vi "Omniax_mDrive_XYZR_MM_BR_RES_2_NC_GR.vi"() -> ()   [LabVIEW 2009]
uses:
  <vilib>/Instr/_visa.llb/VISA Configure Serial Port (Instr).vi
panel:
  out "XY Graph 2":cluster{"Y":dbl[], "Y":dbl[]}[](graph)
  out "XY Graph":cluster{"Y":dbl[], "Y":dbl[]}[](graph)
  out "X Scan Duration":dbl
  out "Y Scan Duration":dbl
  out "Z Scan Duration":dbl
  out "R Scan Duration":dbl
  out "R Backlash steps/sec":i32
  out "R Backlash":i32
  out "R Holding Current %":i32
  out "R Run Current %":i32
  out "R offset deg":dbl
  out "R deg/rev":dbl
  out "R steps/rev":u32
  out "R velocity PV step/sec":i32
  out "R MINPOS":i32=-94296
  out "R MAXPOS":i32=-34296
  out "R COM PORT":refnum<visa-resource-name>="COM5"
  in  "R Scan set":bool
  in  "R Scan Velocity SP deg/sec":dbl
  in  "R Scan Length SP deg":dbl
  in  "R Move Set":bool
  out "Reset R Motor Steps":i32
  in  "Reset R Position deg":dbl
  out "R Velocity MVdeg/sec":dbl
  in  "R Velocity SP deg/sec":dbl
  in  "R Position SP deg":dbl
  out "R Position MV deg":dbl
  out "R Scan velocity MV deg/sec":dbl format="%#_6f"
  out "R Scan length MV deg":dbl
  in  "R Scan Length SP steps":i32 min=0 max=6144000 step=100
  in  "R Scan OK":bool
  in  "R Velocity SP step/sec":i32 min=1 max=102400
  in  "R Scan Velocity SP steps/sec":i32=1 min=1 max=102400 step=1
  in  "R Go":bool
  in  "R Step SP":i32=-20000 min=0 max=6144000 step=500
  out "R Position deg PV":dbl
  out "R Step PV":i32 max=2000
  out "R Backlash corr":bool
  out "R in Motion":bool
  out "R Scan":bool
  out "R in Range":bool
  out "Z COM PORT":refnum<visa-resource-name>="COM5"
  out "Z Backlash steps/sec":i32
  out "Z Backlash":i32
  out "Z Holding Current %":i32
  out "Z Run Current %":i32
  out "Z offset mm":dbl
  out "Z mm/rev":dbl
  out "Z steps/rev":u32
  out "Z  velocity PV step/sec":i32
  out "Z MINPOS":i32=-94296
  out "Z MAXPOS":i32=-34296
  in  "Z Scan set":bool
  in  "Z Scan Velocity SP mm/sec":dbl
  in  "Z Scan Length SP mm":dbl
  in  "Z Move Set":bool
  out "Reset Z Motor Steps":i32
  in  "Reset Z Position mm":dbl
  out "Z Velocity MV mm/sec":dbl
  in  "Z Velocity SP mm/sec":dbl
  in  "Z Position SP mm":dbl
  out "Z Position MV mm":dbl
  out "Z Scan velocity MV mm/sec":dbl format="%#_6f"
  out "Z Scan length MV mm":dbl
  in  "Z Scan Length SP steps":i32 min=0 max=2048000 step=100
  in  "Z Scan OK":bool
  in  "Z Velocity SP step/sec":i32 min=1 max=102400
  in  "Z Scan Velocity SP steps/sec":i32=1 min=1 max=102400 step=1
  in  "Z Go":bool
  in  "Z Step SP":i32=-20000 min=0 max=2048000 step=500
  out "Z Position mm PV":dbl
  out "Z Step PV":i32 max=2000
  out "Z Backlash corr":bool
  out "Z in Motion":bool
  out "Z Scan":bool
  out "Z in Range":bool
  out "Reset X Motor Steps":i32
  in  "Reset X Position mm":dbl
  out "X Backlash corr":bool
  out "X  in Motion":bool
  out "X Scan":bool
  out "X  in Range":bool
  out "X Step PV":i32 max=2000
  out "X Position mm PV":dbl
  out "X velocity PV step/sec":i32
  in  "X Scan set":bool
  in  "X Scan Velocity SP mm/sec":dbl
  in  "X Scan Length SP mm":dbl
  in  "X Move Set":bool
  out "X Velocity MV mm/sec":dbl
  in  "X Velocity SP mm/sec":dbl
  in  "X Position SP mm":dbl
  out "X Position MV mm":dbl
  out "X Scan velocity MV mm/sec":dbl format="%#_6f"
  out "X Scan length MV mm":dbl
  in  "X Scan Length SP steps":i32 min=-460800 max=460800 step=100
  in  "X Scan OK":bool
  in  "X Velocity SP step/sec":i32 min=1 max=102400
  in  "X Scan Velocity SP steps/sec":i32=1 min=1 max=102400 step=1
  in  "X Go":bool
  in  "X Step SP":i32=-20000 min=-460800 max=460800 step=500
  out "X Backlash steps/sec":i32
  out "X Backlash":i32
  out "X Holding Current %":i32
  out "X Run Current %":i32
  out "X offset mm":dbl
  out "X mm/rev":dbl
  out "X steps/rev":u32
  out "X MAXPOS":i32=-34296
  out "X MINPOS":i32=-94296
  out "X COM PORT":refnum<visa-resource-name>="COM5"
  out "Y Backlash corr":bool
  in  "Y Scan set":bool
  in  "Y Scan Velocity SP mm/sec":dbl
  in  "Y Scan Length SP mm":dbl
  in  "Y Move Set":bool
  out "Y Backlash steps/sec":i32
  out "Y Backlash":i32
  out "Y in Motion":bool
  in  "Reset":bool
  out "Reset Y Motor Steps":i32
  in  "Reset Y Position mm":dbl
  out "Y Velocity MV mm/sec":dbl
  in  "Y Velocity SP mm/sec":dbl
  in  "Y Position SP mm":dbl
  out "Y Position MV mm":dbl
  out "Y Holding Current %":i32
  out "Y Run Current %":i32
  out "Y Scan velocity MV mm/sec":dbl format="%#_6f"
  out "Y Scan length MV mm":dbl
  in  "Scan Cancel":bool
  out "Y Position mm PV":dbl
  out "Y offset mm":dbl
  out "Y mm/rev":dbl
  out "Y steps/rev":u32
  out "Y velocity PV step/sec":i32
  in  "Y Scan Length SP steps":i32 min=-460800 max=460800 step=100
  out "Y Scan":bool
  in  "Y Scan OK":bool
  in  "Scan Go":bool
  in  "Y Velocity SP step/sec":i32 min=1 max=102400
  in  "Y Scan Velocity SP steps/sec":i32=1 min=1 max=102400 step=1
  in  "Stop":bool
  out "Y in Range":bool
  out "Y Step PV":i32 max=2000
  in  "Y Go":bool
  in  "Y Step SP":i32=-20000 min=-460800 max=460800 step=500
  out "Y MINPOS":i32=-94296
  out "Y MAXPOS":i32=-34296
  out "Y COM PORT":refnum<visa-resource-name>="COM5"
  # "L"
  # "M"
  # "B"
  # "S"
  # "MX"
  # "MY"
  # "MZ"
  # "MR"
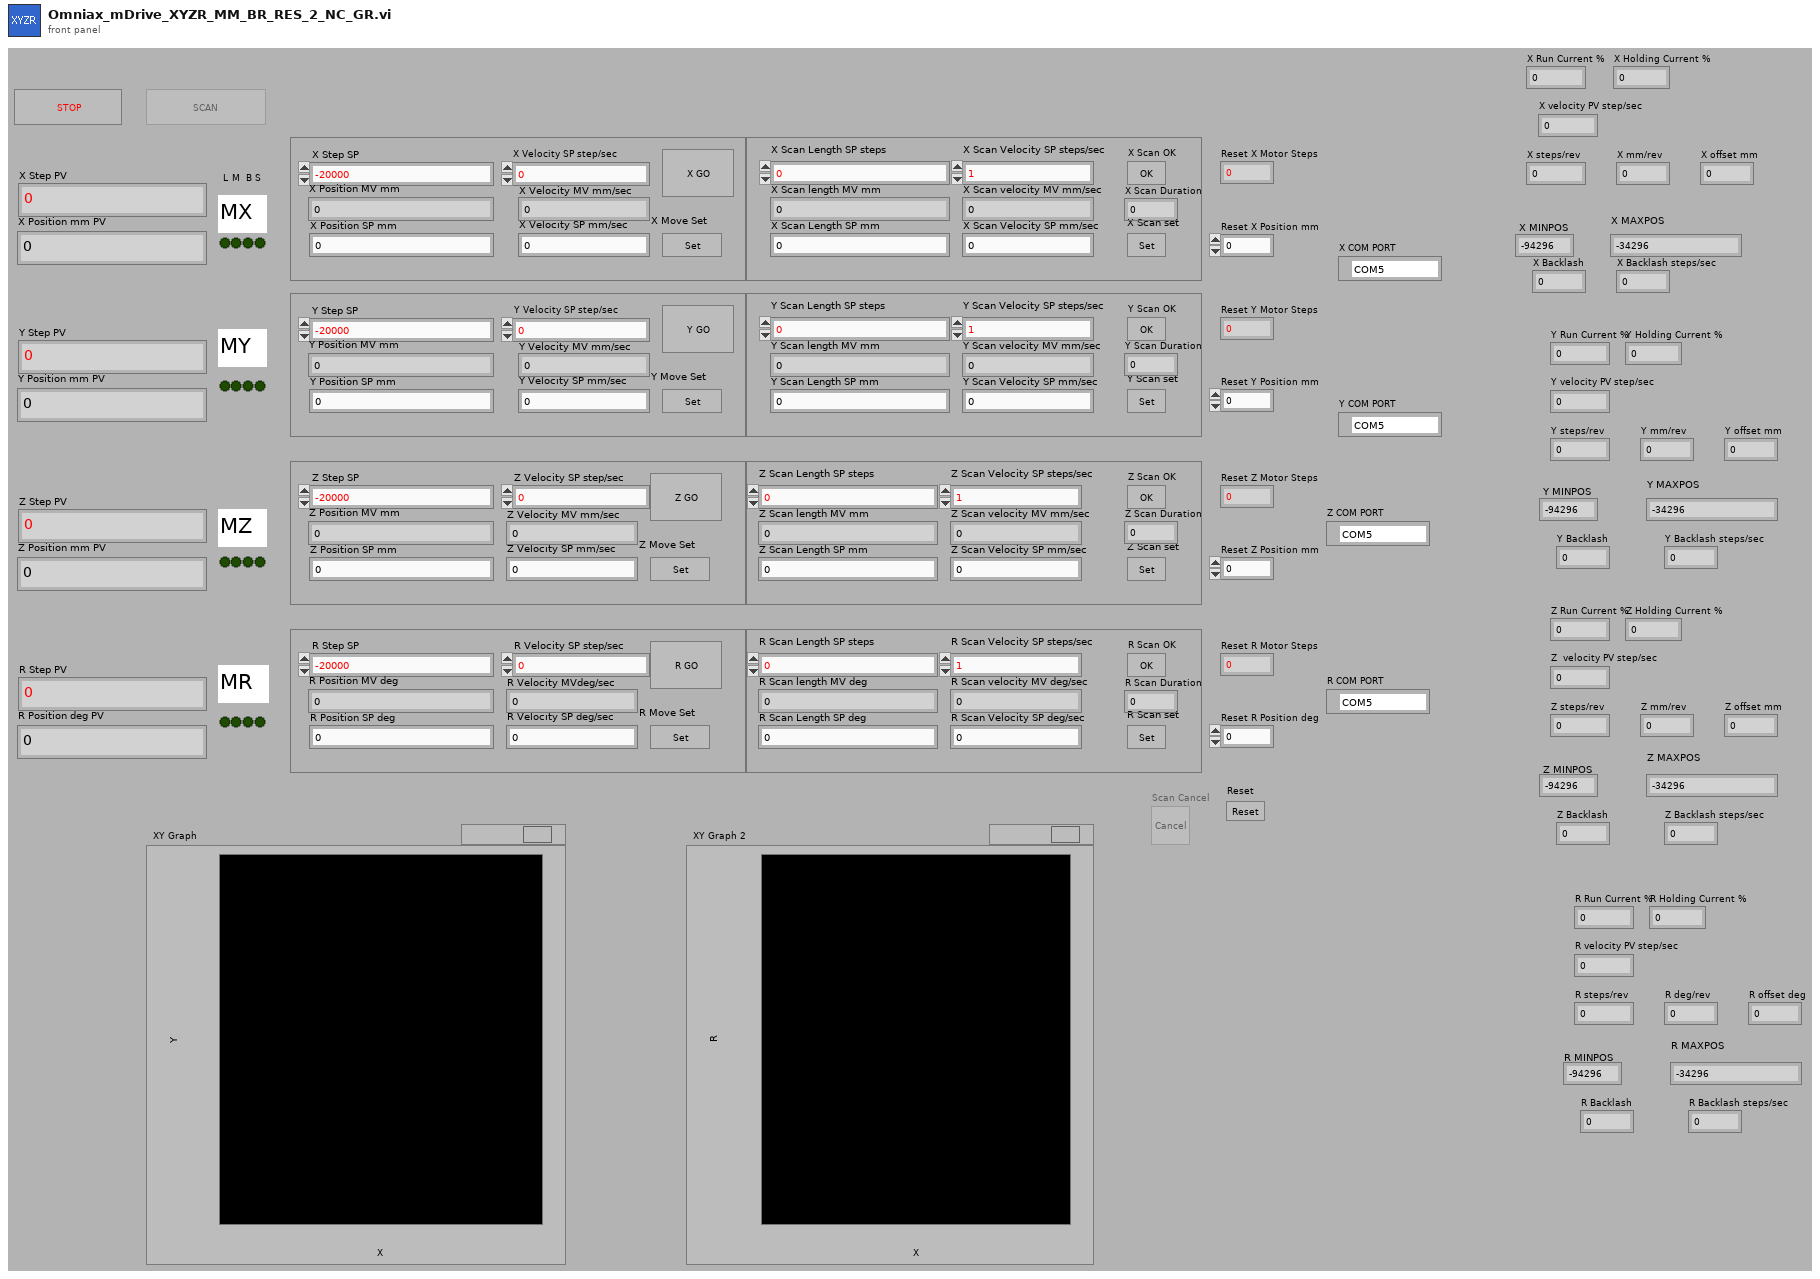
[diagram p1: front panel]
types:
  T1 = enum8{"Enabled", "Disabled", "Disabled and Grayed Out"}
  T2 = enum16{"Stop", "Reset", "Run Current", "Holding Current", "Accel Rate", "Decel Rate", "Move to Relative Position", "Move to Absolute Position", "Echo Mode", "Print Parameter", "Send String", "Microstep Resolution", "Set Current Position", "Max Velocity"}
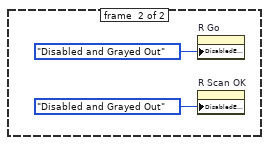
[diagram p2: hidden frame]
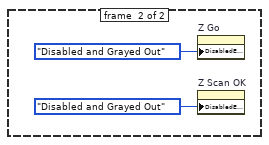
[diagram p5: hidden frame]
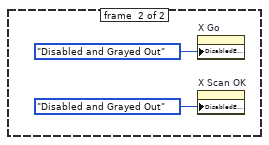
[diagram p8: hidden frame]
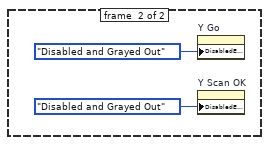
[diagram p11: hidden frame]
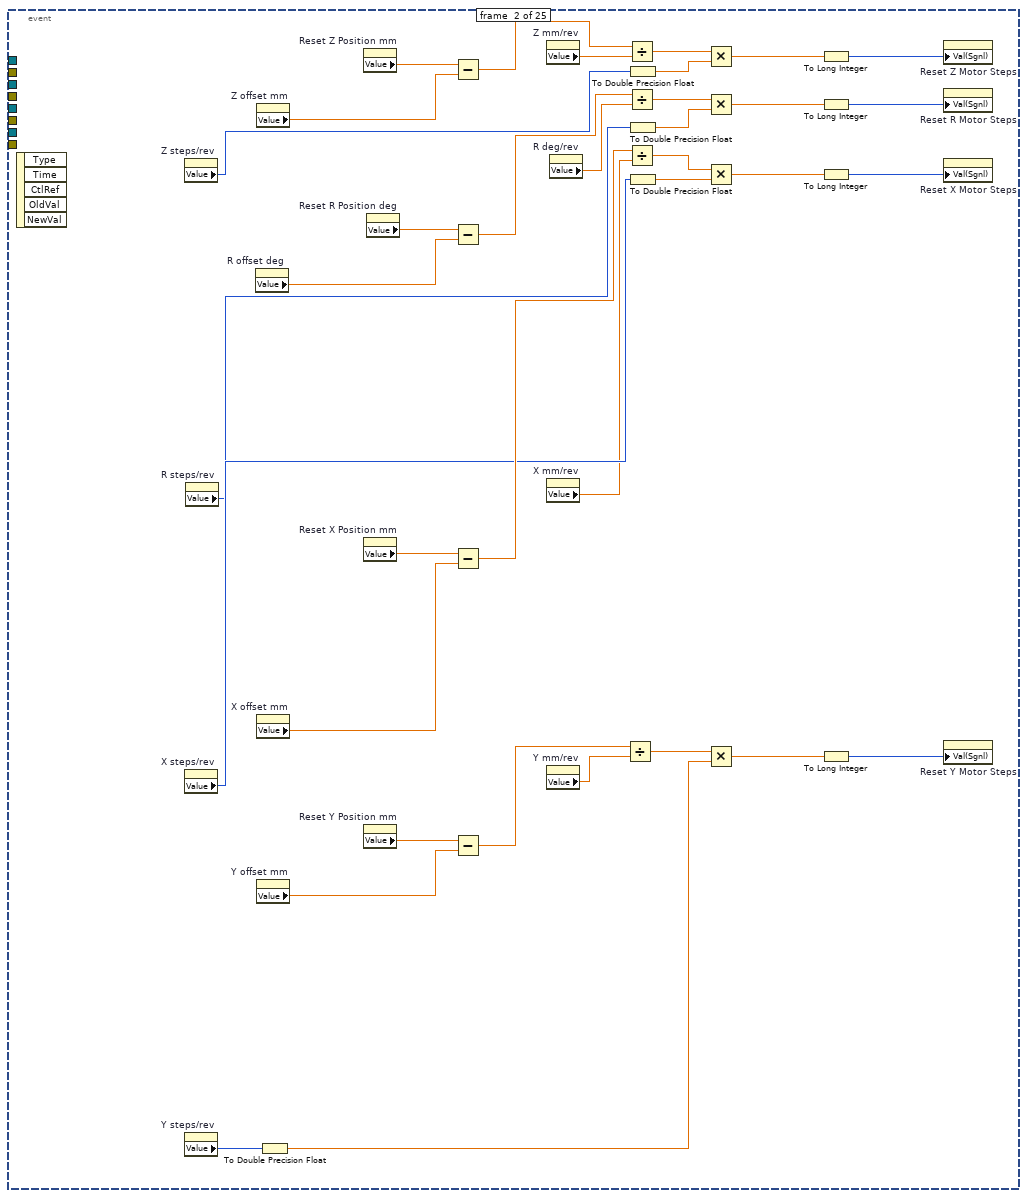
[diagram p14: hidden frame]
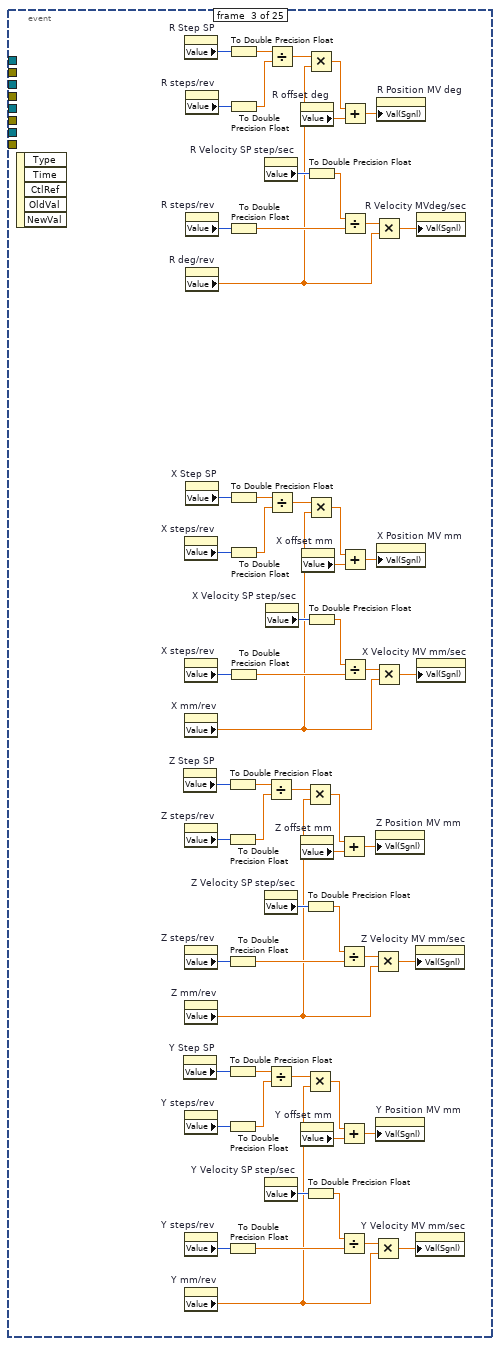
[diagram p15: hidden frame]
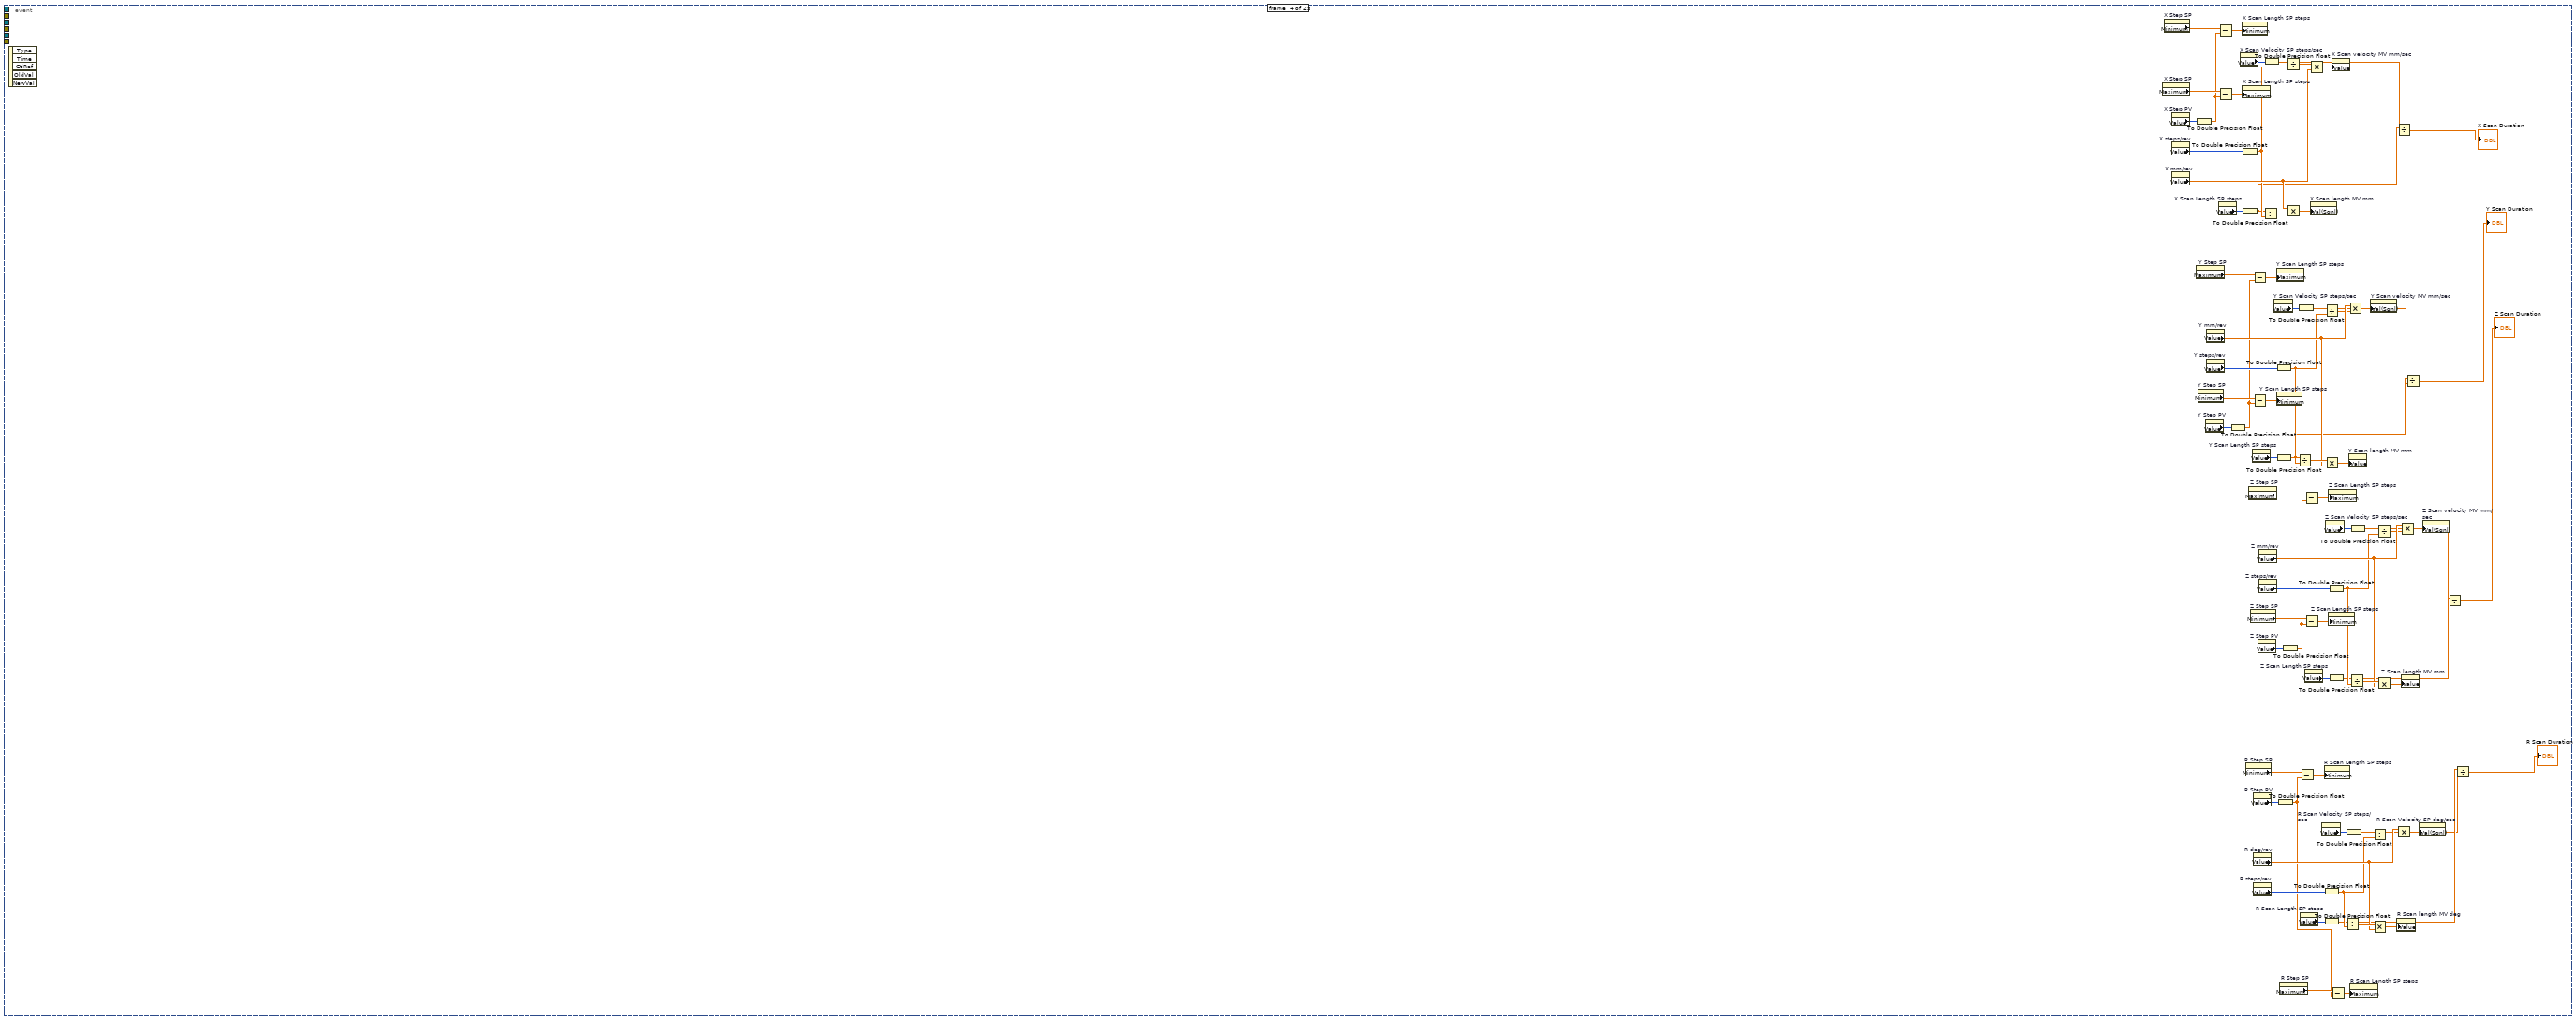
[diagram p16: hidden frame]
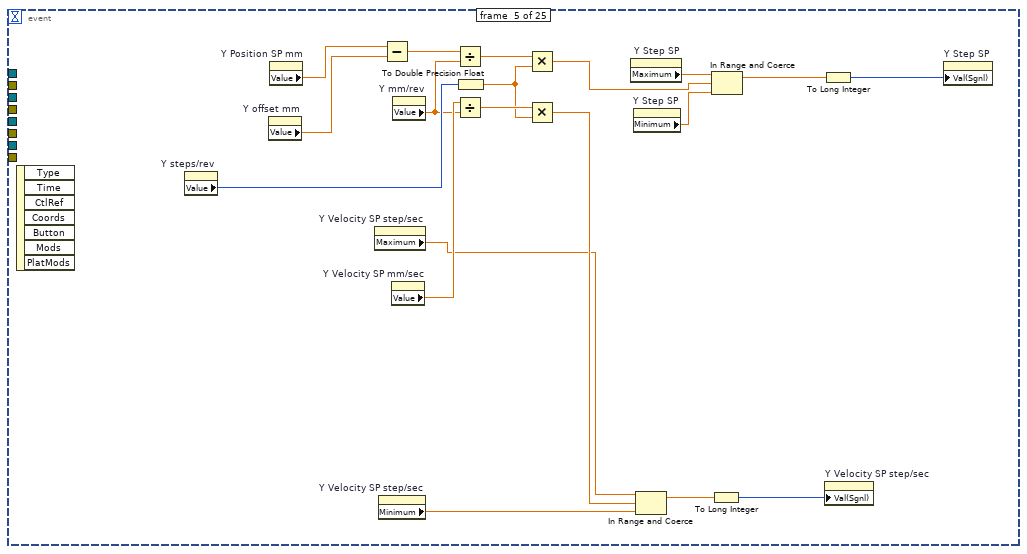
[diagram p17: hidden frame]
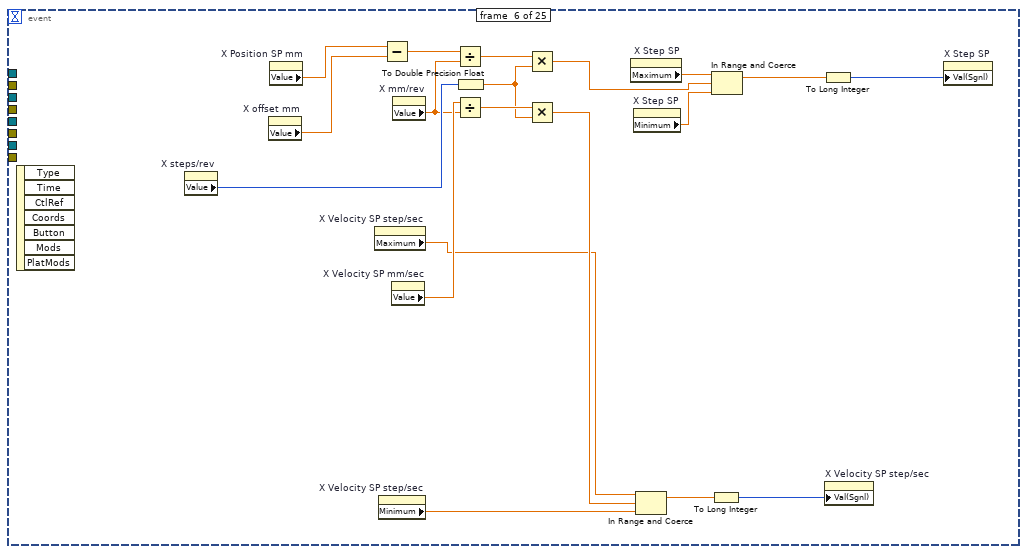
[diagram p18: hidden frame]
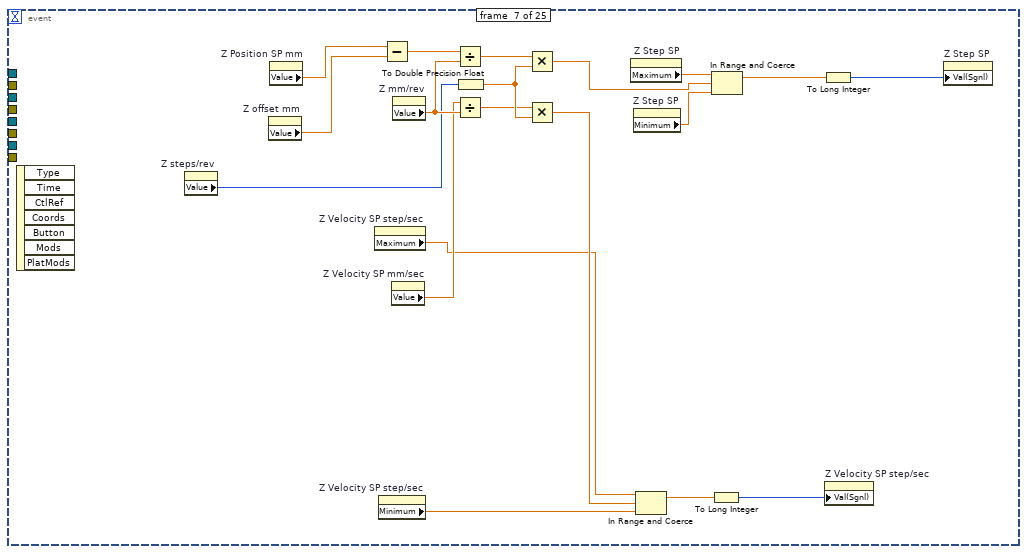
[diagram p19: hidden frame]
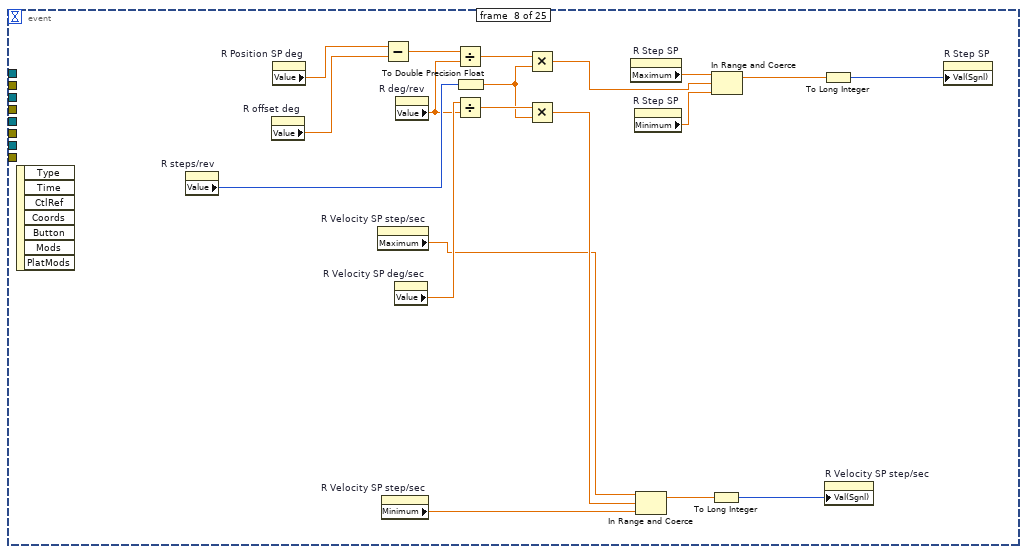
[diagram p20: hidden frame]
diagram:
  w19 = refnum<visa-resource-name> "COM11" ("COM PORT")
  w21 = u16 0 items=["None", "XON/XOFF", "RTS/CTS", "XON/XOFF & RTS/CTS", "DTR/DSR", "XON/XOFF & DTR/DSR"] ("flow control (0:none)")
  w22 = u16 10 items=["1.0"=10, "1.5"=15, "2.0"=20] ("stop bits (10: 1 bit)")
  w52 = refnum<visa-resource-name> "COM10" ("COM PORT")
  w54 = u16 0 items=["None", "XON/XOFF", "RTS/CTS", "XON/XOFF & RTS/CTS", "DTR/DSR", "XON/XOFF & DTR/DSR"] ("flow control (0:none)")
  w55 = u16 10 items=["1.0"=10, "1.5"=15, "2.0"=20] ("stop bits (10: 1 bit)")
  w65 = refnum<visa-resource-name> "COM8" ("COM PORT")
  w67 = u16 0 items=["None", "XON/XOFF", "RTS/CTS", "XON/XOFF & RTS/CTS", "DTR/DSR", "XON/XOFF & DTR/DSR"] ("flow control (0:none)")
  w68 = u16 10 items=["1.0"=10, "1.5"=15, "2.0"=20] ("stop bits (10: 1 bit)")
  w90 = refnum<visa-resource-name> "COM9" ("COM PORT")
  w92 = u16 0 items=["None", "XON/XOFF", "RTS/CTS", "XON/XOFF & RTS/CTS", "DTR/DSR", "XON/XOFF & DTR/DSR"] ("flow control (0:none)")
  w93 = u16 10 items=["1.0"=10, "1.5"=15, "2.0"=20] ("stop bits (10: 1 bit)")
  # "Stop bits"
  # "Stop bits"
  # "Stop bits"
  # "Stop bits"
  n1 = flat-sequence {
    frame #0 {
      w101 = 3.0 ("R deg/rev")
      w99 = u32 51200 ("step/rev")
      w103 = 102400 ("Value (Signaling)")
      n2 = property on="R Velocity SP step/sec" class="DigNum (strict)"("Val(Sgnl)"=w103) -> ()  [unwired: 2 in, 2 out]
      n3 = property on="R Velocity SP step/sec" class="DigNum (strict)"("Minimum"=1.0 ("Data Entry Limits:Minimum")) -> ()  [unwired: 2 in, 2 out]
      n4 = To Double Precision Float(number=w99) -> (double precision float=w100:dbl)
      n5 = To Double Precision Float(number=w103) -> (double precision float=w105:dbl)
      n6 = Divide(x=w105, y=w100) -> (x/y=w104:dbl)
      n7 = property on="R Velocity SP step/sec" class="DigNum (strict)"("Maximum"=w105) -> ()  [unwired: 2 in, 2 out]
      n8 = Multiply(x=w104, y=w101) -> (x*y=w102:dbl)
      n9 = property on="R Velocity SP deg/sec" class="DigNum (strict)"("Val(Sgnl)"=w102) -> ()  [unwired: 2 in, 2 out]
      "R offset deg" <- 0.0 ("R offset deg")
      "R deg/rev" <- w101
      "R steps/rev" <- w99
    }
  }
  n10 = flat-sequence {
    frame #0 {
      w108 = 1.0 ("MM/rev")
      w111 = u32 51200 ("step/rev")
      w106 = 102400 ("Value (Signaling)")
      n11 = property on="X Velocity SP step/sec" class="DigNum (strict)"("Minimum"=1.0 ("Data Entry Limits:Minimum")) -> ()  [unwired: 2 in, 2 out]
      n12 = property on="X Velocity SP step/sec" class="DigNum (strict)"("Val(Sgnl)"=w106) -> ()  [unwired: 2 in, 2 out]
      n13 = To Double Precision Float(number=w111) -> (double precision float=w110:dbl)
      n14 = To Double Precision Float(number=w106) -> (double precision float=w112:dbl)
      n15 = Divide(x=w112, y=w110) -> (x/y=w107:dbl)
      n16 = property on="X Velocity SP step/sec" class="DigNum (strict)"("Maximum"=w112) -> ()  [unwired: 2 in, 2 out]
      n17 = Multiply(x=w107, y=w108) -> (x*y=w109:dbl)
      n18 = property on="X Velocity SP mm/sec" class="DigNum (strict)"("Val(Sgnl)"=w109) -> ()  [unwired: 2 in, 2 out]
      "X offset mm" <- 0.0 ("offset")
      "X steps/rev" <- w111
      "X mm/rev" <- w108
    }
  }
  n19 = flat-sequence {
    frame #0 {
      w116 = 1.0 ("Z mm/rev")
      w115 = u32 51200 ("step/rev")
      w117 = 102400 ("Value (Signaling)")
      n20 = property on="Z Velocity SP step/sec" class="DigNum (strict)"("Val(Sgnl)"=w117) -> ()  [unwired: 2 in, 2 out]
      n21 = property on="Z Velocity SP step/sec" class="DigNum (strict)"("Minimum"=1.0 ("Data Entry Limits:Minimum")) -> ()  [unwired: 2 in, 2 out]
      n22 = To Double Precision Float(number=w115) -> (double precision float=w120:dbl)
      n23 = To Double Precision Float(number=w117) -> (double precision float=w121:dbl)
      n24 = Divide(x=w121, y=w120) -> (x/y=w118:dbl)
      n25 = property on="Z Velocity SP step/sec" class="DigNum (strict)"("Maximum"=w121) -> ()  [unwired: 2 in, 2 out]
      n26 = Multiply(x=w118, y=w116) -> (x*y=w119:dbl)
      n27 = property on="Z Velocity SP mm/sec" class="DigNum (strict)"("Val(Sgnl)"=w119) -> ()  [unwired: 2 in, 2 out]
      "Z offset mm" <- 0.0 ("Z offset mm")
      "Z mm/rev" <- w116
      "Z steps/rev" <- w115
    }
  }
  n28 = flat-sequence {
    frame #0 {
      n29 = property on="X Backlash corr" class="Bool (strict)"("Val(Sgnl)"=FALSE ("Value (Signaling)")) -> ()  [unwired: 2 in, 2 out]
      n30 = property on="Z Backlash corr" class="Bool (strict)"("Val(Sgnl)"=FALSE ("Value (Signaling)")) -> ()  [unwired: 2 in, 2 out]
      n31 = property on="Y Backlash corr" class="Bool (strict)"("Val(Sgnl)"=FALSE ("Value (Signaling)")) -> ()  [unwired: 2 in, 2 out]
      n32 = property on="R Backlash corr" class="Bool (strict)"("Val(Sgnl)"=FALSE ("Value (Signaling)")) -> ()  [unwired: 2 in, 2 out]
      "Z Backlash steps/sec" <- 25600 ("Z Backlash steps/sec")
      "Z Backlash" <- -12800 ("Z Backlash")
      "X Backlash steps/sec" <- 25600 ("Value (Signaling)")
      "X Backlash" <- -5120 ("Backlash2")
      "Y Backlash" <- -5120 ("Backlash2")
      "Y Backlash steps/sec" <- 25600 ("Value (Signaling)")
      "R Backlash steps/sec" <- 25600 ("R Backlash steps/sec")
      "R Backlash" <- -12800 ("R Backlash")
    }
  }
  n33 = flat-sequence {
    frame #0 {
      "Z Holding Current %" <- 20 ("Z Holding Current %")
      "Z Run Current %" <- 40 ("Z Run Current %")
      "X Run Current %" <- 40 ("Run Current %")
      "X Holding Current %" <- 20 ("Holding Current %")
      "Y Run Current %" <- 40 ("Run Current %")
      "Y Holding Current %" <- 20 ("Holding Current %")
      "R Holding Current %" <- 20 ("R Holding Current %")
      "R Run Current %" <- 40 ("R Run Current %")
    }
  }
  n34 = flat-sequence {
    frame #0 {
      n35 = property on="Y Scan" class="Bool (strict)"("Val(Sgnl)"=FALSE ("Value (Signaling)")) -> ()  [unwired: 2 in, 2 out]
      n36 = property on="Y Scan Velocity SP mm/sec" class="DigNum (strict)"("Val(Sgnl)"=0.1 ("Value (Signaling)")) -> ()  [unwired: 2 in, 2 out]
      n37 = property on="Z Scan Velocity SP mm/sec" class="DigNum (strict)"("Val(Sgnl)"=0.1 ("Value (Signaling)")) -> ()  [unwired: 2 in, 2 out]
      n38 = property on="R Scan" class="Bool (strict)"("Val(Sgnl)"=FALSE ("Value (Signaling)")) -> ()  [unwired: 2 in, 2 out]
      n39 = property on="Z Scan" class="Bool (strict)"("Val(Sgnl)"=FALSE ("Value (Signaling)")) -> ()  [unwired: 2 in, 2 out]
      n40 = property on="R Velocity SP deg/sec" class="DigNum (strict)"("Val(Sgnl)"=0.1 ("Value (Signaling)")) -> ()  [unwired: 2 in, 2 out]
      n41 = property on="X Scan" class="Bool (strict)"("Val(Sgnl)"=FALSE ("Value (Signaling)")) -> ()  [unwired: 2 in, 2 out]
      n42 = property on="X Scan Velocity SP mm/sec" class="DigNum (strict)"("Val(Sgnl)"=0.1 ("Value (Signaling)")) -> ()  [unwired: 2 in, 2 out]
      n43 = property on="Scan Go" class="Bool"("DisabledEnum"=T1."Disabled and Grayed Out" ("Disabled")) -> ()  [unwired: 2 in, 2 out]
      n44 = property on="Scan Cancel" class="Bool"("DisabledEnum"=T1."Disabled and Grayed Out" ("Disabled")) -> ()  [unwired: 2 in, 2 out]
    }
  }
  n45 = flat-sequence {
    frame #0 {
      w156 = 1.0 ("MM/rev")
      w159 = u32 51200 ("step/rev")
      w154 = 102400 ("Value (Signaling)")
      n46 = property on="Y Velocity SP step/sec" class="DigNum (strict)"("Minimum"=1.0 ("Data Entry Limits:Minimum")) -> ()  [unwired: 2 in, 2 out]
      n47 = property on="Y Velocity SP step/sec" class="DigNum (strict)"("Val(Sgnl)"=w154) -> ()  [unwired: 2 in, 2 out]
      n48 = To Double Precision Float(number=w159) -> (double precision float=w158:dbl)
      n49 = To Double Precision Float(number=w154) -> (double precision float=w160:dbl)
      n50 = Divide(x=w160, y=w158) -> (x/y=w155:dbl)
      n51 = property on="Y Velocity SP step/sec" class="DigNum (strict)"("Maximum"=w160) -> ()  [unwired: 2 in, 2 out]
      n52 = Multiply(x=w155, y=w156) -> (x*y=w157:dbl)
      n53 = property on="Y Velocity SP mm/sec" class="DigNum (strict)"("Val(Sgnl)"=w157) -> ()  [unwired: 2 in, 2 out]
      "Y offset mm" <- 0.0 ("offset")
      "Y steps/rev" <- w159
      "Y mm/rev" <- w156
    }
  }
  n54 = call-poly "VISA Configure Serial Port"("VISA resource name"=w90, "timeout (10sec)"=u32 10000, "baud rate (9600)"=u32 9600, "data bits (8)"=u16 8, "parity (0:none)"=enum16{"None", "Odd", "Even", "Mark", "Space"}."None", "stop bits (10: 1 bit)"=w93, "flow control (0:none)"=w92) -> ("VISA resource name out"=w83:refnum<visa-resource-name>, "error out"=w82:errorcluster)  [unwired: 7 in]
  n55 = flat-sequence {
    tunnel: w82 -> [w164]
    tunnel: w83 -> [w166]
    tunnel: [w165] -> w4
    tunnel: [w163] -> w3
    tunnel: [w172] -> w81
    tunnel: [w174] -> w79
    tunnel: w4 -> [w173]
    tunnel: w3 -> [w175]
    tunnel: w81 -> [w182]
    tunnel: [w181] -> w80
    tunnel: w79 -> [w179]
    tunnel: [w180] -> w78
    tunnel: [w192] -> w85
    tunnel: [w193] -> w84
    tunnel: w80 -> [w191]
    tunnel: w78 -> [w190]
    tunnel: w85 -> [w203]
    tunnel: w84 -> [w202]
    tunnel: [w205] -> w51
    tunnel: [w204] -> w50
    tunnel: [w199] -> w49
    tunnel: [w210] -> w88
    tunnel: [w211] -> w89
    tunnel: w51 -> [w211]
    tunnel: w50 -> [w210]
    tunnel: w49 -> [w206]
    frame #0 {
      n56 = call "mDrive Send Command.vi"("error in (no error)"=w164, "Extra"="EM=2", "Command"=T2."Send String", "VISA resource name"=w166) -> ("error out"=w163:errorcluster, "VISA resource name out"=w165:refnum<visa-resource-name>)  [unwired: 3 in, 1 out]
    }
    frame #1 {
      # "Run Current %"
      n57 = property on="Y Run Current %" class="DigNum (strict)"() -> ("Value"=w170:i32)  [unwired: 2 in, 2 out]
      n58 = Number To Decimal String(number=w170) -> (decimal integer string=w171:string)  [unwired: 1 in]
      n59 = call "mDrive Send Command.vi"("error in (no error)"=w175, "Extra"=w171, "Command"=T2."Run Current", "VISA resource name"=w173) -> ("error out"=w174:errorcluster, "VISA resource name out"=w172:refnum<visa-resource-name>)  [unwired: 3 in, 1 out]
    }
    frame #2 {
      # "Holding Current %"
      n60 = property on="Y Holding Current %" class="DigNum (strict)"() -> ("Value"=w177:i32)  [unwired: 2 in, 2 out]
      n61 = Number To Decimal String(number=w177) -> (decimal integer string=w178:string)  [unwired: 1 in]
      n62 = call "mDrive Send Command.vi"("error in (no error)"=w179, "Extra"=w178, "Command"=T2."Holding Current", "VISA resource name"=w182) -> ("error out"=w180:errorcluster, "VISA resource name out"=w181:refnum<visa-resource-name>)  [unwired: 3 in, 1 out]
    }
    frame #3 {
      # "Print Velocity Ma"
      # "Velocity Max"
      n63 = property on="Y Velocity SP step/sec" class="DigNum (strict)"() -> ("Value"=w189:i32)  [unwired: 2 in, 2 out]
      n64 = Number To Decimal String(number=w189) -> (decimal integer string=w188:string)  [unwired: 1 in]
      n65 = call "mDrive Send Command.vi"("error in (no error)"=w190, "Extra"=w188, "Command"=T2."Max Velocity", "VISA resource name"=w191) -> ("error out"=w186:errorcluster, "VISA resource name out"=w196:refnum<visa-resource-name>)  [unwired: 3 in, 1 out]
      n66 = call "mDrive Send Command.vi"("error in (no error)"=w186, "Extra"="VM", "Command"=T2."Print Parameter", "VISA resource name"=w196) -> ("error out"=w193:errorcluster, "read buffer"=w194:string, "VISA resource name out"=w192:refnum<visa-resource-name>)  [unwired: 3 in]
      n67 = Decimal String To Number(string=w194, offset=0) -> (number=w187:i32)  [unwired: 1 in, 1 out]
      n68 = property on="Y scan velocity MV step/sec" class="DigNum (strict)"("Val(Sgnl)"=w187) -> ()  [unwired: 2 in, 2 out]
    }
    frame #4 {
      # "PRINT POSITION"
      n69 = call "mDrive Send Command.vi"("error in (no error)"=w202, "Extra"="P", "Command"=T2."Print Parameter", "VISA resource name"=w203) -> ("error out"=w204:errorcluster, "read buffer"=w201:string, "VISA resource name out"=w205:refnum<visa-resource-name>)  [unwired: 3 in]
      n70 = Decimal String To Number(string=w201, offset=0) -> (number=w199:i32)  [unwired: 1 in, 1 out]
    }
    frame #5 {
      w208 = -460800 ("lower limit")
      w209 = 460800 ("upper limit")
      n71 = property on="Y Step SP" class="DigNum (strict)"("Val(Sgnl)"=w206) -> ()  [unwired: 2 in, 2 out]
      n72 = property on="Y Step SP" class="DigNum (strict)"("Maximum"=w209) -> ()  [unwired: 2 in, 2 out]
      n73 = property on="Y Step SP" class="DigNum (strict)"("Minimum"=w208) -> ()  [unwired: 2 in, 2 out]
      n74 = In Range and Coerce(upper limit=w209, x=w206, lower limit=w208) -> (In Range?=w207:bool)  [unwired: 1 out]
      n75 = property on="Y in Range" class="Bool (strict)"("Val(Sgnl)"=w207) -> ()  [unwired: 2 in, 2 out]
      "Y MINPOS" <- w208
      "Y MAXPOS" <- w209
    }
  }
  n76 = call-poly "VISA Configure Serial Port"("VISA resource name"=w65, "timeout (10sec)"=u32 10000, "baud rate (9600)"=u32 9600, "data bits (8)"=u16 8, "parity (0:none)"=enum16{"None", "Odd", "Even", "Mark", "Space"}."None", "stop bits (10: 1 bit)"=w68, "flow control (0:none)"=w67) -> ("VISA resource name out"=w64:refnum<visa-resource-name>, "error out"=w63:errorcluster)  [unwired: 7 in]
  n77 = call-poly "VISA Configure Serial Port"("VISA resource name"=w19, "timeout (10sec)"=u32 10000, "baud rate (9600)"=u32 9600, "data bits (8)"=u16 8, "parity (0:none)"=enum16{"None", "Odd", "Even", "Mark", "Space"}."None", "stop bits (10: 1 bit)"=w22, "flow control (0:none)"=w21) -> ("VISA resource name out"=w18:refnum<visa-resource-name>, "error out"=w17:errorcluster)  [unwired: 7 in]
  n78 = call-poly "VISA Configure Serial Port"("VISA resource name"=w52, "timeout (10sec)"=u32 10000, "baud rate (9600)"=u32 9600, "data bits (8)"=u16 8, "parity (0:none)"=enum16{"None", "Odd", "Even", "Mark", "Space"}."None", "stop bits (10: 1 bit)"=w55, "flow control (0:none)"=w54) -> ("VISA resource name out"=w36:refnum<visa-resource-name>, "error out"=w35:errorcluster)  [unwired: 7 in]
  n79 = flat-sequence {
    tunnel: w63 -> [w213]
    tunnel: w64 -> [w215]
    tunnel: [w214] -> w2
    tunnel: [w212] -> w1
    tunnel: [w221] -> w77
    tunnel: [w223] -> w76
    tunnel: w2 -> [w222]
    tunnel: w1 -> [w224]
    tunnel: w77 -> [w231]
    tunnel: [w230] -> w75
    tunnel: w76 -> [w228]
    tunnel: [w229] -> w74
    tunnel: [w241] -> w73
    tunnel: [w242] -> w72
    tunnel: w75 -> [w240]
    tunnel: w74 -> [w239]
    tunnel: w73 -> [w252]
    tunnel: w72 -> [w251]
    tunnel: [w254] -> w48
    tunnel: [w253] -> w47
    tunnel: [w248] -> w46
    tunnel: [w259] -> w61
    tunnel: [w260] -> w62
    tunnel: w48 -> [w260]
    tunnel: w47 -> [w259]
    tunnel: w46 -> [w255]
    frame #0 {
      n80 = call "mDrive Send Command.vi"("error in (no error)"=w213, "Extra"="EM=2", "Command"=T2."Send String", "VISA resource name"=w215) -> ("error out"=w212:errorcluster, "VISA resource name out"=w214:refnum<visa-resource-name>)  [unwired: 3 in, 1 out]
    }
    frame #1 {
      # "Run Current %"
      n81 = property on="X Run Current %" class="DigNum (strict)"() -> ("Value"=w219:i32)  [unwired: 2 in, 2 out]
      n82 = Number To Decimal String(number=w219) -> (decimal integer string=w220:string)  [unwired: 1 in]
      n83 = call "mDrive Send Command.vi"("error in (no error)"=w224, "Extra"=w220, "Command"=T2."Run Current", "VISA resource name"=w222) -> ("error out"=w223:errorcluster, "VISA resource name out"=w221:refnum<visa-resource-name>)  [unwired: 3 in, 1 out]
    }
    frame #2 {
      # "Holding Current %"
      n84 = property on="X Holding Current %" class="DigNum (strict)"() -> ("Value"=w226:i32)  [unwired: 2 in, 2 out]
      n85 = Number To Decimal String(number=w226) -> (decimal integer string=w227:string)  [unwired: 1 in]
      n86 = call "mDrive Send Command.vi"("error in (no error)"=w228, "Extra"=w227, "Command"=T2."Holding Current", "VISA resource name"=w231) -> ("error out"=w229:errorcluster, "VISA resource name out"=w230:refnum<visa-resource-name>)  [unwired: 3 in, 1 out]
    }
    frame #3 {
      # "Print Velocity Ma"
      # "Velocity Max"
      n87 = property on="X Velocity SP step/sec" class="DigNum (strict)"() -> ("Value"=w238:i32)  [unwired: 2 in, 2 out]
      n88 = Number To Decimal String(number=w238) -> (decimal integer string=w237:string)  [unwired: 1 in]
      n89 = call "mDrive Send Command.vi"("error in (no error)"=w239, "Extra"=w237, "Command"=T2."Max Velocity", "VISA resource name"=w240) -> ("error out"=w235:errorcluster, "VISA resource name out"=w245:refnum<visa-resource-name>)  [unwired: 3 in, 1 out]
      n90 = call "mDrive Send Command.vi"("error in (no error)"=w235, "Extra"="VM", "Command"=T2."Print Parameter", "VISA resource name"=w245) -> ("error out"=w242:errorcluster, "read buffer"=w243:string, "VISA resource name out"=w241:refnum<visa-resource-name>)  [unwired: 3 in]
      n91 = Decimal String To Number(string=w243, offset=0) -> (number=w236:i32)  [unwired: 1 in, 1 out]
      n92 = property on="X velocity PV step/sec" class="DigNum (strict)"("Val(Sgnl)"=w236) -> ()  [unwired: 2 in, 2 out]
    }
    frame #4 {
      # "PRINT POSITION"
      n93 = call "mDrive Send Command.vi"("error in (no error)"=w251, "Extra"="P", "Command"=T2."Print Parameter", "VISA resource name"=w252) -> ("error out"=w253:errorcluster, "read buffer"=w250:string, "VISA resource name out"=w254:refnum<visa-resource-name>)  [unwired: 3 in]
      n94 = Decimal String To Number(string=w250, offset=0) -> (number=w248:i32)  [unwired: 1 in, 1 out]
    }
    frame #5 {
      w257 = -460800 ("lower limit")
      w258 = 460800 ("upper limit")
      n95 = property on="X Step SP" class="DigNum (strict)"("Val(Sgnl)"=w255) -> ()  [unwired: 2 in, 2 out]
      n96 = property on="X Step SP" class="DigNum (strict)"("Maximum"=w258) -> ()  [unwired: 2 in, 2 out]
      n97 = property on="X Step SP" class="DigNum (strict)"("Minimum"=w257) -> ()  [unwired: 2 in, 2 out]
      n98 = In Range and Coerce(upper limit=w258, x=w255, lower limit=w257) -> (In Range?=w256:bool)  [unwired: 1 out]
      n99 = property on="X  in Range" class="Bool (strict)"("Val(Sgnl)"=w256) -> ()  [unwired: 2 in, 2 out]
      "X MINPOS" <- w257
      "X MAXPOS" <- w258
    }
  }
  n100 = flat-sequence {
    tunnel: w17 -> [w264]
    tunnel: w18 -> [w262]
    tunnel: [w261] -> w8
    tunnel: [w263] -> w7
    tunnel: [w271] -> w34
    tunnel: [w273] -> w33
    tunnel: w8 -> [w272]
    tunnel: w7 -> [w267]
    tunnel: w34 -> [w280]
    tunnel: [w279] -> w32
    tunnel: w33 -> [w277]
    tunnel: [w278] -> w31
    tunnel: [w290] -> w30
    tunnel: [w291] -> w29
    tunnel: w32 -> [w289]
    tunnel: w31 -> [w288]
    tunnel: w30 -> [w301]
    tunnel: w29 -> [w300]
    tunnel: [w303] -> w28
    tunnel: [w302] -> w27
    tunnel: [w297] -> w26
    tunnel: [w308] -> w11
    tunnel: [w309] -> w12
    tunnel: w28 -> [w309]
    tunnel: w27 -> [w308]
    tunnel: w26 -> [w306]
    frame #0 {
      n101 = call "mDrive Send Command.vi"("error in (no error)"=w264, "Extra"="EM=2", "Command"=T2."Send String", "VISA resource name"=w262) -> ("error out"=w263:errorcluster, "VISA resource name out"=w261:refnum<visa-resource-name>)  [unwired: 3 in, 1 out]
    }
    frame #1 {
      # "Run Current %"
      n102 = property on="R Run Current %" class="DigNum (strict)"() -> ("Value"=w269:i32)  [unwired: 2 in, 2 out]
      n103 = Number To Decimal String(number=w269) -> (decimal integer string=w270:string)  [unwired: 1 in]
      n104 = call "mDrive Send Command.vi"("error in (no error)"=w267, "Extra"=w270, "Command"=T2."Run Current", "VISA resource name"=w272) -> ("error out"=w273:errorcluster, "VISA resource name out"=w271:refnum<visa-resource-name>)  [unwired: 3 in, 1 out]
    }
    frame #2 {
      # "Holding Current %"
      n105 = property on="R Holding Current %" class="DigNum (strict)"() -> ("Value"=w275:i32)  [unwired: 2 in, 2 out]
      n106 = Number To Decimal String(number=w275) -> (decimal integer string=w276:string)  [unwired: 1 in]
      n107 = call "mDrive Send Command.vi"("error in (no error)"=w277, "Extra"=w276, "Command"=T2."Holding Current", "VISA resource name"=w280) -> ("error out"=w278:errorcluster, "VISA resource name out"=w279:refnum<visa-resource-name>)  [unwired: 3 in, 1 out]
    }
    frame #3 {
      # "Print Velocity Ma"
      # "Velocity Max"
      n108 = property on="R Velocity SP step/sec" class="DigNum (strict)"() -> ("Value"=w287:i32)  [unwired: 2 in, 2 out]
      n109 = Number To Decimal String(number=w287) -> (decimal integer string=w286:string)  [unwired: 1 in]
      n110 = call "mDrive Send Command.vi"("error in (no error)"=w288, "Extra"=w286, "Command"=T2."Max Velocity", "VISA resource name"=w289) -> ("error out"=w284:errorcluster, "VISA resource name out"=w294:refnum<visa-resource-name>)  [unwired: 3 in, 1 out]
      n111 = call "mDrive Send Command.vi"("error in (no error)"=w284, "Extra"="VM", "Command"=T2."Print Parameter", "VISA resource name"=w294) -> ("error out"=w291:errorcluster, "read buffer"=w292:string, "VISA resource name out"=w290:refnum<visa-resource-name>)  [unwired: 3 in]
      n112 = Decimal String To Number(string=w292, offset=0) -> (number=w285:i32)  [unwired: 1 in, 1 out]
      n113 = property on="R velocity PV step/sec" class="DigNum (strict)"("Val(Sgnl)"=w285) -> ()  [unwired: 2 in, 2 out]
    }
    frame #4 {
      # "PRINT POSITION"
      n114 = call "mDrive Send Command.vi"("error in (no error)"=w300, "Extra"="P", "Command"=T2."Print Parameter", "VISA resource name"=w301) -> ("error out"=w302:errorcluster, "read buffer"=w299:string, "VISA resource name out"=w303:refnum<visa-resource-name>)  [unwired: 3 in]
      n115 = Decimal String To Number(string=w299, offset=0) -> (number=w297:i32)  [unwired: 1 in, 1 out]
    }
    frame #5 {
      w305 = 0 ("lower limit")
      w304 = 6144000 ("upper limit")
      n116 = property on="R Step SP" class="DigNum (strict)"("Val(Sgnl)"=w306) -> ()  [unwired: 2 in, 2 out]
      n117 = property on="R Step SP" class="DigNum (strict)"("Maximum"=w304) -> ()  [unwired: 2 in, 2 out]
      n118 = property on="R Step SP" class="DigNum (strict)"("Minimum"=w305) -> ()  [unwired: 2 in, 2 out]
      n119 = In Range and Coerce(upper limit=w304, x=w306, lower limit=w305) -> (In Range?=w307:bool)  [unwired: 1 out]
      n120 = property on="R in Range" class="Bool (strict)"("Val(Sgnl)"=w307) -> ()  [unwired: 2 in, 2 out]
      "R MINPOS" <- w305
      "R MAXPOS" <- w304
    }
  }
  n121 = flat-sequence {
    tunnel: w35 -> [w310]
    tunnel: w36 -> [w313]
    tunnel: [w312] -> w6
    tunnel: [w311] -> w5
    tunnel: [w319] -> w45
    tunnel: [w321] -> w44
    tunnel: w6 -> [w320]
    tunnel: w5 -> [w322]
    tunnel: w45 -> [w329]
    tunnel: [w328] -> w43
    tunnel: w44 -> [w326]
    tunnel: [w327] -> w42
    tunnel: [w339] -> w41
    tunnel: [w340] -> w40
    tunnel: w43 -> [w338]
    tunnel: w42 -> [w337]
    tunnel: w41 -> [w350]
    tunnel: w40 -> [w349]
    tunnel: [w352] -> w39
    tunnel: [w351] -> w38
    tunnel: [w346] -> w37
    tunnel: [w357] -> w15
    tunnel: [w358] -> w16
    tunnel: w39 -> [w358]
    tunnel: w38 -> [w357]
    tunnel: w37 -> [w355]
    frame #0 {
      n122 = call "mDrive Send Command.vi"("error in (no error)"=w310, "Extra"="EM=2", "Command"=T2."Send String", "VISA resource name"=w313) -> ("error out"=w311:errorcluster, "VISA resource name out"=w312:refnum<visa-resource-name>)  [unwired: 3 in, 1 out]
    }
    frame #1 {
      # "Run Current %"
      n123 = property on="Z Run Current %" class="DigNum (strict)"() -> ("Value"=w317:i32)  [unwired: 2 in, 2 out]
      n124 = Number To Decimal String(number=w317) -> (decimal integer string=w318:string)  [unwired: 1 in]
      n125 = call "mDrive Send Command.vi"("error in (no error)"=w322, "Extra"=w318, "Command"=T2."Run Current", "VISA resource name"=w320) -> ("error out"=w321:errorcluster, "VISA resource name out"=w319:refnum<visa-resource-name>)  [unwired: 3 in, 1 out]
    }
    frame #2 {
      # "Holding Current %"
      n126 = property on="Z Run Current %" class="DigNum (strict)"() -> ("Value"=w324:i32)  [unwired: 2 in, 2 out]
      n127 = Number To Decimal String(number=w324) -> (decimal integer string=w325:string)  [unwired: 1 in]
      n128 = call "mDrive Send Command.vi"("error in (no error)"=w326, "Extra"=w325, "Command"=T2."Holding Current", "VISA resource name"=w329) -> ("error out"=w327:errorcluster, "VISA resource name out"=w328:refnum<visa-resource-name>)  [unwired: 3 in, 1 out]
    }
    frame #3 {
      # "Print Velocity Ma"
      # "Velocity Max"
      n129 = property on="Z Velocity SP step/sec" class="DigNum (strict)"() -> ("Value"=w336:i32)  [unwired: 2 in, 2 out]
      n130 = Number To Decimal String(number=w336) -> (decimal integer string=w335:string)  [unwired: 1 in]
      n131 = call "mDrive Send Command.vi"("error in (no error)"=w337, "Extra"=w335, "Command"=T2."Max Velocity", "VISA resource name"=w338) -> ("error out"=w333:errorcluster, "VISA resource name out"=w343:refnum<visa-resource-name>)  [unwired: 3 in, 1 out]
      n132 = call "mDrive Send Command.vi"("error in (no error)"=w333, "Extra"="VM", "Command"=T2."Print Parameter", "VISA resource name"=w343) -> ("error out"=w340:errorcluster, "read buffer"=w341:string, "VISA resource name out"=w339:refnum<visa-resource-name>)  [unwired: 3 in]
      n133 = Decimal String To Number(string=w341, offset=0) -> (number=w334:i32)  [unwired: 1 in, 1 out]
      n134 = property on="Z  velocity PV step/sec" class="DigNum (strict)"("Val(Sgnl)"=w334) -> ()  [unwired: 2 in, 2 out]
    }
    frame #4 {
      # "PRINT POSITION"
      n135 = call "mDrive Send Command.vi"("error in (no error)"=w349, "Extra"="P", "Command"=T2."Print Parameter", "VISA resource name"=w350) -> ("error out"=w351:errorcluster, "read buffer"=w348:string, "VISA resource name out"=w352:refnum<visa-resource-name>)  [unwired: 3 in]
      n136 = Decimal String To Number(string=w348, offset=0) -> (number=w346:i32)  [unwired: 1 in, 1 out]
    }
    frame #5 {
      w353 = 0 ("lower limit")
      w354 = 2048000 ("upper limit")
      n137 = property on="Z Step SP" class="DigNum (strict)"("Val(Sgnl)"=w355) -> ()  [unwired: 2 in, 2 out]
      n138 = property on="Z Step SP" class="DigNum (strict)"("Maximum"=w354) -> ()  [unwired: 2 in, 2 out]
      n139 = property on="Z Step SP" class="DigNum (strict)"("Minimum"=w353) -> ()  [unwired: 2 in, 2 out]
      n140 = In Range and Coerce(upper limit=w354, x=w355, lower limit=w353) -> (In Range?=w356:bool)  [unwired: 1 out]
      n141 = property on="Z in Range" class="Bool (strict)"("Val(Sgnl)"=w356) -> ()  [unwired: 2 in, 2 out]
      "Z MINPOS" <- w353
      "Z MAXPOS" <- w354
    }
  }
  n142 = while {
    tunnel: w89 -> [w372]
    tunnel: w88 -> [w375]
    tunnel: [w376] -> w86
    tunnel: [w374] -> w87
    tunnel: w62 -> [w370]
    tunnel: w61 -> [w369]
    tunnel: [w368] -> w60
    tunnel: [w367] -> w59
    tunnel: w16 -> [w366]
    tunnel: w15 -> [w365]
    tunnel: [w364] -> w14
    tunnel: [w363] -> w13
    tunnel: w12 -> [w362]
    tunnel: w11 -> [w361]
    tunnel: [w360] -> w10
    tunnel: [w359] -> w9
    stop <- w371 stop-if-true
    n143 = flat-sequence {
      frame #0 {
      }
    }
    n144 = flat-sequence {
      frame #0 {
      }
    }
    n145 = flat-sequence {
      frame #0 {
      }
    }
    n146 = flat-sequence {
      frame #0 {
      }
    }
    n147 = flat-sequence {
      frame #0 {
      }
    }
    n148 = event shown="[0] Timeout" {
      selector: _ -> [_ _ _ _ _ _ _ _ _ _ _ _ _ _ _ _ _ _ _ _ _ _ _ _ _]
      dyn-events: _ -> [_ _ _ _ _ _ _ _ _ _ _ _ _ _ _ _ _ _ _ _ _ _ _ _ _]
      timeout: 200 -> [_ _ _ _ _ _ _ _ _ _ _ _ _ _ _ _ _ _ _ _ _ _ _ _ _]
      tunnel: w375 -> [w442 _ _ _ _ _ _ _ _ _ _ _ w1267 _ _ _ _ w1516 _ _ w1612 w1628 w1672 w1749 w1993]
      tunnel: [w441 _ _ _ _ _ _ _ _ _ _ _ w1273 _ _ _ _ w1514 _ _ w1612 w1626 w1674 w1738 w1991] -> w376
      tunnel: w372 -> [w439 _ _ _ _ _ _ _ _ _ _ _ w1268 _ _ _ _ w1515 _ _ w1613 w1629 w1673 w1751 w1994]
      tunnel: [w440 _ _ _ _ _ _ _ _ _ _ _ w1274 _ _ _ _ w1511 _ _ w1613 w1627 w1675 w1739 w1992] -> w374
      tunnel: [_ _ _ _ _ _ _ _ _ _ _ _ _ _ _ _ _ _ _ _ TRUE _ _ _ _] -> w371
      tunnel: w370 -> [w416 _ _ _ _ _ _ _ _ _ _ _ _ _ _ w1425 w1480 _ _ _ _ w1623 w1665 w1755 w1990]
      tunnel: w369 -> [w415 _ _ _ _ _ _ _ _ _ _ _ _ _ _ w1424 w1479 _ _ _ _ w1622 w1664 w1753 w1989]
      tunnel: [w414 _ _ _ _ _ _ _ _ _ _ _ _ _ _ w1423 w1478 _ _ _ _ w1625 w1663 w1731 w1988] -> w368
      tunnel: [w413 _ _ _ _ _ _ _ _ _ _ _ _ _ _ w1422 w1477 _ _ _ _ w1624 w1662 w1729 w1987] -> w367
      tunnel: w366 -> [w387 _ _ _ _ _ _ _ _ _ _ _ _ w1319 _ _ _ _ w1546 _ _ w1621 w1659 w1747 w1986]
      tunnel: w365 -> [w390 _ _ _ _ _ _ _ _ _ _ _ _ w1318 _ _ _ _ w1545 _ _ w1620 w1658 w1745 w1985]
      tunnel: [w389 _ _ _ _ _ _ _ _ _ _ _ _ w1316 _ _ _ _ w1543 _ _ w1619 w1657 w1737 w1982] -> w364
      tunnel: [w388 _ _ _ _ _ _ _ _ _ _ _ _ w1317 _ _ _ _ w1544 _ _ w1618 w1656 w1736 w1981] -> w363
      tunnel: w362 -> [w386 _ _ _ _ _ _ _ _ _ _ _ _ _ w1372 _ _ _ _ w1580 _ w1617 w1653 w1742 w1984]
      tunnel: w361 -> [w385 _ _ _ _ _ _ _ _ _ _ _ _ _ w1371 _ _ _ _ w1579 _ w1616 w1652 w1740 w1983]
      tunnel: [w384 _ _ _ _ _ _ _ _ _ _ _ _ _ w1369 _ _ _ _ w1578 _ w1615 w1651 w1734 w1980] -> w360
      tunnel: [w383 _ _ _ _ _ _ _ _ _ _ _ _ _ w1370 _ _ _ _ w1577 _ w1614 w1650 w1733 w1979] -> w359
      event #0 {
        n149 = event-data() -> ()  [unwired: 1 in, 2 out]
        n150 = flat-sequence {
          tunnel: w442 -> [w854]
          tunnel: w439 -> [w853]
          tunnel: [w859] -> w438
          tunnel: [w833] -> w436
          tunnel: [w846] -> w434
          tunnel: [w824] -> w432
          tunnel: w438 -> [w865]
          tunnel: [w865] -> w437
          tunnel: w436 -> [w864]
          tunnel: [w864] -> w435
          tunnel: w434 -> [w863]
          tunnel: [w863] -> w433
          tunnel: w432 -> [w860]
          tunnel: [w860] -> w428
          tunnel: w437 -> [w872]
          tunnel: [w873] -> w431
          tunnel: w435 -> [w875]
          tunnel: [w874] -> w430
          tunnel: w433 -> [w871]
          tunnel: [w870] -> w429
          tunnel: w428 -> [w870]
          tunnel: w431 -> [w885]
          tunnel: w430 -> [w886]
          tunnel: w429 -> [w888]
          tunnel: [w884] -> w441
          tunnel: [w883] -> w440
          frame #0 {
            w828 = 0.05 ("Delay Time (s)")
            n151 = property on="Y Step SP" class="DigNum (strict)"() -> ("Maximum"=w848:dbl)  [unwired: 2 in, 2 out]
            n152 = property on="Y Step SP" class="DigNum (strict)"() -> ("Minimum"=w850:dbl)  [unwired: 2 in, 2 out]
            n153 = property on="Y steps/rev" class="DigNum (strict)"() -> ("Value"=w844:u32)  [unwired: 2 in, 2 out]
            n154 = property on="Y offset mm" class="DigNum (strict)"() -> ("Value"=w840:dbl)  [unwired: 2 in, 2 out]
            n155 = To Long Integer(number=w848) -> (32bit integer=w847:i32)
            n156 = To Long Integer(number=w850) -> (32bit integer=w849:i32)
            n157 = To Double Precision Float(number=w844) -> (double precision float=w845:dbl)
            n158 = call "mDrive Send Command.vi"("error in (no error)"=w854, "Extra"="P", "Command"=T2."Print Parameter", "VISA resource name"=w853) -> ("error out"=w852:errorcluster, "read buffer"=w858:string, "VISA resource name out"=w856:refnum<visa-resource-name>)  [unwired: 3 in]
            n159 = call "Time Delay4"("error in (no error)"=w852, "Delay Time (s)"=w828) -> ("error out"=w851:errorcluster)  [unwired: 9 in]
            n160 = Decimal String To Number(string=w858, offset=0) -> (number=w836:i32)  [unwired: 1 in, 1 out]
            n161 = To Long Integer(number=w836) -> (32bit integer=w838:i32)
            n162 = property on="Y Step PV" class="DigNum (strict)"("Val(Sgnl)"=w838) -> ()  [unwired: 2 in, 2 out]
            n163 = call "mDrive Send Command.vi"("error in (no error)"=w851, "Extra"="MV", "Command"=T2."Print Parameter", "VISA resource name"=w856) -> ("error out"=w855:errorcluster, "read buffer"=w834:string, "VISA resource name out"=w859:refnum<visa-resource-name>)  [unwired: 3 in]
            n164 = call "Time Delay3"("error in (no error)"=w855, "Delay Time (s)"=w828) -> ("error out"=w833:errorcluster)  [unwired: 9 in]
            n165 = In Range and Coerce(upper limit=w847, x=w838, lower limit=w849) -> (In Range?=w846:bool)  [unwired: 1 out]
            n166 = To Double Precision Float(number=w838) -> (double precision float=w839:dbl)
            n167 = Decimal String To Number(string=w834, offset=0 ("offset (0)")) -> (number=w827:i32)  [unwired: 1 in, 1 out]
            n168 = property on="Y in Range" class="Bool (strict)"("Val(Sgnl)"=w846) -> ()  [unwired: 2 in, 2 out]
            n169 = Divide(x=w839, y=w845) -> (x/y=w843:dbl)
            n170 = Number To Boolean Array(number=w827) -> (Boolean array=w826:bool[])
            n171 = property on="Y mm/rev" class="DigNum (strict)"() -> ("Value"=w842:dbl)  [unwired: 2 in, 2 out]
            n172 = Index Array(array=w826, index=0) -> (element=w824:bool)
            n173 = property on="Y in Motion" class="Bool (strict)"("Val(Sgnl)"=w824) -> ()  [unwired: 2 in, 2 out]
            n174 = Multiply(x=w843, y=w842) -> (x*y=w841:dbl)
            n175 = Add(x=w841, y=w840) -> (x+y=w837:dbl)
            n176 = property on="Y Position mm PV" class="DigNum (strict)"("Val(Sgnl)"=w837) -> ()  [unwired: 2 in, 2 out]
          }
          frame #1 {
            n177 = property on="Y Scan" class="Bool (strict)"() -> ("Value"=w861:bool)  [unwired: 2 in, 2 out]
            n178 = Or(x=w860, y=w861) -> (x .or. y?=w862:bool)
            n179 = case shown="True" w862 {
              frame #0 {
                n180 = property on="Y Go" class="Bool"("DisabledEnum"=T1."Enabled" ("Disabled")) -> ()  [unwired: 2 in, 2 out]
                n181 = property on="Y Scan OK" class="Bool"("DisabledEnum"=T1."Enabled" ("Disabled")) -> ()  [unwired: 2 in, 2 out]
              }
              frame #1 {
                n182 = property on="Y Go" class="Bool"("DisabledEnum"=T1."Disabled and Grayed Out" ("Disabled")) -> ()  [unwired: 2 in, 2 out]
                n183 = property on="Y Scan OK" class="Bool"("DisabledEnum"=T1."Disabled and Grayed Out" ("Disabled")) -> ()  [unwired: 2 in, 2 out]
              }
            }
          }
          frame #2 {
            n184 = case shown="False" w871 {
              tunnel: w872 -> [w878 w882]
              tunnel: [w879 w882] -> w873
              tunnel: [w880 w881] -> w874
              tunnel: w875 -> [w877 w881]
              frame #0 {
                n185 = call "mDrive Send Command.vi"("error in (no error)"=w877, "Command"=T2."Stop", "VISA resource name"=w878) -> ("error out"=w880:errorcluster, "VISA resource name out"=w879:refnum<visa-resource-name>)  [unwired: 4 in, 1 out]
              }
              frame #1 {
              }
            }
          }
          frame #3 {
            n186 = property on="Y Backlash corr" class="Bool (strict)"() -> ("Value"=w889:bool)  [unwired: 2 in, 2 out]
            n187 = Implies(1:w888, 2:w889) -> (0:w887:bool)
            n188 = case shown="False" w887 {
              tunnel: w886 -> [w896 w949]
              tunnel: w885 -> [w895 w950]
              tunnel: [w894 w949] -> w884
              tunnel: [w893 w950] -> w883
              frame #0 {
                # "Backlash"
                n189 = flat-sequence {
                  tunnel: [w911] -> w908
                  tunnel: [w913] -> w907
                  tunnel: [w912] -> w906
                  tunnel: w896 -> [w910]
                  tunnel: w895 -> [w909]
                  tunnel: w908 -> [w921]
                  tunnel: [w921] -> w905
                  tunnel: w907 -> [w920]
                  tunnel: w906 -> [w919]
                  tunnel: [w918] -> w904
                  tunnel: [w917] -> w903
                  tunnel: [w916] -> w892
                  tunnel: w905 -> [w931]
                  tunnel: w904 -> [w930]
                  tunnel: w903 -> [w928]
                  tunnel: [w929] -> w902
                  tunnel: [w928] -> w901
                  tunnel: [w927] -> w898
                  tunnel: [w926] -> w897
                  tunnel: w892 -> [w926]
                  tunnel: w902 -> [w942]
                  tunnel: w901 -> [w935]
                  tunnel: [w942] -> w900
                  tunnel: [w941] -> w899
                  tunnel: w898 -> [w941]
                  tunnel: w897 -> [w937]
                  tunnel: [w936] -> w890
                  tunnel: w900 -> [w946]
                  tunnel: w899 -> [w945]
                  tunnel: [w944] -> w894
                  tunnel: [w943] -> w891
                  tunnel: w890 -> [w943]
                  tunnel: [w948] -> w893
                  tunnel: w891 -> [w948]
                  frame #0 {
                    n190 = property on="Y Backlash steps/sec" class="DigNum (strict)"() -> ("Value"=w911:i32)  [unwired: 2 in, 2 out]
                    n191 = Number To Decimal String(number=w911) -> (decimal integer string=w914:string)  [unwired: 1 in]
                    n192 = call "mDrive Send Command.vi"("error in (no error)"=w910, "Extra"=w914, "Command"=T2."Max Velocity", "VISA resource name"=w909) -> ("error out"=w912:errorcluster, "VISA resource name out"=w913:refnum<visa-resource-name>)  [unwired: 3 in, 1 out]
                  }
                  frame #1 {
                    n193 = property on="Y Backlash" class="DigNum (strict)"() -> ("Value"=w916:i32)  [unwired: 2 in, 2 out]
                    n194 = Number To Decimal String(number=w916) -> (decimal integer string=w922:string)  [unwired: 1 in]
                    n195 = call "mDrive Send Command.vi"("error in (no error)"=w919, "Extra"=w922, "Command"=T2."Move to Relative Position", "VISA resource name"=w920) -> ("error out"=w918:errorcluster, "VISA resource name out"=w917:refnum<visa-resource-name>)  [unwired: 3 in, 1 out]
                  }
                  frame #2 {
                    n196 = To Double Precision Float(number=w926) -> (double precision float=w924:dbl)
                    n197 = To Double Precision Float(number=w931) -> (double precision float=w933:dbl)
                    n198 = Absolute Value(x=w924) -> (abs(x)=w925:dbl)
                    n199 = Divide(x=w925, y=w933) -> (x/y=w934:dbl)
                    n200 = Add(x=w934, y=0.3) -> (x+y=w927:dbl)
                    n201 = call "Time Delay8"("error in (no error)"=w930, "Delay Time (s)"=w927) -> ("error out"=w929:errorcluster)  [unwired: 9 in]
                  }
                  frame #3 {
                    n202 = Negate(x=w937) -> (-x=w938:i32)
                    n203 = Number To Decimal String(number=w938) -> (decimal integer string=w939:string)  [unwired: 1 in]
                    n204 = call "mDrive Send Command.vi"("Extra"=w939, "Command"=T2."Move to Relative Position", "VISA resource name"=w935) -> ("VISA resource name out"=w936:refnum<visa-resource-name>)  [unwired: 4 in, 2 out]
                  }
                  frame #4 {
                    n205 = call "Time Delay2"("error in (no error)"=w946, "Delay Time (s)"=w945) -> ("error out"=w944:errorcluster)  [unwired: 9 in]
                  }
                  frame #5 {
                    n206 = property on="Y Backlash corr" class="Bool (strict)"("Val(Sgnl)"=FALSE ("Value (Signaling)")) -> ()  [unwired: 2 in, 2 out]
                  }
                }
              }
              frame #1 {
              }
            }
          }
        }
        n207 = flat-sequence {
          tunnel: [w605] -> w412
          tunnel: [w581] -> w411
          tunnel: [w594] -> w410
          tunnel: [w572] -> w409
          tunnel: w387 -> [w571]
          tunnel: w390 -> [w570]
          tunnel: w412 -> [w611]
          tunnel: [w611] -> w408
          tunnel: w411 -> [w610]
          tunnel: [w610] -> w407
          tunnel: w410 -> [w609]
          tunnel: [w609] -> w406
          tunnel: w409 -> [w606]
          tunnel: [w606] -> w405
          tunnel: w408 -> [w618]
          tunnel: [w619] -> w404
          tunnel: w407 -> [w621]
          tunnel: [w620] -> w403
          tunnel: w406 -> [w617]
          tunnel: [w616] -> w402
          tunnel: w405 -> [w616]
          tunnel: w404 -> [w631]
          tunnel: w403 -> [w632]
          tunnel: w402 -> [w634]
          tunnel: [w630] -> w388
          tunnel: [w629] -> w389
          frame #0 {
            w576 = 0.05 ("Delay Time (s)")
            n208 = property on="Z Step SP" class="DigNum (strict)"() -> ("Maximum"=w596:dbl)  [unwired: 2 in, 2 out]
            n209 = property on="Z Step SP" class="DigNum (strict)"() -> ("Minimum"=w598:dbl)  [unwired: 2 in, 2 out]
            n210 = property on="Z steps/rev" class="DigNum (strict)"() -> ("Value"=w592:u32)  [unwired: 2 in, 2 out]
            n211 = property on="Z offset mm" class="DigNum (strict)"() -> ("Value"=w588:dbl)  [unwired: 2 in, 2 out]
            n212 = To Long Integer(number=w596) -> (32bit integer=w595:i32)
            n213 = To Long Integer(number=w598) -> (32bit integer=w597:i32)
            n214 = To Double Precision Float(number=w592) -> (double precision float=w593:dbl)
            n215 = call "mDrive Send Command.vi"("error in (no error)"=w570, "Extra"="P", "Command"=T2."Print Parameter", "VISA resource name"=w571) -> ("error out"=w600:errorcluster, "read buffer"=w604:string, "VISA resource name out"=w602:refnum<visa-resource-name>)  [unwired: 3 in]
            n216 = call "Time Delay17"("error in (no error)"=w600, "Delay Time (s)"=w576) -> ("error out"=w599:errorcluster)  [unwired: 9 in]
            n217 = Decimal String To Number(string=w604, offset=0) -> (number=w584:i32)  [unwired: 1 in, 1 out]
            n218 = To Long Integer(number=w584) -> (32bit integer=w586:i32)
            n219 = property on="Z Step PV" class="DigNum (strict)"("Val(Sgnl)"=w586) -> ()  [unwired: 2 in, 2 out]
            n220 = call "mDrive Send Command.vi"("error in (no error)"=w599, "Extra"="MV", "Command"=T2."Print Parameter", "VISA resource name"=w602) -> ("error out"=w601:errorcluster, "read buffer"=w582:string, "VISA resource name out"=w605:refnum<visa-resource-name>)  [unwired: 3 in]
            n221 = call "Time Delay16"("error in (no error)"=w601, "Delay Time (s)"=w576) -> ("error out"=w581:errorcluster)  [unwired: 9 in]
            n222 = In Range and Coerce(upper limit=w595, x=w586, lower limit=w597) -> (In Range?=w594:bool)  [unwired: 1 out]
            n223 = To Double Precision Float(number=w586) -> (double precision float=w587:dbl)
            n224 = Decimal String To Number(string=w582, offset=0 ("offset (0)")) -> (number=w575:i32)  [unwired: 1 in, 1 out]
            n225 = property on="Z in Range" class="Bool (strict)"("Val(Sgnl)"=w594) -> ()  [unwired: 2 in, 2 out]
            n226 = Divide(x=w587, y=w593) -> (x/y=w591:dbl)
            n227 = Number To Boolean Array(number=w575) -> (Boolean array=w574:bool[])
            n228 = property on="Z mm/rev" class="DigNum (strict)"() -> ("Value"=w590:dbl)  [unwired: 2 in, 2 out]
            n229 = Index Array(array=w574, index=0) -> (element=w572:bool)
            n230 = property on="Z in Motion" class="Bool (strict)"("Val(Sgnl)"=w572) -> ()  [unwired: 2 in, 2 out]
            n231 = Multiply(x=w591, y=w590) -> (x*y=w589:dbl)
            n232 = Add(x=w589, y=w588) -> (x+y=w585:dbl)
            n233 = property on="Z Position mm PV" class="DigNum (strict)"("Val(Sgnl)"=w585) -> ()  [unwired: 2 in, 2 out]
          }
          frame #1 {
            n234 = property on="Z Scan" class="Bool (strict)"() -> ("Value"=w607:bool)  [unwired: 2 in, 2 out]
            n235 = Or(x=w606, y=w607) -> (x .or. y?=w608:bool)
            n236 = case shown="True" w608 {
              frame #0 {
                n237 = property on="Z Go" class="Bool"("DisabledEnum"=T1."Enabled" ("Disabled")) -> ()  [unwired: 2 in, 2 out]
                n238 = property on="Z Scan OK" class="Bool"("DisabledEnum"=T1."Enabled" ("Disabled")) -> ()  [unwired: 2 in, 2 out]
              }
              frame #1 {
                n239 = property on="Z Go" class="Bool"("DisabledEnum"=T1."Disabled and Grayed Out" ("Disabled")) -> ()  [unwired: 2 in, 2 out]
                n240 = property on="Z Scan OK" class="Bool"("DisabledEnum"=T1."Disabled and Grayed Out" ("Disabled")) -> ()  [unwired: 2 in, 2 out]
              }
            }
          }
          frame #2 {
            n241 = case shown="False" w617 {
              tunnel: w618 -> [w624 w628]
              tunnel: [w625 w628] -> w619
              tunnel: [w626 w627] -> w620
              tunnel: w621 -> [w623 w627]
              frame #0 {
                n242 = call "mDrive Send Command.vi"("error in (no error)"=w623, "Command"=T2."Stop", "VISA resource name"=w624) -> ("error out"=w626:errorcluster, "VISA resource name out"=w625:refnum<visa-resource-name>)  [unwired: 4 in, 1 out]
              }
              frame #1 {
              }
            }
          }
          frame #3 {
            n243 = property on="Z Backlash corr" class="Bool (strict)"() -> ("Value"=w635:bool)  [unwired: 2 in, 2 out]
            n244 = Implies(1:w634, 2:w635) -> (0:w633:bool)
            n245 = case shown="False" w633 {
              tunnel: w632 -> [w642 w695]
              tunnel: w631 -> [w641 w696]
              tunnel: [w640 w695] -> w630
              tunnel: [w639 w696] -> w629
              frame #0 {
                # "Backlash"
                n246 = flat-sequence {
                  tunnel: [w657] -> w654
                  tunnel: [w659] -> w653
                  tunnel: [w658] -> w652
                  tunnel: w642 -> [w656]
                  tunnel: w641 -> [w655]
                  tunnel: w654 -> [w667]
                  tunnel: [w667] -> w651
                  tunnel: w653 -> [w666]
                  tunnel: w652 -> [w665]
                  tunnel: [w664] -> w650
                  tunnel: [w663] -> w649
                  tunnel: [w662] -> w638
                  tunnel: w651 -> [w677]
                  tunnel: w650 -> [w676]
                  tunnel: w649 -> [w674]
                  tunnel: [w675] -> w648
                  tunnel: [w674] -> w647
                  tunnel: [w673] -> w644
                  tunnel: [w672] -> w643
                  tunnel: w638 -> [w672]
                  tunnel: w648 -> [w688]
                  tunnel: w647 -> [w681]
                  tunnel: [w688] -> w646
                  tunnel: [w687] -> w645
                  tunnel: w644 -> [w687]
                  tunnel: w643 -> [w683]
                  tunnel: [w682] -> w636
                  tunnel: w646 -> [w692]
                  tunnel: w645 -> [w691]
                  tunnel: [w690] -> w640
                  tunnel: [w689] -> w637
                  tunnel: w636 -> [w689]
                  tunnel: [w694] -> w639
                  tunnel: w637 -> [w694]
                  frame #0 {
                    n247 = property on="Z Backlash steps/sec" class="DigNum (strict)"() -> ("Value"=w657:i32)  [unwired: 2 in, 2 out]
                    n248 = Number To Decimal String(number=w657) -> (decimal integer string=w660:string)  [unwired: 1 in]
                    n249 = call "mDrive Send Command.vi"("error in (no error)"=w656, "Extra"=w660, "Command"=T2."Max Velocity", "VISA resource name"=w655) -> ("error out"=w658:errorcluster, "VISA resource name out"=w659:refnum<visa-resource-name>)  [unwired: 3 in, 1 out]
                  }
                  frame #1 {
                    n250 = property on="Z Backlash" class="DigNum (strict)"() -> ("Value"=w662:i32)  [unwired: 2 in, 2 out]
                    n251 = Number To Decimal String(number=w662) -> (decimal integer string=w668:string)  [unwired: 1 in]
                    n252 = call "mDrive Send Command.vi"("error in (no error)"=w665, "Extra"=w668, "Command"=T2."Move to Relative Position", "VISA resource name"=w666) -> ("error out"=w664:errorcluster, "VISA resource name out"=w663:refnum<visa-resource-name>)  [unwired: 3 in, 1 out]
                  }
                  frame #2 {
                    n253 = To Double Precision Float(number=w672) -> (double precision float=w670:dbl)
                    n254 = To Double Precision Float(number=w677) -> (double precision float=w679:dbl)
                    n255 = Absolute Value(x=w670) -> (abs(x)=w671:dbl)
                    n256 = Divide(x=w671, y=w679) -> (x/y=w680:dbl)
                    n257 = Add(x=w680, y=0.3) -> (x+y=w673:dbl)
                    n258 = call "Time Delay18"("error in (no error)"=w676, "Delay Time (s)"=w673) -> ("error out"=w675:errorcluster)  [unwired: 9 in]
                  }
                  frame #3 {
                    n259 = Negate(x=w683) -> (-x=w684:i32)
                    n260 = Number To Decimal String(number=w684) -> (decimal integer string=w685:string)  [unwired: 1 in]
                    n261 = call "mDrive Send Command.vi"("Extra"=w685, "Command"=T2."Move to Relative Position", "VISA resource name"=w681) -> ("VISA resource name out"=w682:refnum<visa-resource-name>)  [unwired: 4 in, 2 out]
                  }
                  frame #4 {
                    n262 = call "Time Delay19"("error in (no error)"=w692, "Delay Time (s)"=w691) -> ("error out"=w690:errorcluster)  [unwired: 9 in]
                  }
                  frame #5 {
                    n263 = property on="Z Backlash corr" class="Bool (strict)"("Val(Sgnl)"=FALSE ("Value (Signaling)")) -> ()  [unwired: 2 in, 2 out]
                  }
                }
              }
              frame #1 {
              }
            }
          }
        }
        n264 = flat-sequence {
          tunnel: [w478] -> w401
          tunnel: [w454] -> w400
          tunnel: [w467] -> w399
          tunnel: [w445] -> w398
          tunnel: w386 -> [w444]
          tunnel: w385 -> [w443]
          tunnel: w401 -> [w484]
          tunnel: [w484] -> w397
          tunnel: w400 -> [w483]
          tunnel: [w483] -> w396
          tunnel: w399 -> [w482]
          tunnel: [w482] -> w395
          tunnel: w398 -> [w479]
          tunnel: [w479] -> w394
          tunnel: w397 -> [w491]
          tunnel: [w492] -> w393
          tunnel: w396 -> [w494]
          tunnel: [w493] -> w392
          tunnel: w395 -> [w490]
          tunnel: [w489] -> w391
          tunnel: w394 -> [w489]
          tunnel: w393 -> [w504]
          tunnel: w392 -> [w505]
          tunnel: w391 -> [w507]
          tunnel: [w503] -> w383
          tunnel: [w502] -> w384
          frame #0 {
            w449 = 0.05 ("Delay Time (s)")
            n265 = property on="R Step SP" class="DigNum (strict)"() -> ("Maximum"=w469:dbl)  [unwired: 2 in, 2 out]
            n266 = property on="R Step SP" class="DigNum (strict)"() -> ("Minimum"=w471:dbl)  [unwired: 2 in, 2 out]
            n267 = property on="R steps/rev" class="DigNum (strict)"() -> ("Value"=w465:u32)  [unwired: 2 in, 2 out]
            n268 = property on="R offset deg" class="DigNum (strict)"() -> ("Value"=w461:dbl)  [unwired: 2 in, 2 out]
            n269 = To Long Integer(number=w469) -> (32bit integer=w468:i32)
            n270 = To Long Integer(number=w471) -> (32bit integer=w470:i32)
            n271 = To Double Precision Float(number=w465) -> (double precision float=w466:dbl)
            n272 = call "mDrive Send Command.vi"("error in (no error)"=w443, "Extra"="P", "Command"=T2."Print Parameter", "VISA resource name"=w444) -> ("error out"=w473:errorcluster, "read buffer"=w477:string, "VISA resource name out"=w475:refnum<visa-resource-name>)  [unwired: 3 in]
            n273 = call "Time Delay21"("error in (no error)"=w473, "Delay Time (s)"=w449) -> ("error out"=w472:errorcluster)  [unwired: 9 in]
            n274 = Decimal String To Number(string=w477, offset=0) -> (number=w457:i32)  [unwired: 1 in, 1 out]
            n275 = To Long Integer(number=w457) -> (32bit integer=w459:i32)
            n276 = property on="R Step PV" class="DigNum (strict)"("Val(Sgnl)"=w459) -> ()  [unwired: 2 in, 2 out]
            n277 = call "mDrive Send Command.vi"("error in (no error)"=w472, "Extra"="MV", "Command"=T2."Print Parameter", "VISA resource name"=w475) -> ("error out"=w474:errorcluster, "read buffer"=w455:string, "VISA resource name out"=w478:refnum<visa-resource-name>)  [unwired: 3 in]
            n278 = call "Time Delay20"("error in (no error)"=w474, "Delay Time (s)"=w449) -> ("error out"=w454:errorcluster)  [unwired: 9 in]
            n279 = In Range and Coerce(upper limit=w468, x=w459, lower limit=w470) -> (In Range?=w467:bool)  [unwired: 1 out]
            n280 = To Double Precision Float(number=w459) -> (double precision float=w460:dbl)
            n281 = Decimal String To Number(string=w455, offset=0 ("offset (0)")) -> (number=w448:i32)  [unwired: 1 in, 1 out]
            n282 = property on="R in Range" class="Bool (strict)"("Val(Sgnl)"=w467) -> ()  [unwired: 2 in, 2 out]
            n283 = Divide(x=w460, y=w466) -> (x/y=w464:dbl)
            n284 = Number To Boolean Array(number=w448) -> (Boolean array=w447:bool[])
            n285 = property on="R deg/rev" class="DigNum (strict)"() -> ("Value"=w463:dbl)  [unwired: 2 in, 2 out]
            n286 = Index Array(array=w447, index=0) -> (element=w445:bool)
            n287 = property on="R in Motion" class="Bool (strict)"("Val(Sgnl)"=w445) -> ()  [unwired: 2 in, 2 out]
            n288 = Multiply(x=w464, y=w463) -> (x*y=w462:dbl)
            n289 = Add(x=w462, y=w461) -> (x+y=w458:dbl)
            n290 = property on="R Position deg PV" class="DigNum (strict)"("Val(Sgnl)"=w458) -> ()  [unwired: 2 in, 2 out]
          }
          frame #1 {
            n291 = property on="R Scan" class="Bool (strict)"() -> ("Value"=w480:bool)  [unwired: 2 in, 2 out]
            n292 = Or(x=w479, y=w480) -> (x .or. y?=w481:bool)
            n293 = case shown="True" w481 {
              frame #0 {
                n294 = property on="R Go" class="Bool"("DisabledEnum"=T1."Enabled" ("Disabled")) -> ()  [unwired: 2 in, 2 out]
                n295 = property on="R Scan OK" class="Bool"("DisabledEnum"=T1."Enabled" ("Disabled")) -> ()  [unwired: 2 in, 2 out]
              }
              frame #1 {
                n296 = property on="R Go" class="Bool"("DisabledEnum"=T1."Disabled and Grayed Out" ("Disabled")) -> ()  [unwired: 2 in, 2 out]
                n297 = property on="R Scan OK" class="Bool"("DisabledEnum"=T1."Disabled and Grayed Out" ("Disabled")) -> ()  [unwired: 2 in, 2 out]
              }
            }
          }
          frame #2 {
            n298 = case shown="False" w490 {
              tunnel: w491 -> [w497 w501]
              tunnel: [w498 w501] -> w492
              tunnel: [w499 w500] -> w493
              tunnel: w494 -> [w496 w500]
              frame #0 {
                n299 = call "mDrive Send Command.vi"("error in (no error)"=w496, "Command"=T2."Stop", "VISA resource name"=w497) -> ("error out"=w499:errorcluster, "VISA resource name out"=w498:refnum<visa-resource-name>)  [unwired: 4 in, 1 out]
              }
              frame #1 {
              }
            }
          }
          frame #3 {
            n300 = property on="R Backlash corr" class="Bool (strict)"() -> ("Value"=w508:bool)  [unwired: 2 in, 2 out]
            n301 = Implies(1:w507, 2:w508) -> (0:w506:bool)
            n302 = case shown="False" w506 {
              tunnel: w505 -> [w515 w568]
              tunnel: w504 -> [w514 w569]
              tunnel: [w513 w568] -> w503
              tunnel: [w512 w569] -> w502
              frame #0 {
                # "Backlash"
                n303 = flat-sequence {
                  tunnel: [w530] -> w527
                  tunnel: [w532] -> w526
                  tunnel: [w531] -> w525
                  tunnel: w515 -> [w529]
                  tunnel: w514 -> [w528]
                  tunnel: w527 -> [w540]
                  tunnel: [w540] -> w524
                  tunnel: w526 -> [w539]
                  tunnel: w525 -> [w538]
                  tunnel: [w537] -> w523
                  tunnel: [w536] -> w522
                  tunnel: [w535] -> w511
                  tunnel: w524 -> [w550]
                  tunnel: w523 -> [w549]
                  tunnel: w522 -> [w547]
                  tunnel: [w548] -> w521
                  tunnel: [w547] -> w520
                  tunnel: [w546] -> w517
                  tunnel: [w545] -> w516
                  tunnel: w511 -> [w545]
                  tunnel: w521 -> [w561]
                  tunnel: w520 -> [w554]
                  tunnel: [w561] -> w519
                  tunnel: [w560] -> w518
                  tunnel: w517 -> [w560]
                  tunnel: w516 -> [w556]
                  tunnel: [w555] -> w509
                  tunnel: w519 -> [w565]
                  tunnel: w518 -> [w564]
                  tunnel: [w563] -> w513
                  tunnel: [w562] -> w510
                  tunnel: w509 -> [w562]
                  tunnel: [w567] -> w512
                  tunnel: w510 -> [w567]
                  frame #0 {
                    n304 = property on="R Backlash steps/sec" class="DigNum (strict)"() -> ("Value"=w530:i32)  [unwired: 2 in, 2 out]
                    n305 = Number To Decimal String(number=w530) -> (decimal integer string=w533:string)  [unwired: 1 in]
                    n306 = call "mDrive Send Command.vi"("error in (no error)"=w529, "Extra"=w533, "Command"=T2."Max Velocity", "VISA resource name"=w528) -> ("error out"=w531:errorcluster, "VISA resource name out"=w532:refnum<visa-resource-name>)  [unwired: 3 in, 1 out]
                  }
                  frame #1 {
                    n307 = property on="R Backlash" class="DigNum (strict)"() -> ("Value"=w535:i32)  [unwired: 2 in, 2 out]
                    n308 = Number To Decimal String(number=w535) -> (decimal integer string=w541:string)  [unwired: 1 in]
                    n309 = call "mDrive Send Command.vi"("error in (no error)"=w538, "Extra"=w541, "Command"=T2."Move to Relative Position", "VISA resource name"=w539) -> ("error out"=w537:errorcluster, "VISA resource name out"=w536:refnum<visa-resource-name>)  [unwired: 3 in, 1 out]
                  }
                  frame #2 {
                    n310 = To Double Precision Float(number=w545) -> (double precision float=w543:dbl)
                    n311 = To Double Precision Float(number=w550) -> (double precision float=w552:dbl)
                    n312 = Absolute Value(x=w543) -> (abs(x)=w544:dbl)
                    n313 = Divide(x=w544, y=w552) -> (x/y=w553:dbl)
                    n314 = Add(x=w553, y=0.3) -> (x+y=w546:dbl)
                    n315 = call "Time Delay22"("error in (no error)"=w549, "Delay Time (s)"=w546) -> ("error out"=w548:errorcluster)  [unwired: 9 in]
                  }
                  frame #3 {
                    n316 = Negate(x=w556) -> (-x=w557:i32)
                    n317 = Number To Decimal String(number=w557) -> (decimal integer string=w558:string)  [unwired: 1 in]
                    n318 = call "mDrive Send Command.vi"("Extra"=w558, "Command"=T2."Move to Relative Position", "VISA resource name"=w554) -> ("VISA resource name out"=w555:refnum<visa-resource-name>)  [unwired: 4 in, 2 out]
                  }
                  frame #4 {
                    n319 = call "Time Delay23"("error in (no error)"=w565, "Delay Time (s)"=w564) -> ("error out"=w563:errorcluster)  [unwired: 9 in]
                  }
                  frame #5 {
                    n320 = property on="R Backlash corr" class="Bool (strict)"("Val(Sgnl)"=FALSE ("Value (Signaling)")) -> ()  [unwired: 2 in, 2 out]
                  }
                }
              }
              frame #1 {
              }
            }
          }
        }
        n321 = flat-sequence {
          tunnel: [w732] -> w427
          tunnel: [w708] -> w426
          tunnel: [w721] -> w425
          tunnel: [w699] -> w424
          tunnel: w416 -> [w698]
          tunnel: w415 -> [w697]
          tunnel: w427 -> [w738]
          tunnel: [w738] -> w423
          tunnel: w426 -> [w737]
          tunnel: [w737] -> w422
          tunnel: w425 -> [w736]
          tunnel: [w736] -> w421
          tunnel: w424 -> [w733]
          tunnel: [w733] -> w420
          tunnel: w423 -> [w745]
          tunnel: [w746] -> w419
          tunnel: w422 -> [w748]
          tunnel: [w747] -> w418
          tunnel: w421 -> [w744]
          tunnel: [w743] -> w417
          tunnel: w420 -> [w743]
          tunnel: w419 -> [w758]
          tunnel: w418 -> [w759]
          tunnel: w417 -> [w761]
          tunnel: [w757] -> w413
          tunnel: [w756] -> w414
          frame #0 {
            w703 = 0.05 ("Delay Time (s)")
            n322 = property on="X Step SP" class="DigNum (strict)"() -> ("Maximum"=w723:dbl)  [unwired: 2 in, 2 out]
            n323 = property on="X Step SP" class="DigNum (strict)"() -> ("Minimum"=w725:dbl)  [unwired: 2 in, 2 out]
            n324 = property on="X steps/rev" class="DigNum (strict)"() -> ("Value"=w719:u32)  [unwired: 2 in, 2 out]
            n325 = property on="X offset mm" class="DigNum (strict)"() -> ("Value"=w715:dbl)  [unwired: 2 in, 2 out]
            n326 = To Long Integer(number=w723) -> (32bit integer=w722:i32)
            n327 = To Long Integer(number=w725) -> (32bit integer=w724:i32)
            n328 = To Double Precision Float(number=w719) -> (double precision float=w720:dbl)
            n329 = call "mDrive Send Command.vi"("error in (no error)"=w697, "Extra"="P", "Command"=T2."Print Parameter", "VISA resource name"=w698) -> ("error out"=w727:errorcluster, "read buffer"=w731:string, "VISA resource name out"=w729:refnum<visa-resource-name>)  [unwired: 3 in]
            n330 = call "Time Delay12"("error in (no error)"=w727, "Delay Time (s)"=w703) -> ("error out"=w726:errorcluster)  [unwired: 9 in]
            n331 = Decimal String To Number(string=w731, offset=0) -> (number=w711:i32)  [unwired: 1 in, 1 out]
            n332 = To Long Integer(number=w711) -> (32bit integer=w713:i32)
            n333 = property on="X Step PV" class="DigNum (strict)"("Val(Sgnl)"=w713) -> ()  [unwired: 2 in, 2 out]
            n334 = call "mDrive Send Command.vi"("error in (no error)"=w726, "Extra"="MV", "Command"=T2."Print Parameter", "VISA resource name"=w729) -> ("error out"=w728:errorcluster, "read buffer"=w709:string, "VISA resource name out"=w732:refnum<visa-resource-name>)  [unwired: 3 in]
            n335 = call "Time Delay11"("error in (no error)"=w728, "Delay Time (s)"=w703) -> ("error out"=w708:errorcluster)  [unwired: 9 in]
            n336 = In Range and Coerce(upper limit=w722, x=w713, lower limit=w724) -> (In Range?=w721:bool)  [unwired: 1 out]
            n337 = To Double Precision Float(number=w713) -> (double precision float=w714:dbl)
            n338 = Decimal String To Number(string=w709, offset=0 ("offset (0)")) -> (number=w702:i32)  [unwired: 1 in, 1 out]
            n339 = property on="X  in Range" class="Bool (strict)"("Val(Sgnl)"=w721) -> ()  [unwired: 2 in, 2 out]
            n340 = Divide(x=w714, y=w720) -> (x/y=w718:dbl)
            n341 = Number To Boolean Array(number=w702) -> (Boolean array=w701:bool[])
            n342 = property on="X mm/rev" class="DigNum (strict)"() -> ("Value"=w717:dbl)  [unwired: 2 in, 2 out]
            n343 = Index Array(array=w701, index=0) -> (element=w699:bool)
            n344 = property on="X  in Motion" class="Bool (strict)"("Val(Sgnl)"=w699) -> ()  [unwired: 2 in, 2 out]
            n345 = Multiply(x=w718, y=w717) -> (x*y=w716:dbl)
            n346 = Add(x=w716, y=w715) -> (x+y=w712:dbl)
            n347 = property on="X Position mm PV" class="DigNum (strict)"("Val(Sgnl)"=w712) -> ()  [unwired: 2 in, 2 out]
          }
          frame #1 {
            n348 = property on="X Scan" class="Bool (strict)"() -> ("Value"=w734:bool)  [unwired: 2 in, 2 out]
            n349 = Or(x=w733, y=w734) -> (x .or. y?=w735:bool)
            n350 = case shown="True" w735 {
              frame #0 {
                n351 = property on="X Go" class="Bool"("DisabledEnum"=T1."Enabled" ("Disabled")) -> ()  [unwired: 2 in, 2 out]
                n352 = property on="X Scan OK" class="Bool"("DisabledEnum"=T1."Enabled" ("Disabled")) -> ()  [unwired: 2 in, 2 out]
              }
              frame #1 {
                n353 = property on="X Go" class="Bool"("DisabledEnum"=T1."Disabled and Grayed Out" ("Disabled")) -> ()  [unwired: 2 in, 2 out]
                n354 = property on="X Scan OK" class="Bool"("DisabledEnum"=T1."Disabled and Grayed Out" ("Disabled")) -> ()  [unwired: 2 in, 2 out]
              }
            }
          }
          frame #2 {
            n355 = case shown="False" w744 {
              tunnel: w745 -> [w751 w755]
              tunnel: [w752 w755] -> w746
              tunnel: [w753 w754] -> w747
              tunnel: w748 -> [w750 w754]
              frame #0 {
                n356 = call "mDrive Send Command.vi"("error in (no error)"=w750, "Command"=T2."Stop", "VISA resource name"=w751) -> ("error out"=w753:errorcluster, "VISA resource name out"=w752:refnum<visa-resource-name>)  [unwired: 4 in, 1 out]
              }
              frame #1 {
              }
            }
          }
          frame #3 {
            n357 = property on="X Backlash corr" class="Bool (strict)"() -> ("Value"=w762:bool)  [unwired: 2 in, 2 out]
            n358 = Implies(1:w761, 2:w762) -> (0:w760:bool)
            n359 = case shown="False" w760 {
              tunnel: w759 -> [w769 w822]
              tunnel: w758 -> [w768 w823]
              tunnel: [w767 w822] -> w757
              tunnel: [w766 w823] -> w756
              frame #0 {
                # "Backlash"
                n360 = flat-sequence {
                  tunnel: [w784] -> w781
                  tunnel: [w786] -> w780
                  tunnel: [w785] -> w779
                  tunnel: w769 -> [w783]
                  tunnel: w768 -> [w782]
                  tunnel: w781 -> [w794]
                  tunnel: [w794] -> w778
                  tunnel: w780 -> [w793]
                  tunnel: w779 -> [w792]
                  tunnel: [w791] -> w777
                  tunnel: [w790] -> w776
                  tunnel: [w789] -> w765
                  tunnel: w778 -> [w804]
                  tunnel: w777 -> [w803]
                  tunnel: w776 -> [w801]
                  tunnel: [w802] -> w775
                  tunnel: [w801] -> w774
                  tunnel: [w800] -> w771
                  tunnel: [w799] -> w770
                  tunnel: w765 -> [w799]
                  tunnel: w775 -> [w815]
                  tunnel: w774 -> [w808]
                  tunnel: [w815] -> w773
                  tunnel: [w814] -> w772
                  tunnel: w771 -> [w814]
                  tunnel: w770 -> [w810]
                  tunnel: [w809] -> w763
                  tunnel: w773 -> [w819]
                  tunnel: w772 -> [w818]
                  tunnel: [w817] -> w767
                  tunnel: [w816] -> w764
                  tunnel: w763 -> [w816]
                  tunnel: [w821] -> w766
                  tunnel: w764 -> [w821]
                  frame #0 {
                    n361 = property on="X Backlash steps/sec" class="DigNum (strict)"() -> ("Value"=w784:i32)  [unwired: 2 in, 2 out]
                    n362 = Number To Decimal String(number=w784) -> (decimal integer string=w787:string)  [unwired: 1 in]
                    n363 = call "mDrive Send Command.vi"("error in (no error)"=w783, "Extra"=w787, "Command"=T2."Max Velocity", "VISA resource name"=w782) -> ("error out"=w785:errorcluster, "VISA resource name out"=w786:refnum<visa-resource-name>)  [unwired: 3 in, 1 out]
                  }
                  frame #1 {
                    n364 = property on="X Backlash" class="DigNum (strict)"() -> ("Value"=w789:i32)  [unwired: 2 in, 2 out]
                    n365 = Number To Decimal String(number=w789) -> (decimal integer string=w795:string)  [unwired: 1 in]
                    n366 = call "mDrive Send Command.vi"("error in (no error)"=w792, "Extra"=w795, "Command"=T2."Move to Relative Position", "VISA resource name"=w793) -> ("error out"=w791:errorcluster, "VISA resource name out"=w790:refnum<visa-resource-name>)  [unwired: 3 in, 1 out]
                  }
                  frame #2 {
                    n367 = To Double Precision Float(number=w799) -> (double precision float=w797:dbl)
                    n368 = To Double Precision Float(number=w804) -> (double precision float=w806:dbl)
                    n369 = Absolute Value(x=w797) -> (abs(x)=w798:dbl)
                    n370 = Divide(x=w798, y=w806) -> (x/y=w807:dbl)
                    n371 = Add(x=w807, y=0.3) -> (x+y=w800:dbl)
                    n372 = call "Time Delay13"("error in (no error)"=w803, "Delay Time (s)"=w800) -> ("error out"=w802:errorcluster)  [unwired: 9 in]
                  }
                  frame #3 {
                    n373 = Negate(x=w810) -> (-x=w811:i32)
                    n374 = Number To Decimal String(number=w811) -> (decimal integer string=w812:string)  [unwired: 1 in]
                    n375 = call "mDrive Send Command.vi"("Extra"=w812, "Command"=T2."Move to Relative Position", "VISA resource name"=w808) -> ("VISA resource name out"=w809:refnum<visa-resource-name>)  [unwired: 4 in, 2 out]
                  }
                  frame #4 {
                    n376 = call "Time Delay14"("error in (no error)"=w819, "Delay Time (s)"=w818) -> ("error out"=w817:errorcluster)  [unwired: 9 in]
                  }
                  frame #5 {
                    n377 = property on="X Backlash corr" class="Bool (strict)"("Val(Sgnl)"=FALSE ("Value (Signaling)")) -> ()  [unwired: 2 in, 2 out]
                  }
                }
              }
              frame #1 {
              }
            }
          }
        }
        n378 = property on="X Position mm PV" class="DigNum (strict)"() -> ("Value"=w378:dbl)  [unwired: 2 in, 2 out]
        n379 = property on="Y Position mm PV" class="DigNum (strict)"() -> ("Value"=w380:dbl)  [unwired: 2 in, 2 out]
        n380 = property on="Z Position mm PV" class="DigNum (strict)"() -> ("Value"=w377:dbl)  [unwired: 2 in, 2 out]
        n381 = property on="R Position deg PV" class="DigNum (strict)"() -> ("Value"=w379:dbl)  [unwired: 2 in, 2 out]
        n382 = call "Build XY Graph"("Y Input"=w380, "X Input"=w378) -> ("XY Graph"=→"XY Graph":cluster{"Y":dbl[], "Y":dbl[]}[])  [unwired: 8 in, 1 out]
        n383 = call "Build XY Graph2"("Y Input"=w379, "X Input"=w377) -> ("XY Graph"=→"XY Graph 2":cluster{"Y":dbl[], "Y":dbl[]}[])  [unwired: 8 in, 1 out]
      }
      event #1 {
        n384 = event-data() -> ()  [unwired: 1 in, 5 out]
        n385 = property on="Z steps/rev" class="DigNum (strict)"() -> ("Value"=w962:u32)  [unwired: 2 in, 2 out]
        n386 = property on="X steps/rev" class="DigNum (strict)"() -> ("Value"=w971:u32)  [unwired: 2 in, 2 out]
        n387 = property on="Y steps/rev" class="DigNum (strict)"() -> ("Value"=w980:u32)  [unwired: 2 in, 2 out]
        n388 = property on="R steps/rev" class="DigNum (strict)"() -> ("Value"=w953:u32)  [unwired: 2 in, 2 out]
        n389 = property on="R offset deg" class="DigNum (strict)"() -> ("Value"=w951:dbl)  [unwired: 2 in, 2 out]
        n390 = property on="Z offset mm" class="DigNum (strict)"() -> ("Value"=w960:dbl)  [unwired: 2 in, 2 out]
        n391 = property on="X offset mm" class="DigNum (strict)"() -> ("Value"=w969:dbl)  [unwired: 2 in, 2 out]
        n392 = property on="Y offset mm" class="DigNum (strict)"() -> ("Value"=w978:dbl)  [unwired: 2 in, 2 out]
        n393 = To Double Precision Float(number=w980) -> (double precision float=w983:dbl)
        n394 = property on="Reset Z Position mm" class="DigNum (strict)"() -> ("Value"=w968:dbl)  [unwired: 2 in, 2 out]
        n395 = property on="Reset X Position mm" class="DigNum (strict)"() -> ("Value"=w977:dbl)  [unwired: 2 in, 2 out]
        n396 = property on="Reset Y Position mm" class="DigNum (strict)"() -> ("Value"=w986:dbl)  [unwired: 2 in, 2 out]
        n397 = property on="Reset R Position deg" class="DigNum (strict)"() -> ("Value"=w959:dbl)  [unwired: 2 in, 2 out]
        n398 = Subtract(x=w968, y=w960) -> (x-y=w967:dbl)
        n399 = Subtract(x=w959, y=w951) -> (x-y=w958:dbl)
        n400 = Subtract(x=w977, y=w969) -> (x-y=w976:dbl)
        n401 = Subtract(x=w986, y=w978) -> (x-y=w985:dbl)
        n402 = property on="Z mm/rev" class="DigNum (strict)"() -> ("Value"=w961:dbl)  [unwired: 2 in, 2 out]
        n403 = property on="X mm/rev" class="DigNum (strict)"() -> ("Value"=w970:dbl)  [unwired: 2 in, 2 out]
        n404 = property on="Y mm/rev" class="DigNum (strict)"() -> ("Value"=w979:dbl)  [unwired: 2 in, 2 out]
        n405 = property on="R deg/rev" class="DigNum (strict)"() -> ("Value"=w952:dbl)  [unwired: 2 in, 2 out]
        n406 = Divide(x=w985, y=w979) -> (x/y=w984:dbl)
        n407 = Divide(x=w967, y=w961) -> (x/y=w966:dbl)
        n408 = Divide(x=w958, y=w952) -> (x/y=w957:dbl)
        n409 = Divide(x=w976, y=w970) -> (x/y=w975:dbl)
        n410 = To Double Precision Float(number=w962) -> (double precision float=w965:dbl)
        n411 = To Double Precision Float(number=w953) -> (double precision float=w956:dbl)
        n412 = To Double Precision Float(number=w971) -> (double precision float=w974:dbl)
        n413 = Multiply(x=w966, y=w965) -> (x*y=w964:dbl)
        n414 = Multiply(x=w957, y=w956) -> (x*y=w955:dbl)
        n415 = Multiply(x=w975, y=w974) -> (x*y=w973:dbl)
        n416 = Multiply(x=w984, y=w983) -> (x*y=w982:dbl)
        n417 = To Long Integer(number=w964) -> (32bit integer=w963:i32)
        n418 = To Long Integer(number=w955) -> (32bit integer=w954:i32)
        n419 = To Long Integer(number=w973) -> (32bit integer=w972:i32)
        n420 = To Long Integer(number=w982) -> (32bit integer=w981:i32)
        n421 = property on="Reset Z Motor Steps" class="DigNum (strict)"("Val(Sgnl)"=w963) -> ()  [unwired: 2 in, 2 out]
        n422 = property on="Reset R Motor Steps" class="DigNum (strict)"("Val(Sgnl)"=w954) -> ()  [unwired: 2 in, 2 out]
        n423 = property on="Reset X Motor Steps" class="DigNum (strict)"("Val(Sgnl)"=w972) -> ()  [unwired: 2 in, 2 out]
        n424 = property on="Reset Y Motor Steps" class="DigNum (strict)"("Val(Sgnl)"=w981) -> ()  [unwired: 2 in, 2 out]
      }
      event #2 {
        n425 = event-data() -> ()  [unwired: 1 in, 5 out]
        n426 = property on="Z Step SP" class="DigNum (strict)"() -> ("Value"=w1002:i32)  [unwired: 2 in, 2 out]
        n427 = property on="Y Step SP" class="DigNum (strict)"() -> ("Value"=w1018:i32)  [unwired: 2 in, 2 out]
        n428 = property on="R Step SP" class="DigNum (strict)"() -> ("Value"=w994:i32)  [unwired: 2 in, 2 out]
        n429 = property on="X steps/rev" class="DigNum (strict)"() -> ("Value"=w1008:u32)  [unwired: 2 in, 2 out]
        n430 = property on="X steps/rev" class="DigNum (strict)"() -> ("Value"=w1035:u32)  [unwired: 2 in, 2 out]
        n431 = property on="X mm/rev" class="DigNum (strict)"() -> ("Value"=w988:dbl)  [unwired: 2 in, 2 out]
        n432 = property on="Z steps/rev" class="DigNum (strict)"() -> ("Value"=w1000:u32)  [unwired: 2 in, 2 out]
        n433 = property on="Z steps/rev" class="DigNum (strict)"() -> ("Value"=w1029:u32)  [unwired: 2 in, 2 out]
        n434 = property on="Z mm/rev" class="DigNum (strict)"() -> ("Value"=w989:dbl)  [unwired: 2 in, 2 out]
        n435 = property on="Y steps/rev" class="DigNum (strict)"() -> ("Value"=w1016:u32)  [unwired: 2 in, 2 out]
        n436 = property on="Y steps/rev" class="DigNum (strict)"() -> ("Value"=w1041:u32)  [unwired: 2 in, 2 out]
        n437 = property on="Y mm/rev" class="DigNum (strict)"() -> ("Value"=w987:dbl)  [unwired: 2 in, 2 out]
        n438 = property on="R steps/rev" class="DigNum (strict)"() -> ("Value"=w992:u32)  [unwired: 2 in, 2 out]
        n439 = property on="R steps/rev" class="DigNum (strict)"() -> ("Value"=w1023:u32)  [unwired: 2 in, 2 out]
        n440 = property on="R deg/rev" class="DigNum (strict)"() -> ("Value"=w990:dbl)  [unwired: 2 in, 2 out]
        n441 = property on="X Step SP" class="DigNum (strict)"() -> ("Value"=w1010:i32)  [unwired: 2 in, 2 out]
        n442 = To Double Precision Float(number=w1002) -> (double precision float=w1003:dbl)
        n443 = To Double Precision Float(number=w1000) -> (double precision float=w1006:dbl)
        n444 = To Double Precision Float(number=w1029) -> (double precision float=w1034:dbl)
        n445 = To Double Precision Float(number=w1018) -> (double precision float=w1019:dbl)
        n446 = To Double Precision Float(number=w1016) -> (double precision float=w1022:dbl)
        n447 = To Double Precision Float(number=w1041) -> (double precision float=w1046:dbl)
        n448 = To Double Precision Float(number=w994) -> (double precision float=w995:dbl)
        n449 = To Double Precision Float(number=w992) -> (double precision float=w998:dbl)
        n450 = To Double Precision Float(number=w1023) -> (double precision float=w1028:dbl)
        n451 = To Double Precision Float(number=w1010) -> (double precision float=w1011:dbl)
        n452 = To Double Precision Float(number=w1008) -> (double precision float=w1014:dbl)
        n453 = To Double Precision Float(number=w1035) -> (double precision float=w1040:dbl)
        n454 = property on="R Velocity SP step/sec" class="DigNum (strict)"() -> ("Value"=w1025:i32)  [unwired: 2 in, 2 out]
        n455 = property on="Z Velocity SP step/sec" class="DigNum (strict)"() -> ("Value"=w1031:i32)  [unwired: 2 in, 2 out]
        n456 = property on="Y Velocity SP step/sec" class="DigNum (strict)"() -> ("Value"=w1043:i32)  [unwired: 2 in, 2 out]
        n457 = property on="X Velocity SP step/sec" class="DigNum (strict)"() -> ("Value"=w1037:i32)  [unwired: 2 in, 2 out]
        n458 = Divide(x=w1003, y=w1006) -> (x/y=w1005:dbl)
        n459 = Divide(x=w1019, y=w1022) -> (x/y=w1021:dbl)
        n460 = Divide(x=w995, y=w998) -> (x/y=w997:dbl)
        n461 = Divide(x=w1011, y=w1014) -> (x/y=w1013:dbl)
        n462 = property on="R offset deg" class="DigNum (strict)"() -> ("Value"=w991:dbl)  [unwired: 2 in, 2 out]
        n463 = property on="Z offset mm" class="DigNum (strict)"() -> ("Value"=w999:dbl)  [unwired: 2 in, 2 out]
        n464 = property on="Y offset mm" class="DigNum (strict)"() -> ("Value"=w1015:dbl)  [unwired: 2 in, 2 out]
        n465 = property on="X offset mm" class="DigNum (strict)"() -> ("Value"=w1007:dbl)  [unwired: 2 in, 2 out]
        n466 = Multiply(x=w1005, y=w989) -> (x*y=w1004:dbl)
        n467 = Multiply(x=w1021, y=w987) -> (x*y=w1020:dbl)
        n468 = Multiply(x=w997, y=w990) -> (x*y=w996:dbl)
        n469 = Multiply(x=w1013, y=w988) -> (x*y=w1012:dbl)
        n470 = To Double Precision Float(number=w1031) -> (double precision float=w1032:dbl)
        n471 = To Double Precision Float(number=w1043) -> (double precision float=w1044:dbl)
        n472 = To Double Precision Float(number=w1025) -> (double precision float=w1026:dbl)
        n473 = To Double Precision Float(number=w1037) -> (double precision float=w1038:dbl)
        n474 = Add(x=w1004, y=w999) -> (x+y=w1001:dbl)
        n475 = Divide(x=w1032, y=w1034) -> (x/y=w1033:dbl)
        n476 = Add(x=w1020, y=w1015) -> (x+y=w1017:dbl)
        n477 = Divide(x=w1044, y=w1046) -> (x/y=w1045:dbl)
        n478 = Add(x=w996, y=w991) -> (x+y=w993:dbl)
        n479 = Divide(x=w1026, y=w1028) -> (x/y=w1027:dbl)
        n480 = Add(x=w1012, y=w1007) -> (x+y=w1009:dbl)
        n481 = Divide(x=w1038, y=w1040) -> (x/y=w1039:dbl)
        n482 = Multiply(x=w1033, y=w989) -> (x*y=w1030:dbl)
        n483 = Multiply(x=w1045, y=w987) -> (x*y=w1042:dbl)
        n484 = Multiply(x=w1027, y=w990) -> (x*y=w1024:dbl)
        n485 = Multiply(x=w1039, y=w988) -> (x*y=w1036:dbl)
        n486 = property on="Z Position MV mm" class="DigNum (strict)"("Val(Sgnl)"=w1001) -> ()  [unwired: 2 in, 2 out]
        n487 = property on="Y Position MV mm" class="DigNum (strict)"("Val(Sgnl)"=w1017) -> ()  [unwired: 2 in, 2 out]
        n488 = property on="R Position MV deg" class="DigNum (strict)"("Val(Sgnl)"=w993) -> ()  [unwired: 2 in, 2 out]
        n489 = property on="X Position MV mm" class="DigNum (strict)"("Val(Sgnl)"=w1009) -> ()  [unwired: 2 in, 2 out]
        n490 = property on="Z Velocity MV mm/sec" class="DigNum (strict)"("Val(Sgnl)"=w1030) -> ()  [unwired: 2 in, 2 out]
        n491 = property on="Y Velocity MV mm/sec" class="DigNum (strict)"("Val(Sgnl)"=w1042) -> ()  [unwired: 2 in, 2 out]
        n492 = property on="R Velocity MVdeg/sec" class="DigNum (strict)"("Val(Sgnl)"=w1024) -> ()  [unwired: 2 in, 2 out]
        n493 = property on="X Velocity MV mm/sec" class="DigNum (strict)"("Val(Sgnl)"=w1036) -> ()  [unwired: 2 in, 2 out]
      }
      event #3 {
        n494 = event-data() -> ()  [unwired: 1 in, 5 out]
        n495 = property on="X Step SP" class="DigNum (strict)"() -> ("Maximum"=w1116:dbl)  [unwired: 2 in, 2 out]
        n496 = property on="X Step SP" class="DigNum (strict)"() -> ("Minimum"=w1117:dbl)  [unwired: 2 in, 2 out]
        n497 = property on="X Step PV" class="DigNum (strict)"() -> ("Value"=w1110:i32)  [unwired: 2 in, 2 out]
        n498 = property on="X steps/rev" class="DigNum (strict)"() -> ("Value"=w1112:u32)  [unwired: 2 in, 2 out]
        n499 = property on="X mm/rev" class="DigNum (strict)"() -> ("Value"=w1111:dbl)  [unwired: 2 in, 2 out]
        n500 = To Double Precision Float(number=w1110) -> (double precision float=w1063:dbl)
        n501 = property on="Y Step SP" class="DigNum (strict)"() -> ("Maximum"=w1102:dbl)  [unwired: 2 in, 2 out]
        n502 = property on="Y Step SP" class="DigNum (strict)"() -> ("Minimum"=w1103:dbl)  [unwired: 2 in, 2 out]
        n503 = property on="Y Step PV" class="DigNum (strict)"() -> ("Value"=w1096:i32)  [unwired: 2 in, 2 out]
        n504 = property on="Y mm/rev" class="DigNum (strict)"() -> ("Value"=w1097:dbl)  [unwired: 2 in, 2 out]
        n505 = property on="Y steps/rev" class="DigNum (strict)"() -> ("Value"=w1098:u32)  [unwired: 2 in, 2 out]
        n506 = Subtract(x=w1117, y=w1063) -> (x-y=w1118:dbl)
        n507 = Subtract(x=w1116, y=w1063) -> (x-y=w1115:dbl)
        n508 = property on="X Scan Length SP steps" class="DigNum (strict)"() -> ("Value"=w1108:i32)  [unwired: 2 in, 2 out]
        n509 = To Double Precision Float(number=w1096) -> (double precision float=w1062:dbl)
        n510 = property on="X Scan Velocity SP steps/sec" class="DigNum (strict)"() -> ("Value"=w1113:i32)  [unwired: 2 in, 2 out]
        n511 = To Double Precision Float(number=w1112) -> (double precision float=w1109:dbl)
        n512 = To Double Precision Float(number=w1108) -> (double precision float=w1048:dbl)
        n513 = property on="X Scan Length SP steps" class="DigNum (strict)"("Minimum"=w1118) -> ()  [unwired: 2 in, 2 out]
        n514 = property on="X Scan Length SP steps" class="DigNum (strict)"("Maximum"=w1115) -> ()  [unwired: 2 in, 2 out]
        n515 = property on="R Step SP" class="DigNum (strict)"() -> ("Minimum"=w1074:dbl)  [unwired: 2 in, 2 out]
        n516 = property on="Z Step SP" class="DigNum (strict)"() -> ("Maximum"=w1089:dbl)  [unwired: 2 in, 2 out]
        n517 = property on="Z Step SP" class="DigNum (strict)"() -> ("Minimum"=w1090:dbl)  [unwired: 2 in, 2 out]
        n518 = Subtract(x=w1102, y=w1062) -> (x-y=w1101:dbl)
        n519 = Subtract(x=w1103, y=w1062) -> (x-y=w1104:dbl)
        n520 = property on="Y Scan Length SP steps" class="DigNum (strict)"() -> ("Value"=w1099:i32)  [unwired: 2 in, 2 out]
        n521 = property on="R Step PV" class="DigNum (strict)"() -> ("Value"=w1069:i32)  [unwired: 2 in, 2 out]
        n522 = property on="R deg/rev" class="DigNum (strict)"() -> ("Value"=w1070:dbl)  [unwired: 2 in, 2 out]
        n523 = property on="R steps/rev" class="DigNum (strict)"() -> ("Value"=w1071:u32)  [unwired: 2 in, 2 out]
        n524 = property on="Z Step PV" class="DigNum (strict)"() -> ("Value"=w1083:i32)  [unwired: 2 in, 2 out]
        n525 = property on="Z mm/rev" class="DigNum (strict)"() -> ("Value"=w1084:dbl)  [unwired: 2 in, 2 out]
        n526 = property on="Z steps/rev" class="DigNum (strict)"() -> ("Value"=w1085:u32)  [unwired: 2 in, 2 out]
        n527 = Divide(x=w1048, y=w1109) -> (x/y=w1107:dbl)
        n528 = To Double Precision Float(number=w1113) -> (double precision float=w1047:dbl)
        n529 = property on="Y Scan Velocity SP steps/sec" class="DigNum (strict)"() -> ("Value"=w1095:i32)  [unwired: 2 in, 2 out]
        n530 = To Double Precision Float(number=w1098) -> (double precision float=w1053:dbl)
        n531 = To Double Precision Float(number=w1099) -> (double precision float=w1052:dbl)
        n532 = property on="Y Scan Length SP steps" class="DigNum (strict)"("Maximum"=w1101) -> ()  [unwired: 2 in, 2 out]
        n533 = property on="Y Scan Length SP steps" class="DigNum (strict)"("Minimum"=w1104) -> ()  [unwired: 2 in, 2 out]
        n534 = To Double Precision Float(number=w1069) -> (double precision float=w1060:dbl)
        n535 = property on="R Step SP" class="DigNum (strict)"() -> ("Maximum"=w1077:dbl)  [unwired: 2 in, 2 out]
        n536 = To Double Precision Float(number=w1083) -> (double precision float=w1061:dbl)
        n537 = Divide(x=w1047, y=w1109) -> (x/y=w1114:dbl)
        n538 = Multiply(x=w1111, y=w1107) -> (x*y=w1105:dbl)
        n539 = Divide(x=w1052, y=w1053) -> (x/y=w1100:dbl)
        n540 = To Double Precision Float(number=w1095) -> (double precision float=w1051:dbl)
        n541 = Subtract(x=w1074, y=w1060) -> (x-y=w1075:dbl)
        n542 = property on="R Scan Length SP steps" class="DigNum (strict)"() -> ("Value"=w1072:i32)  [unwired: 2 in, 2 out]
        n543 = Subtract(x=w1089, y=w1061) -> (x-y=w1088:dbl)
        n544 = Subtract(x=w1090, y=w1061) -> (x-y=w1091:dbl)
        n545 = property on="Z Scan Length SP steps" class="DigNum (strict)"() -> ("Value"=w1086:i32)  [unwired: 2 in, 2 out]
        n546 = Multiply(x=w1114, y=w1111) -> (x*y=w1106:dbl)
        n547 = property on="X Scan length MV mm" class="DigNum (strict)"("Val(Sgnl)"=w1105) -> ()  [unwired: 2 in, 2 out]
        n548 = property on="R Scan Velocity SP steps/sec" class="DigNum (strict)"() -> ("Value"=w1067:i32)  [unwired: 2 in, 2 out]
        n549 = Divide(x=w1051, y=w1053) -> (x/y=w1094:dbl)
        n550 = Multiply(x=w1100, y=w1097) -> (x*y=w1093:dbl)
        n551 = To Double Precision Float(number=w1071) -> (double precision float=w1068:dbl)
        n552 = To Double Precision Float(number=w1072) -> (double precision float=w1057:dbl)
        n553 = property on="R Scan Length SP steps" class="DigNum (strict)"("Minimum"=w1075) -> ()  [unwired: 2 in, 2 out]
        n554 = property on="Z Scan Velocity SP steps/sec" class="DigNum (strict)"() -> ("Value"=w1081:i32)  [unwired: 2 in, 2 out]
        n555 = To Double Precision Float(number=w1085) -> (double precision float=w1082:dbl)
        n556 = To Double Precision Float(number=w1086) -> (double precision float=w1059:dbl)
        n557 = property on="Z Scan Length SP steps" class="DigNum (strict)"("Maximum"=w1088) -> ()  [unwired: 2 in, 2 out]
        n558 = property on="Z Scan Length SP steps" class="DigNum (strict)"("Minimum"=w1091) -> ()  [unwired: 2 in, 2 out]
        n559 = Subtract(x=w1077, y=w1060) -> (x-y=w1076:dbl)
        n560 = property on="X Scan velocity MV mm/sec" class="DigNum (strict)"("Value"=w1106) -> ()  [unwired: 2 in, 2 out]
        n561 = Divide(x=w1057, y=w1068) -> (x/y=w1073:dbl)
        n562 = To Double Precision Float(number=w1067) -> (double precision float=w1056:dbl)
        n563 = Multiply(x=w1097, y=w1094) -> (x*y=w1092:dbl)
        n564 = property on="Y Scan length MV mm" class="DigNum (strict)"("Value"=w1093) -> ()  [unwired: 2 in, 2 out]
        n565 = Divide(x=w1059, y=w1082) -> (x/y=w1087:dbl)
        n566 = To Double Precision Float(number=w1081) -> (double precision float=w1058:dbl)
        n567 = property on="R Scan Length SP steps" class="DigNum (strict)"("Maximum"=w1076) -> ()  [unwired: 2 in, 2 out]
        n568 = property on="Y Scan velocity MV mm/sec" class="DigNum (strict)"("Val(Sgnl)"=w1092) -> ()  [unwired: 2 in, 2 out]
        n569 = Divide(x=w1056, y=w1068) -> (x/y=w1066:dbl)
        n570 = Multiply(x=w1073, y=w1070) -> (x*y=w1065:dbl)
        n571 = Divide(x=w1058, y=w1082) -> (x/y=w1080:dbl)
        n572 = Multiply(x=w1087, y=w1084) -> (x*y=w1079:dbl)
        n573 = Multiply(x=w1070, y=w1066) -> (x*y=w1064:dbl)
        n574 = Divide(x=w1048, y=w1047) -> (x/y=→"X Scan Duration":dbl)
        n575 = property on="R Scan length MV deg" class="DigNum (strict)"("Value"=w1065) -> ()  [unwired: 2 in, 2 out]
        n576 = Multiply(x=w1084, y=w1080) -> (x*y=w1078:dbl)
        n577 = property on="Z Scan length MV mm" class="DigNum (strict)"("Value"=w1079) -> ()  [unwired: 2 in, 2 out]
        n578 = Divide(x=w1052, y=w1051) -> (x/y=→"Y Scan Duration":dbl)
        n579 = property on="R Scan Velocity SP deg/sec" class="DigNum (strict)"("Val(Sgnl)"=w1064) -> ()  [unwired: 2 in, 2 out]
        n580 = property on="Z Scan velocity MV mm/sec" class="DigNum (strict)"("Val(Sgnl)"=w1078) -> ()  [unwired: 2 in, 2 out]
        n581 = Divide(x=w1059, y=w1058) -> (x/y=→"Z Scan Duration":dbl)
        n582 = Divide(x=w1057, y=w1056) -> (x/y=→"R Scan Duration":dbl)
      }
      event #4 {
        n583 = event-data() -> ()  [unwired: 1 in, 7 out]
        n584 = property on="Y steps/rev" class="DigNum (strict)"() -> ("Value"=w1135:u32)  [unwired: 2 in, 2 out]
        n585 = property on="Y offset mm" class="DigNum (strict)"() -> ("Value"=w1133:dbl)  [unwired: 2 in, 2 out]
        n586 = property on="Y Position SP mm" class="DigNum (strict)"() -> ("Value"=w1132:dbl)  [unwired: 2 in, 2 out]
        n587 = property on="Y Velocity SP step/sec" class="DigNum (strict)"() -> ("Maximum"=w1122:dbl)  [unwired: 2 in, 2 out]
        n588 = property on="Y Velocity SP step/sec" class="DigNum (strict)"() -> ("Minimum"=w1121:dbl)  [unwired: 2 in, 2 out]
        n589 = Subtract(x=w1132, y=w1133) -> (x-y=w1136:dbl)
        n590 = property on="Y Velocity SP mm/sec" class="DigNum (strict)"() -> ("Value"=w1126:dbl)  [unwired: 2 in, 2 out]
        n591 = property on="Y mm/rev" class="DigNum (strict)"() -> ("Value"=w1119:dbl)  [unwired: 2 in, 2 out]
        n592 = Divide(x=w1136, y=w1119) -> (x/y=w1137:dbl)
        n593 = Divide(x=w1126, y=w1119) -> (x/y=w1127:dbl)
        n594 = To Double Precision Float(number=w1135) -> (double precision float=w1120:dbl)
        n595 = Multiply(x=w1137, y=w1120) -> (x*y=w1131:dbl)
        n596 = Multiply(x=w1127, y=w1120) -> (x*y=w1124:dbl)
        n597 = property on="Y Step SP" class="DigNum (strict)"() -> ("Maximum"=w1129:dbl)  [unwired: 2 in, 2 out]
        n598 = property on="Y Step SP" class="DigNum (strict)"() -> ("Minimum"=w1128:dbl)  [unwired: 2 in, 2 out]
        n599 = In Range and Coerce(upper limit=w1122, x=w1124, lower limit=w1121) -> (coerced(x)=w1123:dbl)  [unwired: 1 out]
        n600 = To Long Integer(number=w1123) -> (32bit integer=w1125:i32)
        n601 = In Range and Coerce(upper limit=w1129, x=w1131, lower limit=w1128) -> (coerced(x)=w1130:dbl)  [unwired: 1 out]
        n602 = To Long Integer(number=w1130) -> (32bit integer=w1134:i32)
        n603 = property on="Y Velocity SP step/sec" class="DigNum (strict)"("Val(Sgnl)"=w1125) -> ()  [unwired: 2 in, 2 out]
        n604 = property on="Y Step SP" class="DigNum (strict)"("Val(Sgnl)"=w1134) -> ()  [unwired: 2 in, 2 out]
      }
      event #5 {
        n605 = event-data() -> ()  [unwired: 1 in, 7 out]
        n606 = property on="X steps/rev" class="DigNum (strict)"() -> ("Value"=w1154:u32)  [unwired: 2 in, 2 out]
        n607 = property on="X offset mm" class="DigNum (strict)"() -> ("Value"=w1152:dbl)  [unwired: 2 in, 2 out]
        n608 = property on="X Position SP mm" class="DigNum (strict)"() -> ("Value"=w1151:dbl)  [unwired: 2 in, 2 out]
        n609 = property on="X Velocity SP step/sec" class="DigNum (strict)"() -> ("Maximum"=w1141:dbl)  [unwired: 2 in, 2 out]
        n610 = property on="X Velocity SP step/sec" class="DigNum (strict)"() -> ("Minimum"=w1140:dbl)  [unwired: 2 in, 2 out]
        n611 = Subtract(x=w1151, y=w1152) -> (x-y=w1155:dbl)
        n612 = property on="X Velocity SP mm/sec" class="DigNum (strict)"() -> ("Value"=w1145:dbl)  [unwired: 2 in, 2 out]
        n613 = property on="X mm/rev" class="DigNum (strict)"() -> ("Value"=w1138:dbl)  [unwired: 2 in, 2 out]
        n614 = Divide(x=w1155, y=w1138) -> (x/y=w1156:dbl)
        n615 = Divide(x=w1145, y=w1138) -> (x/y=w1146:dbl)
        n616 = To Double Precision Float(number=w1154) -> (double precision float=w1139:dbl)
        n617 = Multiply(x=w1156, y=w1139) -> (x*y=w1150:dbl)
        n618 = Multiply(x=w1146, y=w1139) -> (x*y=w1143:dbl)
        n619 = property on="X Step SP" class="DigNum (strict)"() -> ("Maximum"=w1148:dbl)  [unwired: 2 in, 2 out]
        n620 = property on="X Step SP" class="DigNum (strict)"() -> ("Minimum"=w1147:dbl)  [unwired: 2 in, 2 out]
        n621 = In Range and Coerce(upper limit=w1141, x=w1143, lower limit=w1140) -> (coerced(x)=w1142:dbl)  [unwired: 1 out]
        n622 = To Long Integer(number=w1142) -> (32bit integer=w1144:i32)
        n623 = In Range and Coerce(upper limit=w1148, x=w1150, lower limit=w1147) -> (coerced(x)=w1149:dbl)  [unwired: 1 out]
        n624 = To Long Integer(number=w1149) -> (32bit integer=w1153:i32)
        n625 = property on="X Velocity SP step/sec" class="DigNum (strict)"("Val(Sgnl)"=w1144) -> ()  [unwired: 2 in, 2 out]
        n626 = property on="X Step SP" class="DigNum (strict)"("Val(Sgnl)"=w1153) -> ()  [unwired: 2 in, 2 out]
      }
      event #6 {
        n627 = event-data() -> ()  [unwired: 1 in, 7 out]
        n628 = property on="Z steps/rev" class="DigNum (strict)"() -> ("Value"=w1171:u32)  [unwired: 2 in, 2 out]
        n629 = property on="Z offset mm" class="DigNum (strict)"() -> ("Value"=w1169:dbl)  [unwired: 2 in, 2 out]
        n630 = property on="Z Position SP mm" class="DigNum (strict)"() -> ("Value"=w1168:dbl)  [unwired: 2 in, 2 out]
        n631 = property on="Z Velocity SP step/sec" class="DigNum (strict)"() -> ("Maximum"=w1158:dbl)  [unwired: 2 in, 2 out]
        n632 = property on="Z Velocity SP step/sec" class="DigNum (strict)"() -> ("Minimum"=w1157:dbl)  [unwired: 2 in, 2 out]
        n633 = Subtract(x=w1168, y=w1169) -> (x-y=w1172:dbl)
        n634 = property on="Z Velocity SP mm/sec" class="DigNum (strict)"() -> ("Value"=w1162:dbl)  [unwired: 2 in, 2 out]
        n635 = property on="Z mm/rev" class="DigNum (strict)"() -> ("Value"=w1174:dbl)  [unwired: 2 in, 2 out]
        n636 = Divide(x=w1172, y=w1174) -> (x/y=w1173:dbl)
        n637 = Divide(x=w1162, y=w1174) -> (x/y=w1163:dbl)
        n638 = To Double Precision Float(number=w1171) -> (double precision float=w1175:dbl)
        n639 = Multiply(x=w1173, y=w1175) -> (x*y=w1167:dbl)
        n640 = Multiply(x=w1163, y=w1175) -> (x*y=w1160:dbl)
        n641 = property on="Z Step SP" class="DigNum (strict)"() -> ("Maximum"=w1165:dbl)  [unwired: 2 in, 2 out]
        n642 = property on="Z Step SP" class="DigNum (strict)"() -> ("Minimum"=w1164:dbl)  [unwired: 2 in, 2 out]
        n643 = In Range and Coerce(upper limit=w1158, x=w1160, lower limit=w1157) -> (coerced(x)=w1159:dbl)  [unwired: 1 out]
        n644 = To Long Integer(number=w1159) -> (32bit integer=w1161:i32)
        n645 = In Range and Coerce(upper limit=w1165, x=w1167, lower limit=w1164) -> (coerced(x)=w1166:dbl)  [unwired: 1 out]
        n646 = To Long Integer(number=w1166) -> (32bit integer=w1170:i32)
        n647 = property on="Z Velocity SP step/sec" class="DigNum (strict)"("Val(Sgnl)"=w1161) -> ()  [unwired: 2 in, 2 out]
        n648 = property on="Z Step SP" class="DigNum (strict)"("Val(Sgnl)"=w1170) -> ()  [unwired: 2 in, 2 out]
      }
      event #7 {
        n649 = event-data() -> ()  [unwired: 1 in, 7 out]
        n650 = property on="R steps/rev" class="DigNum (strict)"() -> ("Value"=w1192:u32)  [unwired: 2 in, 2 out]
        n651 = property on="R offset deg" class="DigNum (strict)"() -> ("Value"=w1190:dbl)  [unwired: 2 in, 2 out]
        n652 = property on="R Position SP deg" class="DigNum (strict)"() -> ("Value"=w1189:dbl)  [unwired: 2 in, 2 out]
        n653 = property on="R Velocity SP step/sec" class="DigNum (strict)"() -> ("Maximum"=w1179:dbl)  [unwired: 2 in, 2 out]
        n654 = property on="R Velocity SP step/sec" class="DigNum (strict)"() -> ("Minimum"=w1178:dbl)  [unwired: 2 in, 2 out]
        n655 = Subtract(x=w1189, y=w1190) -> (x-y=w1193:dbl)
        n656 = property on="R Velocity SP deg/sec" class="DigNum (strict)"() -> ("Value"=w1183:dbl)  [unwired: 2 in, 2 out]
        n657 = property on="R deg/rev" class="DigNum (strict)"() -> ("Value"=w1176:dbl)  [unwired: 2 in, 2 out]
        n658 = Divide(x=w1193, y=w1176) -> (x/y=w1194:dbl)
        n659 = Divide(x=w1183, y=w1176) -> (x/y=w1184:dbl)
        n660 = To Double Precision Float(number=w1192) -> (double precision float=w1177:dbl)
        n661 = Multiply(x=w1194, y=w1177) -> (x*y=w1188:dbl)
        n662 = Multiply(x=w1184, y=w1177) -> (x*y=w1181:dbl)
        n663 = property on="R Step SP" class="DigNum (strict)"() -> ("Maximum"=w1186:dbl)  [unwired: 2 in, 2 out]
        n664 = property on="R Step SP" class="DigNum (strict)"() -> ("Minimum"=w1185:dbl)  [unwired: 2 in, 2 out]
        n665 = In Range and Coerce(upper limit=w1179, x=w1181, lower limit=w1178) -> (coerced(x)=w1180:dbl)  [unwired: 1 out]
        n666 = To Long Integer(number=w1180) -> (32bit integer=w1182:i32)
        n667 = In Range and Coerce(upper limit=w1186, x=w1188, lower limit=w1185) -> (coerced(x)=w1187:dbl)  [unwired: 1 out]
        n668 = To Long Integer(number=w1187) -> (32bit integer=w1191:i32)
        n669 = property on="R Velocity SP step/sec" class="DigNum (strict)"("Val(Sgnl)"=w1182) -> ()  [unwired: 2 in, 2 out]
        n670 = property on="R Step SP" class="DigNum (strict)"("Val(Sgnl)"=w1191) -> ()  [unwired: 2 in, 2 out]
      }
      event #8 {
        n671 = event-data() -> ()  [unwired: 1 in, 7 out]
        n672 = property on="Y steps/rev" class="DigNum (strict)"() -> ("Value"=w1210:u32)  [unwired: 2 in, 2 out]
        n673 = property on="Y mm/rev" class="DigNum (strict)"() -> ("Value"=w1195:dbl)  [unwired: 2 in, 2 out]
        n674 = property on="Y Scan Length SP mm" class="DigNum (strict)"() -> ("Value"=w1208:dbl)  [unwired: 2 in, 2 out]
        n675 = property on="Y Scan Velocity SP mm/sec" class="DigNum (strict)"() -> ("Value"=w1202:dbl)  [unwired: 2 in, 2 out]
        n676 = property on="Y Scan Velocity SP steps/sec" class="DigNum (strict)"() -> ("Maximum"=w1198:dbl)  [unwired: 2 in, 2 out]
        n677 = property on="Y Scan Velocity SP steps/sec" class="DigNum (strict)"() -> ("Minimum"=w1197:dbl)  [unwired: 2 in, 2 out]
        n678 = Divide(x=w1208, y=w1195) -> (x/y=w1211:dbl)
        n679 = Divide(x=w1202, y=w1195) -> (x/y=w1203:dbl)
        n680 = To Double Precision Float(number=w1210) -> (double precision float=w1196:dbl)
        n681 = Multiply(x=w1211, y=w1196) -> (x*y=w1207:dbl)
        n682 = Multiply(x=w1203, y=w1196) -> (x*y=w1200:dbl)
        n683 = property on="Y Step SP" class="DigNum (strict)"() -> ("Maximum"=w1204:dbl)  [unwired: 2 in, 2 out]
        n684 = property on="Y Step SP" class="DigNum (strict)"() -> ("Minimum"=w1205:dbl)  [unwired: 2 in, 2 out]
        n685 = In Range and Coerce(upper limit=w1198, x=w1200, lower limit=w1197) -> (coerced(x)=w1199:dbl)  [unwired: 1 out]
        n686 = To Long Integer(number=w1199) -> (32bit integer=w1201:i32)
        n687 = In Range and Coerce(upper limit=w1204, x=w1207, lower limit=w1205) -> (coerced(x)=w1206:dbl)  [unwired: 1 out]
        n688 = To Long Integer(number=w1206) -> (32bit integer=w1209:i32)
        n689 = property on="Y Scan Velocity SP steps/sec" class="DigNum (strict)"("Val(Sgnl)"=w1201) -> ()  [unwired: 2 in, 2 out]
        n690 = property on="Y Scan Length SP steps" class="DigNum (strict)"("Val(Sgnl)"=w1209) -> ()  [unwired: 2 in, 2 out]
      }
      event #9 {
        n691 = event-data() -> ()  [unwired: 1 in, 7 out]
        n692 = property on="X steps/rev" class="DigNum (strict)"() -> ("Value"=w1227:u32)  [unwired: 2 in, 2 out]
        n693 = property on="X mm/rev" class="DigNum (strict)"() -> ("Value"=w1212:dbl)  [unwired: 2 in, 2 out]
        n694 = property on="X Scan Length SP mm" class="DigNum (strict)"() -> ("Value"=w1225:dbl)  [unwired: 2 in, 2 out]
        n695 = property on="X Scan Velocity SP mm/sec" class="DigNum (strict)"() -> ("Value"=w1219:dbl)  [unwired: 2 in, 2 out]
        n696 = property on="X Scan Velocity SP steps/sec" class="DigNum (strict)"() -> ("Maximum"=w1215:dbl)  [unwired: 2 in, 2 out]
        n697 = property on="X Scan Velocity SP steps/sec" class="DigNum (strict)"() -> ("Minimum"=w1214:dbl)  [unwired: 2 in, 2 out]
        n698 = Divide(x=w1225, y=w1212) -> (x/y=w1228:dbl)
        n699 = Divide(x=w1219, y=w1212) -> (x/y=w1220:dbl)
        n700 = To Double Precision Float(number=w1227) -> (double precision float=w1213:dbl)
        n701 = Multiply(x=w1228, y=w1213) -> (x*y=w1224:dbl)
        n702 = Multiply(x=w1220, y=w1213) -> (x*y=w1217:dbl)
        n703 = property on="X Step SP" class="DigNum (strict)"() -> ("Maximum"=w1221:dbl)  [unwired: 2 in, 2 out]
        n704 = property on="X Step SP" class="DigNum (strict)"() -> ("Minimum"=w1222:dbl)  [unwired: 2 in, 2 out]
        n705 = In Range and Coerce(upper limit=w1215, x=w1217, lower limit=w1214) -> (coerced(x)=w1216:dbl)  [unwired: 1 out]
        n706 = To Long Integer(number=w1216) -> (32bit integer=w1218:i32)
        n707 = In Range and Coerce(upper limit=w1221, x=w1224, lower limit=w1222) -> (coerced(x)=w1223:dbl)  [unwired: 1 out]
        n708 = To Long Integer(number=w1223) -> (32bit integer=w1226:i32)
        n709 = property on="X Scan Velocity SP steps/sec" class="DigNum (strict)"("Val(Sgnl)"=w1218) -> ()  [unwired: 2 in, 2 out]
        n710 = property on="X Scan Length SP steps" class="DigNum (strict)"("Val(Sgnl)"=w1226) -> ()  [unwired: 2 in, 2 out]
      }
      event #10 {
        n711 = event-data() -> ()  [unwired: 1 in, 7 out]
        n712 = property on="Z steps/rev" class="DigNum (strict)"() -> ("Value"=w1244:u32)  [unwired: 2 in, 2 out]
        n713 = property on="Z mm/rev" class="DigNum (strict)"() -> ("Value"=w1229:dbl)  [unwired: 2 in, 2 out]
        n714 = property on="Z Scan Length SP mm" class="DigNum (strict)"() -> ("Value"=w1242:dbl)  [unwired: 2 in, 2 out]
        n715 = property on="Z Scan Velocity SP mm/sec" class="DigNum (strict)"() -> ("Value"=w1236:dbl)  [unwired: 2 in, 2 out]
        n716 = property on="Z Scan Velocity SP steps/sec" class="DigNum (strict)"() -> ("Maximum"=w1232:dbl)  [unwired: 2 in, 2 out]
        n717 = property on="Z Scan Velocity SP steps/sec" class="DigNum (strict)"() -> ("Minimum"=w1231:dbl)  [unwired: 2 in, 2 out]
        n718 = Divide(x=w1242, y=w1229) -> (x/y=w1245:dbl)
        n719 = Divide(x=w1236, y=w1229) -> (x/y=w1237:dbl)
        n720 = To Double Precision Float(number=w1244) -> (double precision float=w1230:dbl)
        n721 = Multiply(x=w1245, y=w1230) -> (x*y=w1241:dbl)
        n722 = Multiply(x=w1237, y=w1230) -> (x*y=w1234:dbl)
        n723 = property on="Z Step SP" class="DigNum (strict)"() -> ("Maximum"=w1238:dbl)  [unwired: 2 in, 2 out]
        n724 = property on="Z Step SP" class="DigNum (strict)"() -> ("Minimum"=w1239:dbl)  [unwired: 2 in, 2 out]
        n725 = In Range and Coerce(upper limit=w1232, x=w1234, lower limit=w1231) -> (coerced(x)=w1233:dbl)  [unwired: 1 out]
        n726 = To Long Integer(number=w1233) -> (32bit integer=w1235:i32)
        n727 = In Range and Coerce(upper limit=w1238, x=w1241, lower limit=w1239) -> (coerced(x)=w1240:dbl)  [unwired: 1 out]
        n728 = To Long Integer(number=w1240) -> (32bit integer=w1243:i32)
        n729 = property on="Z Scan Velocity SP steps/sec" class="DigNum (strict)"("Val(Sgnl)"=w1235) -> ()  [unwired: 2 in, 2 out]
        n730 = property on="Z Scan Length SP steps" class="DigNum (strict)"("Val(Sgnl)"=w1243) -> ()  [unwired: 2 in, 2 out]
      }
      event #11 {
        n731 = event-data() -> ()  [unwired: 1 in, 7 out]
        n732 = property on="R steps/rev" class="DigNum (strict)"() -> ("Value"=w1261:u32)  [unwired: 2 in, 2 out]
        n733 = property on="R Velocity SP step/sec" class="DigNum (strict)"() -> ("Maximum"=w1249:dbl)  [unwired: 2 in, 2 out]
        n734 = property on="R Scan Length SP deg" class="DigNum (strict)"() -> ("Value"=w1259:dbl)  [unwired: 2 in, 2 out]
        n735 = property on="R deg/rev" class="DigNum (strict)"() -> ("Value"=w1246:dbl)  [unwired: 2 in, 2 out]
        n736 = property on="R Scan Velocity SP steps/sec" class="DigNum (strict)"() -> ("Minimum"=w1248:dbl)  [unwired: 2 in, 2 out]
        n737 = property on="R Scan Velocity SP deg/sec" class="DigNum (strict)"() -> ("Value"=w1253:dbl)  [unwired: 2 in, 2 out]
        n738 = Divide(x=w1259, y=w1246) -> (x/y=w1262:dbl)
        n739 = To Double Precision Float(number=w1261) -> (double precision float=w1247:dbl)
        n740 = Multiply(x=w1262, y=w1247) -> (x*y=w1258:dbl)
        n741 = Divide(x=w1253, y=w1246) -> (x/y=w1254:dbl)
        n742 = property on="R Step SP" class="DigNum (strict)"() -> ("Maximum"=w1255:dbl)  [unwired: 2 in, 2 out]
        n743 = property on="R Step SP" class="DigNum (strict)"() -> ("Minimum"=w1256:dbl)  [unwired: 2 in, 2 out]
        n744 = Multiply(x=w1254, y=w1247) -> (x*y=w1251:dbl)
        n745 = In Range and Coerce(upper limit=w1255, x=w1258, lower limit=w1256) -> (coerced(x)=w1257:dbl)  [unwired: 1 out]
        n746 = In Range and Coerce(upper limit=w1249, x=w1251, lower limit=w1248) -> (coerced(x)=w1250:dbl)  [unwired: 1 out]
        n747 = To Long Integer(number=w1257) -> (32bit integer=w1260:i32)
        n748 = To Long Integer(number=w1250) -> (32bit integer=w1252:i32)
        n749 = property on="R Scan Length SP steps" class="DigNum (strict)"("Val(Sgnl)"=w1260) -> ()  [unwired: 2 in, 2 out]
        n750 = property on="R Scan Velocity SP steps/sec" class="DigNum (strict)"("Val(Sgnl)"=w1252) -> ()  [unwired: 2 in, 2 out]
      }
      event #12 {
        n751 = event-data() -> ()  [unwired: 1 in, 7 out]
        n752 = flat-sequence {
          tunnel: w1267 -> [w1277]
          tunnel: w1268 -> [w1278]
          tunnel: [w1278] -> w1264
          tunnel: [w1277] -> w1263
          tunnel: [w1281] -> w1266
          tunnel: [w1280] -> w1265
          tunnel: w1264 -> [w1283]
          tunnel: w1263 -> [w1282]
          tunnel: [w1301] -> w1270
          tunnel: [w1300] -> w1269
          tunnel: w1266 -> [w1299]
          tunnel: w1265 -> [w1298]
          tunnel: [w1308] -> w1272
          tunnel: [w1307] -> w1271
          tunnel: w1270 -> [w1306]
          tunnel: w1269 -> [w1305]
          tunnel: [w1314] -> w1273
          tunnel: [w1315] -> w1274
          tunnel: w1272 -> [w1315]
          tunnel: w1271 -> [w1313]
          frame #0 {
            n753 = property on="Scan Go" class="Bool"("DisabledEnum"=T1."Disabled and Grayed Out" ("Disabled")) -> ()  [unwired: 2 in, 2 out]
            n754 = property on="Y Go" class="Bool"("DisabledEnum"=T1."Disabled and Grayed Out" ("Disabled")) -> ()  [unwired: 2 in, 2 out]
          }
          frame #1 {
            n755 = property on="Y Step SP" class="DigNum (strict)"() -> ("Value"=w1291:i32)  [unwired: 2 in, 2 out]
            n756 = property on="Y Step PV" class="DigNum (strict)"() -> ("Value"=w1290:i32)  [unwired: 2 in, 2 out]
            n757 = property on="Y Backlash" class="DigNum (strict)"() -> ("Value"=w1279:i32)  [unwired: 2 in, 2 out]
            n758 = Subtract(x=w1291, y=w1290) -> (x-y=w1289:i32)
            n759 = Sign(1:w1279) -> (0:w1287:i32)
            n760 = Sign(1:w1289) -> (0:w1288:i32)
            n761 = Multiply(x=w1288, y=w1287) -> (x*y=w1286:i32)
            n762 = Equal?(x=w1286, y=1) -> (x = y?=w1284:bool)
            n763 = case shown="False" w1284 {
              tunnel: w1283 -> [w1294 w1296]
              tunnel: w1282 -> [w1293 w1295]
              tunnel: [w1293 w1295] -> w1281
              tunnel: [w1294 w1296] -> w1280
              frame #0 {
                n764 = property on="Y Backlash corr" class="Bool (strict)"("Val(Sgnl)"=FALSE ("Value (Signaling)")) -> ()  [unwired: 2 in, 2 out]
              }
              frame #1 {
                n765 = property on="Y Backlash corr" class="Bool (strict)"("Val(Sgnl)"=TRUE ("Value (Signaling)")) -> ()  [unwired: 2 in, 2 out]
              }
            }
          }
          frame #2 {
            # "Velocity Setting"
            n766 = property on="Y Velocity SP step/sec" class="DigNum (strict)"() -> ("Value"=w1302:i32)  [unwired: 2 in, 2 out]
            n767 = Number To Decimal String(number=w1302) -> (decimal integer string=w1303:string)  [unwired: 1 in]
            n768 = call "mDrive Send Command.vi"("error in (no error)"=w1299, "Extra"=w1303, "Command"=T2."Max Velocity", "VISA resource name"=w1298) -> ("error out"=w1300:errorcluster, "VISA resource name out"=w1301:refnum<visa-resource-name>)  [unwired: 3 in, 1 out]
          }
          frame #3 {
            # "Move to Abs Position"
            n769 = property on="Y Step SP" class="DigNum (strict)"() -> ("Value"=w1311:i32)  [unwired: 2 in, 2 out]
            n770 = Number To Decimal String(number=w1311) -> (decimal integer string=w1310:string)  [unwired: 1 in]
            n771 = call "mDrive Send Command.vi"("error in (no error)"=w1305, "Extra"=w1310, "Command"=T2."Move to Absolute Position", "VISA resource name"=w1306) -> ("error out"=w1307:errorcluster, "VISA resource name out"=w1308:refnum<visa-resource-name>)  [unwired: 3 in, 1 out]
          }
          frame #4 {
            n772 = call "Time Delay"("error in (no error)"=w1313, "Delay Time (s)"=0.1) -> ("error out"=w1314:errorcluster)  [unwired: 9 in]
          }
        }
      }
      event #13 {
        n773 = event-data() -> ()  [unwired: 1 in, 7 out]
        n774 = flat-sequence {
          tunnel: w1318 -> [w1330]
          tunnel: w1319 -> [w1331]
          tunnel: [w1331] -> w1321
          tunnel: [w1330] -> w1320
          tunnel: [w1334] -> w1323
          tunnel: [w1333] -> w1322
          tunnel: w1321 -> [w1336]
          tunnel: w1320 -> [w1335]
          tunnel: [w1354] -> w1325
          tunnel: [w1353] -> w1324
          tunnel: w1323 -> [w1352]
          tunnel: w1322 -> [w1351]
          tunnel: [w1361] -> w1327
          tunnel: [w1360] -> w1326
          tunnel: w1325 -> [w1359]
          tunnel: w1324 -> [w1358]
          tunnel: [w1367] -> w1317
          tunnel: [w1368] -> w1316
          tunnel: w1327 -> [w1368]
          tunnel: w1326 -> [w1366]
          frame #0 {
            n775 = property on="Scan Go" class="Bool"("DisabledEnum"=T1."Disabled and Grayed Out" ("Disabled")) -> ()  [unwired: 2 in, 2 out]
            n776 = property on="Z Go" class="Bool"("DisabledEnum"=T1."Disabled and Grayed Out" ("Disabled")) -> ()  [unwired: 2 in, 2 out]
          }
          frame #1 {
            n777 = property on="Z Step SP" class="DigNum (strict)"() -> ("Value"=w1344:i32)  [unwired: 2 in, 2 out]
            n778 = property on="Z Step PV" class="DigNum (strict)"() -> ("Value"=w1343:i32)  [unwired: 2 in, 2 out]
            n779 = property on="Z Backlash" class="DigNum (strict)"() -> ("Value"=w1332:i32)  [unwired: 2 in, 2 out]
            n780 = Subtract(x=w1344, y=w1343) -> (x-y=w1342:i32)
            n781 = Sign(1:w1332) -> (0:w1340:i32)
            n782 = Sign(1:w1342) -> (0:w1341:i32)
            n783 = Multiply(x=w1341, y=w1340) -> (x*y=w1339:i32)
            n784 = Equal?(x=w1339, y=1) -> (x = y?=w1337:bool)
            n785 = case shown="True" w1337 {
              tunnel: w1336 -> [w1347 w1349]
              tunnel: w1335 -> [w1346 w1348]
              tunnel: [w1346 w1348] -> w1334
              tunnel: [w1347 w1349] -> w1333
              frame #0 {
                n786 = property on="Z Backlash corr" class="Bool (strict)"("Val(Sgnl)"=FALSE ("Value (Signaling)")) -> ()  [unwired: 2 in, 2 out]
              }
              frame #1 {
                n787 = property on="Z Backlash corr" class="Bool (strict)"("Val(Sgnl)"=TRUE ("Value (Signaling)")) -> ()  [unwired: 2 in, 2 out]
              }
            }
          }
          frame #2 {
            # "Velocity Setting"
            n788 = property on="Z Velocity SP step/sec" class="DigNum (strict)"() -> ("Value"=w1355:i32)  [unwired: 2 in, 2 out]
            n789 = Number To Decimal String(number=w1355) -> (decimal integer string=w1356:string)  [unwired: 1 in]
            n790 = call "mDrive Send Command.vi"("error in (no error)"=w1352, "Extra"=w1356, "Command"=T2."Max Velocity", "VISA resource name"=w1351) -> ("error out"=w1353:errorcluster, "VISA resource name out"=w1354:refnum<visa-resource-name>)  [unwired: 3 in, 1 out]
          }
          frame #3 {
            # "Move to Abs Position"
            n791 = property on="Z Step SP" class="DigNum (strict)"() -> ("Value"=w1364:i32)  [unwired: 2 in, 2 out]
            n792 = Number To Decimal String(number=w1364) -> (decimal integer string=w1363:string)  [unwired: 1 in]
            n793 = call "mDrive Send Command.vi"("error in (no error)"=w1358, "Extra"=w1363, "Command"=T2."Move to Absolute Position", "VISA resource name"=w1359) -> ("error out"=w1360:errorcluster, "VISA resource name out"=w1361:refnum<visa-resource-name>)  [unwired: 3 in, 1 out]
          }
          frame #4 {
            n794 = call "Time Delay28"("error in (no error)"=w1366, "Delay Time (s)"=0.1) -> ("error out"=w1367:errorcluster)  [unwired: 9 in]
          }
        }
      }
      event #14 {
        n795 = event-data() -> ()  [unwired: 1 in, 7 out]
        n796 = flat-sequence {
          tunnel: w1371 -> [w1383]
          tunnel: w1372 -> [w1384]
          tunnel: [w1384] -> w1374
          tunnel: [w1383] -> w1373
          tunnel: [w1387] -> w1376
          tunnel: [w1386] -> w1375
          tunnel: w1374 -> [w1389]
          tunnel: w1373 -> [w1388]
          tunnel: [w1407] -> w1378
          tunnel: [w1406] -> w1377
          tunnel: w1376 -> [w1405]
          tunnel: w1375 -> [w1404]
          tunnel: [w1414] -> w1380
          tunnel: [w1413] -> w1379
          tunnel: w1378 -> [w1412]
          tunnel: w1377 -> [w1411]
          tunnel: [w1420] -> w1370
          tunnel: [w1421] -> w1369
          tunnel: w1380 -> [w1421]
          tunnel: w1379 -> [w1419]
          frame #0 {
            n797 = property on="Scan Go" class="Bool"("DisabledEnum"=T1."Disabled and Grayed Out" ("Disabled")) -> ()  [unwired: 2 in, 2 out]
            n798 = property on="R Go" class="Bool"("DisabledEnum"=T1."Disabled and Grayed Out" ("Disabled")) -> ()  [unwired: 2 in, 2 out]
          }
          frame #1 {
            n799 = property on="R Step SP" class="DigNum (strict)"() -> ("Value"=w1397:i32)  [unwired: 2 in, 2 out]
            n800 = property on="R Step PV" class="DigNum (strict)"() -> ("Value"=w1396:i32)  [unwired: 2 in, 2 out]
            n801 = property on="R Backlash" class="DigNum (strict)"() -> ("Value"=w1385:i32)  [unwired: 2 in, 2 out]
            n802 = Subtract(x=w1397, y=w1396) -> (x-y=w1395:i32)
            n803 = Sign(1:w1385) -> (0:w1393:i32)
            n804 = Sign(1:w1395) -> (0:w1394:i32)
            n805 = Multiply(x=w1394, y=w1393) -> (x*y=w1392:i32)
            n806 = Equal?(x=w1392, y=1) -> (x = y?=w1390:bool)
            n807 = case shown="True" w1390 {
              tunnel: w1389 -> [w1400 w1402]
              tunnel: w1388 -> [w1399 w1401]
              tunnel: [w1399 w1401] -> w1387
              tunnel: [w1400 w1402] -> w1386
              frame #0 {
                n808 = property on="R Backlash corr" class="Bool (strict)"("Val(Sgnl)"=FALSE ("Value (Signaling)")) -> ()  [unwired: 2 in, 2 out]
              }
              frame #1 {
                n809 = property on="R Backlash corr" class="Bool (strict)"("Val(Sgnl)"=TRUE ("Value (Signaling)")) -> ()  [unwired: 2 in, 2 out]
              }
            }
          }
          frame #2 {
            # "Velocity Setting"
            n810 = property on="R Velocity SP step/sec" class="DigNum (strict)"() -> ("Value"=w1408:i32)  [unwired: 2 in, 2 out]
            n811 = Number To Decimal String(number=w1408) -> (decimal integer string=w1409:string)  [unwired: 1 in]
            n812 = call "mDrive Send Command.vi"("error in (no error)"=w1405, "Extra"=w1409, "Command"=T2."Max Velocity", "VISA resource name"=w1404) -> ("error out"=w1406:errorcluster, "VISA resource name out"=w1407:refnum<visa-resource-name>)  [unwired: 3 in, 1 out]
          }
          frame #3 {
            # "Move to Abs Position"
            n813 = property on="R Step SP" class="DigNum (strict)"() -> ("Value"=w1417:i32)  [unwired: 2 in, 2 out]
            n814 = Number To Decimal String(number=w1417) -> (decimal integer string=w1416:string)  [unwired: 1 in]
            n815 = call "mDrive Send Command.vi"("error in (no error)"=w1411, "Extra"=w1416, "Command"=T2."Move to Absolute Position", "VISA resource name"=w1412) -> ("error out"=w1413:errorcluster, "VISA resource name out"=w1414:refnum<visa-resource-name>)  [unwired: 3 in, 1 out]
          }
          frame #4 {
            n816 = call "Time Delay29"("error in (no error)"=w1419, "Delay Time (s)"=0.1) -> ("error out"=w1420:errorcluster)  [unwired: 9 in]
          }
        }
      }
      event #15 {
        n817 = event-data() -> ()  [unwired: 1 in, 7 out]
        n818 = flat-sequence {
          tunnel: [w1435] -> w1427
          tunnel: [w1434] -> w1426
          tunnel: w1425 -> [w1435]
          tunnel: w1424 -> [w1434]
          tunnel: [w1440] -> w1429
          tunnel: [w1439] -> w1428
          tunnel: w1427 -> [w1442]
          tunnel: w1426 -> [w1441]
          tunnel: [w1460] -> w1431
          tunnel: [w1459] -> w1430
          tunnel: w1429 -> [w1458]
          tunnel: w1428 -> [w1457]
          tunnel: [w1467] -> w1433
          tunnel: [w1466] -> w1432
          tunnel: w1431 -> [w1465]
          tunnel: w1430 -> [w1464]
          tunnel: [w1473] -> w1422
          tunnel: [w1474] -> w1423
          tunnel: w1433 -> [w1474]
          tunnel: w1432 -> [w1472]
          frame #0 {
            n819 = property on="Scan Go" class="Bool"("DisabledEnum"=T1."Disabled and Grayed Out" ("Disabled")) -> ()  [unwired: 2 in, 2 out]
            n820 = property on="X Go" class="Bool"("DisabledEnum"=T1."Disabled and Grayed Out" ("Disabled")) -> ()  [unwired: 2 in, 2 out]
          }
          frame #1 {
            n821 = property on="X Step SP" class="DigNum (strict)"() -> ("Value"=w1450:i32)  [unwired: 2 in, 2 out]
            n822 = property on="X Step PV" class="DigNum (strict)"() -> ("Value"=w1449:i32)  [unwired: 2 in, 2 out]
            n823 = property on="X Backlash" class="DigNum (strict)"() -> ("Value"=w1438:i32)  [unwired: 2 in, 2 out]
            n824 = Subtract(x=w1450, y=w1449) -> (x-y=w1448:i32)
            n825 = Sign(1:w1438) -> (0:w1446:i32)
            n826 = Sign(1:w1448) -> (0:w1447:i32)
            n827 = Multiply(x=w1447, y=w1446) -> (x*y=w1445:i32)
            n828 = Equal?(x=w1445, y=1) -> (x = y?=w1443:bool)
            n829 = case shown="True" w1443 {
              tunnel: w1442 -> [w1453 w1455]
              tunnel: w1441 -> [w1452 w1454]
              tunnel: [w1452 w1454] -> w1440
              tunnel: [w1453 w1455] -> w1439
              frame #0 {
                n830 = property on="X Backlash corr" class="Bool (strict)"("Val(Sgnl)"=FALSE ("Value (Signaling)")) -> ()  [unwired: 2 in, 2 out]
              }
              frame #1 {
                n831 = property on="X Backlash corr" class="Bool (strict)"("Val(Sgnl)"=TRUE ("Value (Signaling)")) -> ()  [unwired: 2 in, 2 out]
              }
            }
          }
          frame #2 {
            # "Velocity Setting"
            n832 = property on="X Velocity SP step/sec" class="DigNum (strict)"() -> ("Value"=w1461:i32)  [unwired: 2 in, 2 out]
            n833 = Number To Decimal String(number=w1461) -> (decimal integer string=w1462:string)  [unwired: 1 in]
            n834 = call "mDrive Send Command.vi"("error in (no error)"=w1458, "Extra"=w1462, "Command"=T2."Max Velocity", "VISA resource name"=w1457) -> ("error out"=w1459:errorcluster, "VISA resource name out"=w1460:refnum<visa-resource-name>)  [unwired: 3 in, 1 out]
          }
          frame #3 {
            # "Move to Abs Position"
            n835 = property on="X Step SP" class="DigNum (strict)"() -> ("Value"=w1470:i32)  [unwired: 2 in, 2 out]
            n836 = Number To Decimal String(number=w1470) -> (decimal integer string=w1469:string)  [unwired: 1 in]
            n837 = call "mDrive Send Command.vi"("error in (no error)"=w1464, "Extra"=w1469, "Command"=T2."Move to Absolute Position", "VISA resource name"=w1465) -> ("error out"=w1466:errorcluster, "VISA resource name out"=w1467:refnum<visa-resource-name>)  [unwired: 3 in, 1 out]
          }
          frame #4 {
            n838 = call "Time Delay15"("error in (no error)"=w1472, "Delay Time (s)"=0.1) -> ("error out"=w1473:errorcluster)  [unwired: 9 in]
          }
        }
      }
      event #16 {
        n839 = event-data() -> ()  [unwired: 1 in, 7 out]
        n840 = flat-sequence {
          tunnel: [w1490] -> w1482
          tunnel: [w1488] -> w1481
          tunnel: w1480 -> [w1484]
          tunnel: w1479 -> [w1483]
          tunnel: w1482 -> [w1505]
          tunnel: w1481 -> [w1504]
          tunnel: [w1505] -> w1476
          tunnel: [w1504] -> w1475
          tunnel: [w1507] -> w1477
          tunnel: [w1508] -> w1478
          tunnel: w1476 -> [w1508]
          tunnel: w1475 -> [w1507]
          frame #0 {
            # "VELOCITY"
            n841 = property on="X Scan Velocity SP steps/sec" class="DigNum (strict)"() -> ("Value"=w1491:i32)  [unwired: 2 in, 2 out]
            n842 = Number To Decimal String(number=w1491) -> (decimal integer string=w1492:string)  [unwired: 1 in]
            n843 = call "mDrive Send Command.vi"("error in (no error)"=w1483, "Extra"=w1492, "Command"=T2."Max Velocity", "VISA resource name"=w1484) -> ("error out"=w1493:errorcluster, "VISA resource name out"=w1498:refnum<visa-resource-name>)  [unwired: 3 in, 1 out]
            n844 = call "Time Delay9"("error in (no error)"=w1493) -> ("error out"=w1496:errorcluster)  [unwired: 10 in]
            n845 = call "mDrive Send Command.vi"("error in (no error)"=w1496, "Extra"="VM", "Command"=T2."Print Parameter", "VISA resource name"=w1498) -> ("error out"=w1489:errorcluster, "read buffer"=w1494:string, "VISA resource name out"=w1490:refnum<visa-resource-name>)  [unwired: 3 in]
            n846 = call "Time Delay10"("error in (no error)"=w1489) -> ("error out"=w1488:errorcluster)  [unwired: 10 in]
            n847 = Decimal String To Number(string=w1494, offset=0) -> (number=w1497:i32)  [unwired: 1 in, 1 out]
            n848 = property on="X velocity PV step/sec" class="DigNum (strict)"("Val(Sgnl)"=w1497) -> ()  [unwired: 2 in, 2 out]
          }
          frame #1 {
            n849 = property on="X Scan" class="Bool (strict)"("Val(Sgnl)"=TRUE ("Slew Ready 2")) -> ()  [unwired: 2 in, 2 out]
            n850 = property on="Scan Go" class="Bool"("DisabledEnum"=T1."Enabled" ("Disabled")) -> ()  [unwired: 2 in, 2 out]
            n851 = property on="Scan Cancel" class="Bool"("DisabledEnum"=T1."Enabled" ("Disabled")) -> ()  [unwired: 2 in, 2 out]
            n852 = property on="X Scan Length SP steps" class="DigNum (strict)"("DisabledEnum"=T1."Disabled and Grayed Out" ("Disabled")) -> ()  [unwired: 2 in, 2 out]
            n853 = property on="X Scan Velocity SP steps/sec" class="DigNum (strict)"("DisabledEnum"=T1."Disabled and Grayed Out" ("Disabled")) -> ()  [unwired: 2 in, 2 out]
          }
          frame #2 {
            n854 = property on="X Go" class="Bool"("DisabledEnum"=T1."Disabled and Grayed Out" ("Disabled")) -> ()  [unwired: 2 in, 2 out]
          }
        }
      }
      event #17 {
        n855 = event-data() -> ()  [unwired: 1 in, 7 out]
        n856 = flat-sequence {
          tunnel: w1516 -> [w1526]
          tunnel: w1515 -> [w1525]
          tunnel: [w1522] -> w1513
          tunnel: [w1520] -> w1512
          tunnel: w1513 -> [w1539]
          tunnel: w1512 -> [w1538]
          tunnel: [w1539] -> w1510
          tunnel: [w1538] -> w1509
          tunnel: [w1541] -> w1514
          tunnel: [w1542] -> w1511
          tunnel: w1510 -> [w1542]
          tunnel: w1509 -> [w1541]
          frame #0 {
            # "VELOCITY"
            n857 = property on="Y Scan Velocity SP steps/sec" class="DigNum (strict)"() -> ("Value"=w1523:i32)  [unwired: 2 in, 2 out]
            n858 = Number To Decimal String(number=w1523) -> (decimal integer string=w1524:string)  [unwired: 1 in]
            n859 = call "mDrive Send Command.vi"("error in (no error)"=w1526, "Extra"=w1524, "Command"=T2."Max Velocity", "VISA resource name"=w1525) -> ("error out"=w1527:errorcluster, "VISA resource name out"=w1532:refnum<visa-resource-name>)  [unwired: 3 in, 1 out]
            n860 = call "Time Delay5"("error in (no error)"=w1527) -> ("error out"=w1530:errorcluster)  [unwired: 10 in]
            n861 = call "mDrive Send Command.vi"("error in (no error)"=w1530, "Extra"="VM", "Command"=T2."Print Parameter", "VISA resource name"=w1532) -> ("error out"=w1521:errorcluster, "read buffer"=w1528:string, "VISA resource name out"=w1522:refnum<visa-resource-name>)  [unwired: 3 in]
            n862 = call "Time Delay6"("error in (no error)"=w1521) -> ("error out"=w1520:errorcluster)  [unwired: 10 in]
            n863 = Decimal String To Number(string=w1528, offset=0) -> (number=w1531:i32)  [unwired: 1 in, 1 out]
            n864 = property on="Y velocity PV step/sec" class="DigNum (strict)"("Val(Sgnl)"=w1531) -> ()  [unwired: 2 in, 2 out]
          }
          frame #1 {
            n865 = property on="Y Scan" class="Bool (strict)"("Val(Sgnl)"=TRUE ("Slew Ready 2")) -> ()  [unwired: 2 in, 2 out]
            n866 = property on="Scan Go" class="Bool"("DisabledEnum"=T1."Enabled" ("Disabled")) -> ()  [unwired: 2 in, 2 out]
            n867 = property on="Scan Cancel" class="Bool"("DisabledEnum"=T1."Enabled" ("Disabled")) -> ()  [unwired: 2 in, 2 out]
            n868 = property on="Y Scan Length SP steps" class="DigNum (strict)"("DisabledEnum"=T1."Disabled and Grayed Out" ("Disabled")) -> ()  [unwired: 2 in, 2 out]
            n869 = property on="Y Scan Velocity SP steps/sec" class="DigNum (strict)"("DisabledEnum"=T1."Disabled and Grayed Out" ("Disabled")) -> ()  [unwired: 2 in, 2 out]
          }
          frame #2 {
            n870 = property on="Y Go" class="Bool"("DisabledEnum"=T1."Disabled and Grayed Out" ("Disabled")) -> ()  [unwired: 2 in, 2 out]
          }
        }
      }
      event #18 {
        n871 = event-data() -> ()  [unwired: 1 in, 7 out]
        n872 = flat-sequence {
          tunnel: [w1558] -> w1550
          tunnel: [w1556] -> w1549
          tunnel: w1546 -> [w1552]
          tunnel: w1545 -> [w1551]
          tunnel: w1550 -> [w1573]
          tunnel: w1549 -> [w1572]
          tunnel: [w1573] -> w1548
          tunnel: [w1572] -> w1547
          tunnel: [w1575] -> w1544
          tunnel: [w1576] -> w1543
          tunnel: w1548 -> [w1576]
          tunnel: w1547 -> [w1575]
          frame #0 {
            # "VELOCITY"
            n873 = property on="Z Scan Velocity SP steps/sec" class="DigNum (strict)"() -> ("Value"=w1559:i32)  [unwired: 2 in, 2 out]
            n874 = Number To Decimal String(number=w1559) -> (decimal integer string=w1560:string)  [unwired: 1 in]
            n875 = call "mDrive Send Command.vi"("error in (no error)"=w1551, "Extra"=w1560, "Command"=T2."Max Velocity", "VISA resource name"=w1552) -> ("error out"=w1561:errorcluster, "VISA resource name out"=w1566:refnum<visa-resource-name>)  [unwired: 3 in, 1 out]
            n876 = call "Time Delay24"("error in (no error)"=w1561) -> ("error out"=w1564:errorcluster)  [unwired: 10 in]
            n877 = call "mDrive Send Command.vi"("error in (no error)"=w1564, "Extra"="VM", "Command"=T2."Print Parameter", "VISA resource name"=w1566) -> ("error out"=w1557:errorcluster, "read buffer"=w1562:string, "VISA resource name out"=w1558:refnum<visa-resource-name>)  [unwired: 3 in]
            n878 = call "Time Delay25"("error in (no error)"=w1557) -> ("error out"=w1556:errorcluster)  [unwired: 10 in]
            n879 = Decimal String To Number(string=w1562, offset=0) -> (number=w1565:i32)  [unwired: 1 in, 1 out]
            n880 = property on="Z  velocity PV step/sec" class="DigNum (strict)"("Val(Sgnl)"=w1565) -> ()  [unwired: 2 in, 2 out]
          }
          frame #1 {
            n881 = property on="Z Scan" class="Bool (strict)"("Val(Sgnl)"=TRUE ("Slew Ready 2")) -> ()  [unwired: 2 in, 2 out]
            n882 = property on="Scan Go" class="Bool"("DisabledEnum"=T1."Enabled" ("Disabled")) -> ()  [unwired: 2 in, 2 out]
            n883 = property on="Scan Cancel" class="Bool"("DisabledEnum"=T1."Enabled" ("Disabled")) -> ()  [unwired: 2 in, 2 out]
            n884 = property on="Z Scan Length SP steps" class="DigNum (strict)"("DisabledEnum"=T1."Disabled and Grayed Out" ("Disabled")) -> ()  [unwired: 2 in, 2 out]
            n885 = property on="Z Scan Velocity SP steps/sec" class="DigNum (strict)"("DisabledEnum"=T1."Disabled and Grayed Out" ("Disabled")) -> ()  [unwired: 2 in, 2 out]
          }
          frame #2 {
            n886 = property on="Z Go" class="Bool"("DisabledEnum"=T1."Disabled and Grayed Out" ("Disabled")) -> ()  [unwired: 2 in, 2 out]
          }
        }
      }
      event #19 {
        n887 = event-data() -> ()  [unwired: 1 in, 7 out]
        n888 = flat-sequence {
          tunnel: [w1592] -> w1584
          tunnel: [w1590] -> w1583
          tunnel: w1580 -> [w1586]
          tunnel: w1579 -> [w1585]
          tunnel: w1584 -> [w1607]
          tunnel: w1583 -> [w1606]
          tunnel: [w1607] -> w1582
          tunnel: [w1606] -> w1581
          tunnel: [w1609] -> w1577
          tunnel: [w1610] -> w1578
          tunnel: w1582 -> [w1610]
          tunnel: w1581 -> [w1609]
          frame #0 {
            # "VELOCITY"
            n889 = property on="R Scan Velocity SP steps/sec" class="DigNum (strict)"() -> ("Value"=w1593:i32)  [unwired: 2 in, 2 out]
            n890 = Number To Decimal String(number=w1593) -> (decimal integer string=w1594:string)  [unwired: 1 in]
            n891 = call "mDrive Send Command.vi"("error in (no error)"=w1585, "Extra"=w1594, "Command"=T2."Max Velocity", "VISA resource name"=w1586) -> ("error out"=w1595:errorcluster, "VISA resource name out"=w1600:refnum<visa-resource-name>)  [unwired: 3 in, 1 out]
            n892 = call "Time Delay26"("error in (no error)"=w1595) -> ("error out"=w1598:errorcluster)  [unwired: 10 in]
            n893 = call "mDrive Send Command.vi"("error in (no error)"=w1598, "Extra"="VM", "Command"=T2."Print Parameter", "VISA resource name"=w1600) -> ("error out"=w1591:errorcluster, "read buffer"=w1596:string, "VISA resource name out"=w1592:refnum<visa-resource-name>)  [unwired: 3 in]
            n894 = call "Time Delay27"("error in (no error)"=w1591) -> ("error out"=w1590:errorcluster)  [unwired: 10 in]
            n895 = Decimal String To Number(string=w1596, offset=0) -> (number=w1599:i32)  [unwired: 1 in, 1 out]
            n896 = property on="R velocity PV step/sec" class="DigNum (strict)"("Val(Sgnl)"=w1599) -> ()  [unwired: 2 in, 2 out]
          }
          frame #1 {
            n897 = property on="R Scan" class="Bool (strict)"("Val(Sgnl)"=TRUE ("Slew Ready 2")) -> ()  [unwired: 2 in, 2 out]
            n898 = property on="Scan Go" class="Bool"("DisabledEnum"=T1."Enabled" ("Disabled")) -> ()  [unwired: 2 in, 2 out]
            n899 = property on="Scan Cancel" class="Bool"("DisabledEnum"=T1."Enabled" ("Disabled")) -> ()  [unwired: 2 in, 2 out]
            n900 = property on="R Scan Length SP steps" class="DigNum (strict)"("DisabledEnum"=T1."Disabled and Grayed Out" ("Disabled")) -> ()  [unwired: 2 in, 2 out]
            n901 = property on="R Scan Velocity SP steps/sec" class="DigNum (strict)"("DisabledEnum"=T1."Disabled and Grayed Out" ("Disabled")) -> ()  [unwired: 2 in, 2 out]
          }
          frame #2 {
            n902 = property on="R Go" class="Bool"("DisabledEnum"=T1."Disabled and Grayed Out" ("Disabled")) -> ()  [unwired: 2 in, 2 out]
          }
        }
      }
      event #20 {
        n903 = event-data() -> ()  [unwired: 1 in, 4 out]
        n904 = event-data() -> ()  [unwired: 3 in, 1 out]
      }
      event #21 {
        n905 = event-data() -> ()  [unwired: 1 in, 7 out]
        n906 = flat-sequence {
          tunnel: [w1643] -> w1625
          tunnel: [w1642] -> w1624
          tunnel: w1623 -> [w1641]
          tunnel: w1622 -> [w1640]
          frame #0 {
            n907 = call "mDrive Send Command.vi"("error in (no error)"=w1640, "Command"=T2."Stop", "VISA resource name"=w1641) -> ("error out"=w1642:errorcluster, "VISA resource name out"=w1643:refnum<visa-resource-name>)  [unwired: 4 in, 1 out]
          }
        }
        n908 = flat-sequence {
          tunnel: w1629 -> [w1649]
          tunnel: w1628 -> [w1648]
          tunnel: [w1647] -> w1627
          tunnel: [w1646] -> w1626
          frame #0 {
            n909 = call "mDrive Send Command.vi"("error in (no error)"=w1648, "Command"=T2."Stop", "VISA resource name"=w1649) -> ("error out"=w1646:errorcluster, "VISA resource name out"=w1647:refnum<visa-resource-name>)  [unwired: 4 in, 1 out]
          }
        }
        n910 = flat-sequence {
          tunnel: [w1638] -> w1619
          tunnel: [w1637] -> w1618
          tunnel: w1621 -> [w1636]
          tunnel: w1620 -> [w1635]
          frame #0 {
            n911 = call "mDrive Send Command.vi"("error in (no error)"=w1635, "Command"=T2."Stop", "VISA resource name"=w1636) -> ("error out"=w1637:errorcluster, "VISA resource name out"=w1638:refnum<visa-resource-name>)  [unwired: 4 in, 1 out]
          }
        }
        n912 = flat-sequence {
          tunnel: w1617 -> [w1634]
          tunnel: w1616 -> [w1633]
          tunnel: [w1632] -> w1615
          tunnel: [w1630] -> _
          tunnel: [w1630] -> w1614
          frame #0 {
            n913 = call "mDrive Send Command.vi"("error in (no error)"=w1633, "Command"=T2."Stop", "VISA resource name"=w1634) -> ("error out"=w1630:errorcluster, "VISA resource name out"=w1632:refnum<visa-resource-name>)  [unwired: 4 in, 1 out]
          }
        }
      }
      event #22 {
        n914 = event-data() -> ()  [unwired: 1 in, 7 out]
        n915 = flat-sequence {
          tunnel: w1665 -> [w1704]
          tunnel: w1664 -> [w1703]
          tunnel: [w1706] -> w1667
          tunnel: [w1705] -> w1666
          tunnel: [w1713] -> w1662
          tunnel: [w1714] -> w1663
          tunnel: w1667 -> [w1714]
          tunnel: w1666 -> [w1713]
          frame #0 {
            n916 = call "mDrive Send Command.vi"("error in (no error)"=w1703, "Command"=T2."Stop", "VISA resource name"=w1704) -> ("error out"=w1705:errorcluster, "VISA resource name out"=w1706:refnum<visa-resource-name>)  [unwired: 4 in, 1 out]
          }
          frame #1 {
            n917 = property on="X Scan" class="Bool (strict)"("Value"=FALSE ("Slew Ready")) -> ()  [unwired: 2 in, 2 out]
            n918 = property on="X Scan set" class="Bool"("DisabledEnum"=T1."Enabled" ("Disabled")) -> ()  [unwired: 2 in, 2 out]
            n919 = property on="X Scan Velocity SP steps/sec" class="DigNum (strict)"("DisabledEnum"=T1."Enabled" ("Disabled")) -> ()  [unwired: 2 in, 2 out]
            n920 = property on="X Scan Length SP steps" class="DigNum (strict)"("DisabledEnum"=T1."Enabled" ("Disabled")) -> ()  [unwired: 2 in, 2 out]
            n921 = property on="X Go" class="Bool"("DisabledEnum"=T1."Enabled" ("Disabled")) -> ()  [unwired: 2 in, 2 out]
            n922 = property on="X Scan OK" class="Bool"("DisabledEnum"=T1."Enabled" ("Disabled")) -> ()  [unwired: 2 in, 2 out]
          }
        }
        n923 = flat-sequence {
          tunnel: w1673 -> [w1717]
          tunnel: w1672 -> [w1716]
          tunnel: [w1719] -> w1669
          tunnel: [w1718] -> w1668
          tunnel: [w1726] -> w1674
          tunnel: [w1727] -> w1675
          tunnel: w1669 -> [w1727]
          tunnel: w1668 -> [w1726]
          frame #0 {
            n924 = call "mDrive Send Command.vi"("error in (no error)"=w1716, "Command"=T2."Stop", "VISA resource name"=w1717) -> ("error out"=w1718:errorcluster, "VISA resource name out"=w1719:refnum<visa-resource-name>)  [unwired: 4 in, 1 out]
          }
          frame #1 {
            n925 = property on="Y Scan" class="Bool (strict)"("Value"=FALSE ("Slew Ready")) -> ()  [unwired: 2 in, 2 out]
            n926 = property on="Y Scan Velocity SP steps/sec" class="DigNum (strict)"("DisabledEnum"=T1."Enabled" ("Disabled")) -> ()  [unwired: 2 in, 2 out]
            n927 = property on="Y Go" class="Bool"("DisabledEnum"=T1."Enabled" ("Disabled")) -> ()  [unwired: 2 in, 2 out]
            n928 = property on="Y Scan OK" class="Bool"("DisabledEnum"=T1."Enabled" ("Disabled")) -> ()  [unwired: 2 in, 2 out]
            n929 = property on="Y Scan Length SP steps" class="DigNum (strict)"("DisabledEnum"=T1."Enabled" ("Disabled")) -> ()  [unwired: 2 in, 2 out]
            n930 = property on="Y Scan set" class="Bool"("DisabledEnum"=T1."Enabled" ("Disabled")) -> ()  [unwired: 2 in, 2 out]
          }
        }
        n931 = flat-sequence {
          tunnel: [w1693] -> w1661
          tunnel: [w1692] -> w1660
          tunnel: w1659 -> [w1690]
          tunnel: w1658 -> [w1689]
          tunnel: [w1700] -> w1656
          tunnel: [w1701] -> w1657
          tunnel: w1661 -> [w1701]
          tunnel: w1660 -> [w1700]
          frame #0 {
            n932 = call "mDrive Send Command.vi"("error in (no error)"=w1689, "Command"=T2."Stop", "VISA resource name"=w1690) -> ("error out"=w1692:errorcluster, "VISA resource name out"=w1693:refnum<visa-resource-name>)  [unwired: 4 in, 1 out]
          }
          frame #1 {
            n933 = property on="Z Scan" class="Bool (strict)"("Value"=FALSE ("Slew Ready")) -> ()  [unwired: 2 in, 2 out]
            n934 = property on="Z Scan set" class="Bool"("DisabledEnum"=T1."Enabled" ("Disabled")) -> ()  [unwired: 2 in, 2 out]
            n935 = property on="Z Scan Velocity SP steps/sec" class="DigNum (strict)"("DisabledEnum"=T1."Enabled" ("Disabled")) -> ()  [unwired: 2 in, 2 out]
            n936 = property on="Z Scan Length SP steps" class="DigNum (strict)"("DisabledEnum"=T1."Enabled" ("Disabled")) -> ()  [unwired: 2 in, 2 out]
            n937 = property on="Z Go" class="Bool"("DisabledEnum"=T1."Enabled" ("Disabled")) -> ()  [unwired: 2 in, 2 out]
            n938 = property on="Z Scan OK" class="Bool"("DisabledEnum"=T1."Enabled" ("Disabled")) -> ()  [unwired: 2 in, 2 out]
          }
        }
        n939 = flat-sequence {
          tunnel: [w1680] -> w1655
          tunnel: [w1679] -> w1654
          tunnel: w1653 -> [w1677]
          tunnel: w1652 -> [w1676]
          tunnel: [w1687] -> w1650
          tunnel: [w1688] -> w1651
          tunnel: w1655 -> [w1688]
          tunnel: w1654 -> [w1687]
          frame #0 {
            n940 = call "mDrive Send Command.vi"("error in (no error)"=w1676, "Command"=T2."Stop", "VISA resource name"=w1677) -> ("error out"=w1679:errorcluster, "VISA resource name out"=w1680:refnum<visa-resource-name>)  [unwired: 4 in, 1 out]
          }
          frame #1 {
            n941 = property on="R Scan" class="Bool (strict)"("Value"=FALSE ("Slew Ready")) -> ()  [unwired: 2 in, 2 out]
            n942 = property on="R Scan OK" class="Bool"("DisabledEnum"=T1."Enabled" ("Disabled")) -> ()  [unwired: 2 in, 2 out]
            n943 = property on="R Scan Length SP steps" class="DigNum (strict)"("DisabledEnum"=T1."Enabled" ("Disabled")) -> ()  [unwired: 2 in, 2 out]
            n944 = property on="R Scan set" class="Bool"("DisabledEnum"=T1."Enabled" ("Disabled")) -> ()  [unwired: 2 in, 2 out]
            n945 = property on="R Scan Velocity SP steps/sec" class="DigNum (strict)"("DisabledEnum"=T1."Enabled" ("Disabled")) -> ()  [unwired: 2 in, 2 out]
            n946 = property on="R Go" class="Bool"("DisabledEnum"=T1."Enabled" ("Disabled")) -> ()  [unwired: 2 in, 2 out]
          }
        }
        n947 = property on="Scan Go" class="Bool"("DisabledEnum"=T1."Disabled and Grayed Out" ("Disabled")) -> ()  [unwired: 2 in, 2 out]
        n948 = property on="Scan Cancel" class="Bool"("DisabledEnum"=T1."Disabled and Grayed Out" ("Disabled")) -> ()  [unwired: 2 in, 2 out]
      }
      event #23 {
        n949 = event-data() -> ()  [unwired: 1 in, 7 out]
        n950 = flat-sequence {
          tunnel: [w1807] -> w1791
          tunnel: [w1805] -> w1784
          tunnel: [w1806] -> w1781
          tunnel: [w1800] -> w1780
          tunnel: [w1804] -> w1779
          tunnel: [w1803] -> w1778
          tunnel: [w1802] -> w1777
          tunnel: [w1801] -> w1776
          tunnel: w1755 -> [w1799]
          tunnel: [w1799] -> w1754
          tunnel: w1753 -> [w1798]
          tunnel: [w1798] -> w1752
          tunnel: w1751 -> [w1797]
          tunnel: [w1797] -> w1750
          tunnel: w1749 -> [w1796]
          tunnel: [w1796] -> w1748
          tunnel: w1747 -> [w1795]
          tunnel: [w1795] -> w1746
          tunnel: w1745 -> [w1794]
          tunnel: [w1794] -> w1744
          tunnel: [w1793] -> w1743
          tunnel: w1742 -> [w1793]
          tunnel: [w1792] -> w1741
          tunnel: w1740 -> [w1792]
          tunnel: [w1859] -> w1788
          tunnel: [w1858] -> w1786
          tunnel: w1791 -> [w1857]
          tunnel: w1784 -> [w1856]
          tunnel: [w1856] -> w1782
          tunnel: w1781 -> [w1855]
          tunnel: w1780 -> [w1844]
          tunnel: w1779 -> [w1854]
          tunnel: w1778 -> [w1850]
          tunnel: w1777 -> [w1847]
          tunnel: w1776 -> [w1853]
          tunnel: [w1852] -> w1774
          tunnel: [w1851] -> w1772
          tunnel: [w1850] -> w1769
          tunnel: [w1849] -> w1767
          tunnel: [w1848] -> w1765
          tunnel: [w1847] -> w1763
          tunnel: [w1846] -> w1761
          tunnel: [w1845] -> w1759
          tunnel: [w1844] -> w1758
          tunnel: w1754 -> [w1843]
          tunnel: w1752 -> [w1842]
          tunnel: w1750 -> [w1841]
          tunnel: w1748 -> [w1840]
          tunnel: w1746 -> [w1839]
          tunnel: w1744 -> [w1838]
          tunnel: w1743 -> [w1837]
          tunnel: w1741 -> [w1836]
          tunnel: w1788 -> [w1900]
          tunnel: [w1900] -> w1787
          tunnel: w1786 -> [w1899]
          tunnel: [w1899] -> w1785
          tunnel: [w1897] -> w1783
          tunnel: w1782 -> [w1897]
          tunnel: [w1896] -> w1775
          tunnel: w1774 -> [w1896]
          tunnel: [w1895] -> w1773
          tunnel: w1772 -> [w1895]
          tunnel: [w1894] -> w1771
          tunnel: [w1893] -> w1770
          tunnel: w1769 -> [w1893]
          tunnel: [w1892] -> w1768
          tunnel: w1767 -> [w1892]
          tunnel: [w1891] -> w1766
          tunnel: w1765 -> [w1891]
          tunnel: [w1890] -> w1764
          tunnel: w1763 -> [w1890]
          tunnel: [w1889] -> w1762
          tunnel: w1761 -> [w1889]
          tunnel: [w1888] -> w1760
          tunnel: w1759 -> [w1888]
          tunnel: w1758 -> [w1894]
          tunnel: w1787 -> [w1920]
          tunnel: [w1918] -> w1790
          tunnel: w1785 -> [w1919]
          tunnel: [w1917] -> w1789
          tunnel: w1783 -> [w1916]
          tunnel: w1775 -> [w1915]
          tunnel: w1773 -> [w1914]
          tunnel: w1771 -> [w1913]
          tunnel: w1770 -> [w1912]
          tunnel: w1768 -> [w1911]
          tunnel: w1766 -> [w1910]
          tunnel: w1764 -> [w1909]
          tunnel: w1762 -> [w1908]
          tunnel: w1760 -> [w1907]
          tunnel: [w1906] -> w1757
          tunnel: [w1905] -> w1756
          tunnel: [w1904] -> w1735
          tunnel: [w1903] -> w1732
          tunnel: [w1902] -> w1730
          tunnel: [w1901] -> w1728
          tunnel: w1790 -> [w1978]
          tunnel: w1789 -> [w1977]
          tunnel: [w1978] -> w1739
          tunnel: [w1977] -> w1738
          tunnel: [w1971] -> w1737
          tunnel: w1757 -> [w1971]
          tunnel: [w1970] -> w1736
          tunnel: w1756 -> [w1970]
          tunnel: w1735 -> [w1960]
          tunnel: [w1960] -> w1734
          tunnel: [w1959] -> w1733
          tunnel: w1732 -> [w1959]
          tunnel: [w1958] -> w1731
          tunnel: w1730 -> [w1958]
          tunnel: [w1957] -> w1729
          tunnel: w1728 -> [w1957]
          frame #0 {
            n951 = property on="X Scan" class="Bool (strict)"() -> ("Value"=w1800:bool)  [unwired: 2 in, 2 out]
            n952 = property on="Y Scan" class="Bool (strict)"() -> ("Value"=w1805:bool)  [unwired: 2 in, 2 out]
            n953 = property on="Z Scan" class="Bool (strict)"() -> ("Value"=w1802:bool)  [unwired: 2 in, 2 out]
            n954 = property on="R Scan" class="Bool (strict)"() -> ("Value"=w1803:bool)  [unwired: 2 in, 2 out]
            n955 = case shown="True" w1800 {
              tunnel: ["" w1823] -> w1806
              frame #0 {
              }
              frame #1 {
                n956 = property on="X Scan Length SP steps" class="DigNum (strict)"() -> ("Value"=w1828:i32)  [unwired: 2 in, 2 out]
                n957 = Number To Decimal String(number=w1828) -> (decimal integer string=w1825:string)  [unwired: 1 in]
                n958 = call <vilib>:"Space Constant.vi"() -> ("String"=w1826:string)
                n959 = Concatenate Strings("MR", w1826, w1825, "\r") -> (w1823:string)
              }
            }
            n960 = case shown="True" w1805 {
              tunnel: ["" w1830] -> w1807
              frame #0 {
              }
              frame #1 {
                n961 = property on="Y Scan Length SP steps" class="DigNum (strict)"() -> ("Value"=w1835:i32)  [unwired: 2 in, 2 out]
                n962 = Number To Decimal String(number=w1835) -> (decimal integer string=w1832:string)  [unwired: 1 in]
                n963 = call <vilib>:"Space Constant.vi"() -> ("String"=w1833:string)
                n964 = Concatenate Strings("MR", w1833, w1832, "\r") -> (w1830:string)
              }
            }
            n965 = case shown="True" w1802 {
              tunnel: ["" w1816] -> w1804
              frame #0 {
              }
              frame #1 {
                n966 = property on="Z Scan Length SP steps" class="DigNum (strict)"() -> ("Value"=w1821:i32)  [unwired: 2 in, 2 out]
                n967 = Number To Decimal String(number=w1821) -> (decimal integer string=w1818:string)  [unwired: 1 in]
                n968 = call <vilib>:"Space Constant.vi"() -> ("String"=w1819:string)
                n969 = Concatenate Strings("MR", w1819, w1818, "\r") -> (w1816:string)
              }
            }
            n970 = case shown="True" w1803 {
              tunnel: ["" w1809] -> w1801
              frame #0 {
              }
              frame #1 {
                n971 = property on="R Scan Length SP steps" class="DigNum (strict)"() -> ("Value"=w1814:i32)  [unwired: 2 in, 2 out]
                n972 = Number To Decimal String(number=w1814) -> (decimal integer string=w1811:string)  [unwired: 1 in]
                n973 = call <vilib>:"Space Constant.vi"() -> ("String"=w1812:string)
                n974 = Concatenate Strings("MR", w1812, w1811, "\r") -> (w1809:string)
              }
            }
          }
          frame #1 {
            n975 = case shown="False" w1844 {
              tunnel: [w1875 w1880] -> w1852
              tunnel: [w1874 w1879] -> w1851
              tunnel: w1855 -> [_ w1878]
              tunnel: w1843 -> [w1875 w1877]
              tunnel: w1842 -> [w1874 w1876]
              frame #0 {
              }
              frame #1 {
                n976 = VISA Write(VISA resource name=w1877, write buffer=w1878, error in (no error)=w1876) -> (VISA resource name out=w1880:refnum<visa-resource-name>, error out=w1879:errorcluster)  [unwired: 1 out]
              }
            }
            n977 = case shown="False" w1856 {
              tunnel: [w1882 w1887] -> w1859
              tunnel: [w1881 w1886] -> w1858
              tunnel: w1857 -> [_ w1885]
              tunnel: w1841 -> [w1882 w1884]
              tunnel: w1840 -> [w1881 w1883]
              frame #0 {
              }
              frame #1 {
                n978 = VISA Write(VISA resource name=w1884, write buffer=w1885, error in (no error)=w1883) -> (VISA resource name out=w1887:refnum<visa-resource-name>, error out=w1886:errorcluster)  [unwired: 1 out]
              }
            }
            n979 = case shown="False" w1847 {
              tunnel: [w1868 w1873] -> w1846
              tunnel: [w1867 w1872] -> w1845
              tunnel: w1854 -> [_ w1871]
              tunnel: w1839 -> [w1868 w1870]
              tunnel: w1838 -> [w1867 w1869]
              frame #0 {
              }
              frame #1 {
                n980 = VISA Write(VISA resource name=w1870, write buffer=w1871, error in (no error)=w1869) -> (VISA resource name out=w1873:refnum<visa-resource-name>, error out=w1872:errorcluster)  [unwired: 1 out]
              }
            }
            n981 = case shown="False" w1850 {
              tunnel: [w1861 w1866] -> w1849
              tunnel: [w1860 w1865] -> w1848
              tunnel: w1853 -> [_ w1864]
              tunnel: w1837 -> [w1861 w1863]
              tunnel: w1836 -> [w1860 w1862]
              frame #0 {
              }
              frame #1 {
                n982 = VISA Write(VISA resource name=w1863, write buffer=w1864, error in (no error)=w1862) -> (VISA resource name out=w1866:refnum<visa-resource-name>, error out=w1865:errorcluster)  [unwired: 1 out]
              }
            }
          }
          frame #2 {
            n983 = call "Time Delay7"("Delay Time (s)"=0.1) -> ()  [unwired: 10 in, 1 out]
          }
          frame #3 {
            n984 = case shown="True" w1913 {
              tunnel: w1915 -> [w1940 w1944]
              tunnel: w1914 -> [w1939 w1943]
              tunnel: [w1940 w1942] -> w1902
              tunnel: [w1939 w1941] -> w1901
              frame #0 {
              }
              frame #1 {
                n985 = property class="Instr"(reference=w1944, error in=w1943) -> (reference out=w1946:refnum<visa-resource-name>, error out=w1945:errorcluster, "Serial Settings:Number of Bytes at Serial Port"=w1947:u32)
                n986 = VISA Read(VISA resource name=w1946, byte count=w1947, error in (no error)=w1945) -> (VISA resource name out=w1942:refnum<visa-resource-name>, error out=w1941:errorcluster)  [unwired: 2 out]
              }
            }
            n987 = case shown="True" w1916 {
              tunnel: w1920 -> [w1949 w1953]
              tunnel: w1919 -> [w1948 w1952]
              tunnel: [w1949 w1951] -> w1918
              tunnel: [w1948 w1950] -> w1917
              frame #0 {
              }
              frame #1 {
                n988 = property class="Instr"(reference=w1953, error in=w1952) -> (reference out=w1955:refnum<visa-resource-name>, error out=w1954:errorcluster, "Serial Settings:Number of Bytes at Serial Port"=w1956:u32)
                n989 = VISA Read(VISA resource name=w1955, byte count=w1956, error in (no error)=w1954) -> (VISA resource name out=w1951:refnum<visa-resource-name>, error out=w1950:errorcluster)  [unwired: 2 out]
              }
            }
            n990 = case shown="True" w1909 {
              tunnel: w1908 -> [w1922 w1926]
              tunnel: w1907 -> [w1921 w1925]
              tunnel: [w1922 w1924] -> w1906
              tunnel: [w1921 w1923] -> w1905
              frame #0 {
              }
              frame #1 {
                n991 = property class="Instr"(reference=w1926, error in=w1925) -> (reference out=w1928:refnum<visa-resource-name>, error out=w1927:errorcluster, "Serial Settings:Number of Bytes at Serial Port"=w1929:u32)
                n992 = VISA Read(VISA resource name=w1928, byte count=w1929, error in (no error)=w1927) -> (VISA resource name out=w1924:refnum<visa-resource-name>, error out=w1923:errorcluster)  [unwired: 2 out]
              }
            }
            n993 = case shown="True" w1912 {
              tunnel: w1911 -> [w1931 w1935]
              tunnel: w1910 -> [w1930 w1934]
              tunnel: [w1931 w1933] -> w1904
              tunnel: [w1930 w1932] -> w1903
              frame #0 {
              }
              frame #1 {
                n994 = property class="Instr"(reference=w1935, error in=w1934) -> (reference out=w1937:refnum<visa-resource-name>, error out=w1936:errorcluster, "Serial Settings:Number of Bytes at Serial Port"=w1938:u32)
                n995 = VISA Read(VISA resource name=w1937, byte count=w1938, error in (no error)=w1936) -> (VISA resource name out=w1933:refnum<visa-resource-name>, error out=w1932:errorcluster)  [unwired: 2 out]
              }
            }
          }
          frame #4 {
            n996 = property on="R Scan" class="Bool (strict)"("Val(Sgnl)"=FALSE ("Slew Ready 2")) -> ()  [unwired: 2 in, 2 out]
            n997 = property on="X Scan" class="Bool (strict)"("Val(Sgnl)"=FALSE ("Slew Ready 2")) -> ()  [unwired: 2 in, 2 out]
            n998 = property on="Z Scan" class="Bool (strict)"("Val(Sgnl)"=FALSE ("Slew Ready 2")) -> ()  [unwired: 2 in, 2 out]
            n999 = property on="Y Scan Length SP steps" class="DigNum (strict)"("DisabledEnum"=T1."Enabled" ("Disabled")) -> ()  [unwired: 2 in, 2 out]
            n1000 = property on="Scan Go" class="Bool"("DisabledEnum"=T1."Disabled and Grayed Out" ("Disabled")) -> ()  [unwired: 2 in, 2 out]
            n1001 = property on="Y Scan" class="Bool (strict)"("Val(Sgnl)"=FALSE ("Slew Ready 2")) -> ()  [unwired: 2 in, 2 out]
            n1002 = property on="Scan Cancel" class="Bool"("DisabledEnum"=T1."Disabled and Grayed Out" ("Disabled")) -> ()  [unwired: 2 in, 2 out]
            n1003 = property on="Y Scan Selocity SP steps/sec" class="DigNum (strict)"("DisabledEnum"=T1."Enabled" ("Disabled")) -> ()  [unwired: 2 in, 2 out]
            n1004 = property on="R Scan Length SP steps" class="DigNum (strict)"("DisabledEnum"=T1."Enabled" ("Disabled")) -> ()  [unwired: 2 in, 2 out]
            n1005 = property on="X Scan Length SP steps" class="DigNum (strict)"("DisabledEnum"=T1."Enabled" ("Disabled")) -> ()  [unwired: 2 in, 2 out]
            n1006 = property on="Z Scan Length SP steps" class="DigNum (strict)"("DisabledEnum"=T1."Enabled" ("Disabled")) -> ()  [unwired: 2 in, 2 out]
            n1007 = property on="X Scan Velocity SP steps/sec" class="DigNum (strict)"("DisabledEnum"=T1."Enabled" ("Disabled")) -> ()  [unwired: 2 in, 2 out]
            n1008 = property on="R Scan Velocity SP steps/sec" class="DigNum (strict)"("DisabledEnum"=T1."Enabled" ("Disabled")) -> ()  [unwired: 2 in, 2 out]
            n1009 = property on="Z Scan Velocity SP steps/sec" class="DigNum (strict)"("DisabledEnum"=T1."Enabled" ("Disabled")) -> ()  [unwired: 2 in, 2 out]
          }
        }
      }
      event #24 {
        n1010 = event-data() -> ()  [unwired: 1 in, 7 out]
        n1011 = flat-sequence {
          tunnel: [w2009] -> w1988
          tunnel: w1989 -> [w2012]
          tunnel: [w2011] -> w1987
          tunnel: w1990 -> [w2010]
          frame #0 {
            n1012 = property on="Reset X Motor Steps" class="DigNum (strict)"() -> ("Value"=w2013:i32)  [unwired: 2 in, 2 out]
            n1013 = Number To Decimal String(number=w2013) -> (decimal integer string=w2014:string)  [unwired: 1 in]
            n1014 = call "mDrive Send Command.vi"("error in (no error)"=w2012, "Extra"=w2014, "Command"=T2."Set Current Position", "VISA resource name"=w2010) -> ("error out"=w2011:errorcluster, "VISA resource name out"=w2009:refnum<visa-resource-name>)  [unwired: 3 in, 1 out]
          }
        }
        n1015 = flat-sequence {
          tunnel: w1994 -> [w2019]
          tunnel: w1993 -> [w2018]
          tunnel: [w2017] -> w1992
          tunnel: [w2016] -> w1991
          frame #0 {
            n1016 = property on="Reset Y Motor Steps" class="DigNum (strict)"() -> ("Value"=w2020:i32)  [unwired: 2 in, 2 out]
            n1017 = Number To Decimal String(number=w2020) -> (decimal integer string=w2021:string)  [unwired: 1 in]
            n1018 = call "mDrive Send Command.vi"("error in (no error)"=w2018, "Extra"=w2021, "Command"=T2."Set Current Position", "VISA resource name"=w2019) -> ("error out"=w2016:errorcluster, "VISA resource name out"=w2017:refnum<visa-resource-name>)  [unwired: 3 in, 1 out]
          }
        }
        n1019 = flat-sequence {
          tunnel: [w1996] -> w1982
          tunnel: [w1998] -> w1981
          tunnel: w1984 -> [w1997]
          tunnel: w1983 -> [w1995]
          frame #0 {
            n1020 = property on="Reset R Motor Steps" class="DigNum (strict)"() -> ("Value"=w1999:i32)  [unwired: 2 in, 2 out]
            n1021 = Number To Decimal String(number=w1999) -> (decimal integer string=w2000:string)  [unwired: 1 in]
            n1022 = call "mDrive Send Command.vi"("error in (no error)"=w1995, "Extra"=w2000, "Command"=T2."Set Current Position", "VISA resource name"=w1997) -> ("error out"=w1998:errorcluster, "VISA resource name out"=w1996:refnum<visa-resource-name>)  [unwired: 3 in, 1 out]
          }
        }
        n1023 = flat-sequence {
          tunnel: [w2005] -> w1980
          tunnel: [w2004] -> w1979
          tunnel: w1986 -> [w2003]
          tunnel: w1985 -> [w2002]
          frame #0 {
            n1024 = property on="Reset Z Motor Steps" class="DigNum (strict)"() -> ("Value"=w2006:i32)  [unwired: 2 in, 2 out]
            n1025 = Number To Decimal String(number=w2006) -> (decimal integer string=w2007:string)  [unwired: 1 in]
            n1026 = call "mDrive Send Command.vi"("error in (no error)"=w2002, "Extra"=w2007, "Command"=T2."Set Current Position", "VISA resource name"=w2003) -> ("error out"=w2004:errorcluster, "VISA resource name out"=w2005:refnum<visa-resource-name>)  [unwired: 3 in, 1 out]
          }
        }
      }
    }
  }
  n1027 = flat-sequence {
    tunnel: w60 -> [w2027]
    tunnel: w59 -> [w2024]
    frame #0 {
      n1028 = call "mDrive Send Command.vi"("error in (no error)"=w2024, "Command"=T2."Stop", "VISA resource name"=w2027) -> ("error out"=w2025:errorcluster, "VISA resource name out"=w2026:refnum<visa-resource-name>)  [unwired: 4 in, 1 out]
      n1029 = VISA Close(VISA resource name=w2026, error in (no error)=w2025) -> ()  [unwired: 1 out]
    }
  }
  n1030 = flat-sequence {
    tunnel: w87 -> [w2032]
    tunnel: w86 -> [w2029]
    frame #0 {
      n1031 = call "mDrive Send Command.vi"("error in (no error)"=w2029, "Command"=T2."Stop", "VISA resource name"=w2032) -> ("error out"=w2030:errorcluster, "VISA resource name out"=w2031:refnum<visa-resource-name>)  [unwired: 4 in, 1 out]
      n1032 = VISA Close(VISA resource name=w2031, error in (no error)=w2030) -> ()  [unwired: 1 out]
    }
  }
  n1033 = flat-sequence {
    tunnel: w14 -> [w2037]
    tunnel: w13 -> [w2034]
    frame #0 {
      n1034 = call "mDrive Send Command.vi"("error in (no error)"=w2034, "Command"=T2."Stop", "VISA resource name"=w2037) -> ("error out"=w2035:errorcluster, "VISA resource name out"=w2036:refnum<visa-resource-name>)  [unwired: 4 in, 1 out]
      n1035 = VISA Close(VISA resource name=w2036, error in (no error)=w2035) -> ()  [unwired: 1 out]
    }
  }
  n1036 = flat-sequence {
    tunnel: w10 -> [w2042]
    tunnel: w9 -> [w2039]
    frame #0 {
      n1037 = call "mDrive Send Command.vi"("error in (no error)"=w2039, "Command"=T2."Stop", "VISA resource name"=w2042) -> ("error out"=w2040:errorcluster, "VISA resource name out"=w2041:refnum<visa-resource-name>)  [unwired: 4 in, 1 out]
      n1038 = VISA Close(VISA resource name=w2041, error in (no error)=w2040) -> ()  [unwired: 1 out]
    }
  }
  "Y COM PORT" <- w90
  "X COM PORT" <- w65
  "Z COM PORT" <- w52
  "R COM PORT" <- w19
